vi "FIB MAIN (6400d-132016-w's conflicted copy 2019-02-25).vi"() -> ()   [LabVIEW 2018]
uses:
  <vilib>/userdefined/High Color/IMAQdx.ctl
  STAGE POSITION.ctl
  Original FIB Source/CENTER STIGMATOR.ctl
  FIB EVENTS.ctl
  FIB CAMERA EVENTS.ctl
  <vilib>/vision/driver/IMAQdx.llb/IMAQdx Buffer Number Mode.ctl
  <vilib>/vision/driver/IMAQdx.llb/IMAQdx Camera Control Mode.ctl
  <vilib>/Instr/_visa.llb/VISA Flush IO Buffer Mask.ctl
  <vilib>/Utility/error.llb/whitespace.ctl
  Mikrodaq/HYMOD MAIA/ddd.ctl
  FIB STAGE EVENTS.ctl
  <vilib>/Instr/_visa.llb/VISA Configure Serial Port (Instr).vi
  <vilib>/vision/driver/NI_Vision_Acquisition_Software.lvlib
  <resource>/objmgr/imaqdx.rc
  <vilib>/vision/NI_Vision_Development_Module.lvlib
  <vilib>/Utility/Variable/NI_VariableUtilities.lvlib
panel:
  out "PREVIOUS GUN SETTINGS":T1 {"ION CURRENT" min=0 max=3e-05 step=1e-07; "SUPPRESSOR" min=0 max=30000 step=250; "EXTRACTOR" min=0 max=30000 step=250; "BEAM ENERGY" min=0 max=30000 step=1000}
  out "size(s) 5":i32
  in  "ENABLE APERTURES":bool
  in  "ENABLE ORSAY":bool=TRUE
  in  "ENABLE CAMERA":bool
  out "size(s) 4":i32
  in  "Tab Control 4":enum32{"COMMANDS", "HV RAMPS"}(tab)
  in  "1V ENERGY RAMP":bool
  out "TEST OUTPUT":string
  in  "TEST COMMAND":bool
  in  "TEST COMMAND":string
  out "SERIAL \nRESPONSE":string[](array[string])
  out "WARNING":string
  out "PROCESS":string
  out "PROCESSES":string[](array[string])
  out "BEAM RAMP":dbl[unit][](graph)
  out "EXTRACTOR RAMP":dbl[unit][](graph)
  out "SUPPRESSOR RAMP":dbl[unit][](graph)
  in  "Tab Control 3":T2(tab)
  in  "E&B":T3 {"ELECTRIC FIELD" min=0 max=20 step=0.1 scale=0.0..2.0; "M-FINE" min=0 max=20000 step=100 scale=-0.08..0.08; "M-COARSE" min=0 max=20 step=0.1 scale=0.0..2.0}
  in  "WIEN":bool
  out "CURRENT":dbl[unit] format="%_4g"
  out "VOLTAGE":dbl[unit] format="%_4g"
  out "BEAM VOLTAGE":dbl[unit](graph)
  out "BEAM CURRENT":dbl[unit](graph)
  out "VOLTAGE":dbl[unit] format="%_4g"
  out "CURRENT":dbl[unit] format="%_4g"
  out "EXTRACTOR":dbl[unit](graph)
  out "EXTRACTOR  CURRENT":dbl[unit](graph)
  out "VOLTAGE":dbl[unit] format="%_4g"
  out "CURRENT":dbl[unit] format="%_4g"
  out "SUPPRESSOR VOLTAGE":dbl[unit](graph)
  out "SUPPRESSOR CURRENT":dbl[unit](graph)
  out "CONDENSOR VOLTAGE":dbl[unit](graph)
  out "CONDENSOR CURRENT":dbl[unit](graph)
  out "OBJECTIVE VOLTAGE":dbl[unit](graph)
  out "OBJECTIVE CURRENT":dbl[unit](graph)
  out "HV SUPPLY FEEDBACK 13":dbl[unit](graph)
  out "HV SUPPLY FEEDBACK 12":dbl[unit](graph)
  out "HEAT POWER":cluster{i32[], dbl[unit][]}(graph)
  in  "IGAIN":dbl=0.00039 format="%_3p"
  in  "IOFFSET":dbl format="%_4g"
  in  "VOFFSET":dbl format="%_4g"
  out "CURRENT":dbl[unit] format="%_4g"
  out "VOLTAGE":dbl[unit] format="%_4g"
  in  "VGAIN":dbl=0.00071 format="%_3p"
  in  "OFFSET":dbl
  in  "RPONT":dbl[unit]
  in  "RMES":dbl[unit]
  out "TIMER":u32
  out "size(s)":i32
  out "SUPPRESSOR RAMP":dbl[unit][](array[numeric])
  out "EXTRACTOR RAMP":dbl[unit][](array[numeric])
  out "BEAM RAMP":dbl[unit][](array[numeric])
  in  "MEASURE HV":bool
  out "SERIAL \nRESPONSE 2":string[](array[string])
  out "VISA ERROR":errorcluster
  out "BEAM CURRENT (FC2)":dbl[unit] format="%_4g"
  out "BEAM CURRENT (FC1)":dbl[unit] format="%_4g"
  in  "APERTURE (MASS)":u16(ring)=3 items=["10 um", "20 um", "50 um", "50 um", "100 um", "200 um", "400 um"]
  in  "BRIGHT,CONT,GAMMA":cluster{"B":dbl, "C":dbl, "G":dbl}={"B"=250.0, "C"=67.0, "G"=1.6000000000000005} {"G" format="%_4g"; "C" format="%_4g"; "B" format="%_4g"}
  in  "REFLECTIVITY":bool
  in  "ROTATE VIEW":bool
  in  "ANGLE":sgl format="%.2f"
  in  "IMAGE SYMMETRY":u32(ring)=2 items=["Horizontal", "Vertical", "CENTRAL", "1st Diagonal", "2nd Diagonal"]
  in  "SYMMETRY":bool
  out "FIB CAMERA ERROR":errorcluster
  out "FIB SAMPLE CAMERA":T4="CSIRO-SAMPLE" caption="Session Out"
  out "IMAGE YCENTRE":dbl
  out "IMAGE XCENTRE":dbl
  out "ActualPeakBandwidth":dbl=1000.0
  out "IMAGE YPIXELS":u32=1024
  out "IMAGE XPIXELS":u32=1360
  in  "START SCANNING":bool
  in  "STOP":bool
  out "INTERLOCK STATE":bool
  in  "BEAM ON":bool=TRUE
  in  "BLANKING CONTROL":u16(ring) items=["LOCAL ", "SOURCE", "EXTERNAL"]
  in  "FIB SETUP FILE":path=path "C:/Users/jamie/Desktop/test.tdms"
  in  "SAVE SETUP":bool
  in  "READ & APPLY SETUP":bool
  in  "OBJECT APERTURE":u16(ring)=3 items=["10 um", "20 um", "50 um", "50 um", "100 um", "200 um", "400 um"]
  in  "USER":string="jslaird"
  in  "COMMENT":string
  in  "NAME":string
  out "gamme":bool
  out "Image":T5(plugin-control)
  in  "Tab Control":T6(tab)
  in  "RESET":bool
  in  "INTERLOCK HV":bool
  out "HIGH ENERGY":bool
  in  "SETTINGS DELAY":dbl[unit]=0.2
  in  "dV ENERGY":dbl[unit]=250.0
  in  "dV SUPPRESS":dbl[unit]=50.0
  in  "SHUTDOWN":bool
  in  "FILAMENT":bool
  out "HIGH VOLTAGE SUPPLIES":cluster{dbl[unit], dbl[unit], dbl[unit]}(knob)={0.0, 103.78830891166923, 181.50345045415557} scale format="%#_6p"
  in  "ION GUN":bool
  in  "FILAMENT HEATING":dbl[unit](slide) min=0.0 max=5.0 step=0.1 scale=0.0..5.000000000000001
  in  "ION GUN SETTINGS":T1 {"ION CURRENT" min=0 max=3e-05 step=1e-07; "SUPPRESSOR" min=0 max=30000 step=250; "EXTRACTOR" min=0 max=30000 step=250; "BEAM ENERGY" min=0 max=30000 step=1000}
  in  "dV EXTRACTOR":dbl[unit]=50.0
  in  "MOVE 2 POSITION":T7 {"Z" format="%_4g"; "Y" format="%_4g"; "X" format="%_4g"}
  out "POSITION":T7 {"Z" format="%_4g"; "Y" format="%_4g"; "X" format="%_4g"}
  in  "EXPOSURE":dbl(slide)=106.26827541712952 min=1.0 max=2500.0 step=10.0 scale=5.0..1000.0 scale format="%#_3f"
  out "FIB CAMERA":T5(plugin-control)
  out "IP ADDRESS":string="192.168.1.10"
  in  "CONFIGS":u16(ring) items=["MANUAL", "BEAM FOCUS", "SAMPLE VIEWING"]
  in  "GAIN METHOD":u16(ring)=2 items=["OFF", "ONCE", "CONTINOUS"]
  in  "GAIN":sgl=1.0 min=0 max=31 step=1
  out "CENTRE CAMERA FOV":T8={"Numeric Control"=677, "Numeric Control"=510}
  in  "Tab Control 2":T9(tab)
  out "Yo":dbl format="%_3g"
  out "Xo":dbl format="%_3g"
  in  "STORE OBJECT":bool
  in  "WOBBLER SETTINBGS FOR OBJECT ALIGNMENT":T10={"WOBBLER AMPLITUDE"={0.0, 33.333523, 47.735184}, "WOBBLE"=1} {"WOBBLE" items=["ENERGY", "CONDENSOR", "OBJECTIVE"]; "WOBBLER AMPLITUDE" scale=0.0..100.0}
  in  "OBJ APERTURE ALIGNMENT":T11={"DOWN"=FALSE, "UP"=FALSE, "STEP SIZE"=1, "LEFT"=FALSE, "RIGHT"=FALSE} {"STEP SIZE" items=["1 um", "5 um", "20 um", "50 um", "100 um", "500 um", "2000 um"]}
  in  "TURN ON WOBBLER":bool
  in  "OBJECT APERTURE POSITIONS":cluster{"NAME":string, "Xo":dbl, "Yo":dbl}[](array[cluster])=[{"NAME"="10um", "Xo"=0.0, "Yo"=0.0}, {"NAME"="20um", "Xo"=0.0, "Yo"=0.0}, {"NAME"="50um", "Xo"=0.0, "Yo"=0.0}, {"NAME"="50um", "Xo"=0.0, "Yo"=0.0}, {"NAME"="100um", "Xo"=0.0, "Yo"=0.0}, {"NAME"="200um", "Xo"=0.0, "Yo"=0.0}, {"NAME"="400um", "Xo"=0.0, "Yo"=0.0}] {"Yo" format="%_3g"; "Xo" format="%_3g"}
  in  "MASS APERTURE POSITIONS":cluster{"NAME":string, "Xa":dbl, "Ya":dbl}[](array[cluster])=[{"NAME"="10um", "Xa"=0.0, "Ya"=0.0}, {"NAME"="20um", "Xa"=0.0, "Ya"=0.0}, {"NAME"="50um", "Xa"=0.0, "Ya"=0.0}, {"NAME"="50um", "Xa"=0.0, "Ya"=0.0}, {"NAME"="100um", "Xa"=0.0, "Ya"=0.0}, {"NAME"="200um", "Xa"=0.0, "Ya"=0.0}, {"NAME"="400um", "Xa"=0.0, "Ya"=0.0}] {"Ya" format="%_3g"; "Xa" format="%_3g"}
  in  "MASS APERTURE ALIGNMENT":T11={"DOWN"=FALSE, "UP"=FALSE, "STEP SIZE"=1, "LEFT"=FALSE, "RIGHT"=FALSE} {"STEP SIZE" items=["1 um", "5 um", "20 um", "50 um", "100 um", "500 um", "2000 um"]}
  out "Xa":dbl format="%_3g"
  out "Ya":dbl format="%_3g"
  in  "STORE APERTURE":bool
  out "REFERENCED":bool[](array[boolean])
  out "ON TRARGET":bool[](array[boolean])
  in  "INIT PI":bool
  in  "STAGE AXES":string[](array[string])=["1", "2"]
  out "VELOCITIES":dbl[](array[numeric])
  out "POSITIONS":dbl[](array[numeric]) format="%_5g"
  out "STATUS":bool
  in  "HOME ALL AXES":bool
  in  "AXES MOTIION SETTINGS":dbl[][](array[numeric])=[[1.0, 140.0, 5.0, 350.0, 1200.0, 10000.0, 100.0, 30000.0, 200.0], [2.0, 140.0, 5.0, 350.0, 1200.0, 10000.0, 100.0, 30000.0, 200.0], [3.0, 140.0, 5.0, 0.0, 1200.0, 10000.0, 100.0, 30000.0, 200.0], [4.0, 140.0, 5.0, 0.0, 0.0, 10000.0, 100.0, 30000.0, 200.0]]
  out "NO CONTROLLER":bool
  in  "HOME ON LIMIT":u16(ring) items=["POSITIVE", "NEGATIVE"]
  out "RANGE":dbl[](array[numeric]) format="%_5g"
  in  "STIGMATOR":T12 {"STIG ALIGN"."-Y" min=-100 max=100 step=0.1 scale=-100.0..100.0; "STIG ALIGN"."+Y" min=-100 max=100 step=0.1 scale=-100.0..100.0; "STIG ALIGN"."-X" min=-100 max=100 step=0.1 scale=-100.0..100.0; "STIG ALIGN"."+X" min=-100 max=100 step=0.1 scale=-100.0..100.0; "THETA" format="%_3g"; "OFFY" format="%_3g"; "OFFX" format="%_3g"; "STIG Y" format="%_3g"; "STIG X" format="%_3g"}
  in  "STIGMATOR X & Y":cluster{"X":sgl, "Y":sgl} {"Y" min=0 max=20000 step=100 scale=0.0..1000.0; "X" min=0 max=20 step=0.1 scale=0.0..20.0}
  out "OBJECTIVE":sgl[unit] format="%_4g"
  out "CONDENSOR":sgl[unit] format="%_4g"
  in  "OBJECTIVE":cluster{"COARSE":sgl[unit], "FINE":sgl[unit]} {"FINE" min=0 max=20000 step=100 scale=0.0..1000.0; "COARSE" min=0 max=20000 step=100}
  in  "CONDENSOR":cluster{"COARSE":sgl[unit], "FINE":sgl[unit]} {"FINE" min=0 max=20000 step=100 scale=1.0..1000.0; "COARSE" min=0 max=20000 step=100}
  in  "SCAN CENTRE ON STAGE":T13 {"Zs" format="%_2g"; "Xs" format="%_2g"; "Ys" format="%_2g"}
  in  "STAGE POSITION":T13 {"Zs" format="%_2g"; "Xs" format="%_2g"; "Ys" format="%_2g"}
  in  "SCANNING CLUSTER":T14 {"MAGNIFICATION" scale=-180.0..180.0; "Y-OFFSET" min=0 max=3e-05 step=1e-07; "X-OFFSET" min=0 max=3e-05 step=1e-07; "SCANNING TYPE" items=["EXTERNAL", "ION MILLING"]}
  in  "EXTERNAL SCANNING ROI":T15={"X-AMPLITUDE"=1e-07, "dX"=0.0, "Y-AMPLITUDE"=1e-07, "dY"=0.0} {"Y-AMPLITUDE" min=1e-07 max=0.0005 step=9.999999999999999e-06; "X-AMPLITUDE" min=1e-07 max=0.0005 step=9.999999999999999e-06}
  out "CHAMBER VACUUM":cluster{dbl[unit], dbl[unit]}(knob)={2.179544466940017e-05, 0.00030039245125477424} scale format="%#_2e"
  in  "COLUMN THRESHOLD":dbl[unit]=6.666118421052631e-05
  out "VACUUM STATE":bool
  out "COLUMN VACUUM":dbl[unit](graph)
  out "COLUMN VACUUM":cluster{dbl[unit], dbl[unit]}(knob)={8.118323356328827e-09, 0.00010317996118558537} scale format="%#_1e"
  out "150V GOOD":bool
  in  "CHAMBER THRESHOLD":dbl[unit]
  in  "GATE VALVE":bool=TRUE
  in  "TERMINATION":bool=TRUE
  in  "TERMINATION CHAR":u16(ring)=1 items=["NONE", "CR", "LF", "CR+LF"]
  out "APPEND":string
  out "ORSAY CONNECTED":bool
  in  "STARTUP":T16[](array[typedef])=[enum."OPEN SERIAL CONN TO ORSAY", enum."INITIALISE ORSAY", enum."TURN OFF WOBBLER", enum."VACUUM ", enum."CHECK 150V", enum."BLANKING TOGGLE"]
  out "ORSAY":refnum<visa-resource-name>
  # "EXTRACTOR"
  # "CONDENSOR"
  # "OBJECT\nAPERTURES"
  # "OBJECTIVE"
  # "FILAMENT SHOULD BE ON PRIOR TO GUN !"
  # "E"
  # "C"
  # "O"
  # "AXIS               P                        I                      D                      L                  LOW-VEL    LOW-ACC      HI-VEL          HI-ACC"
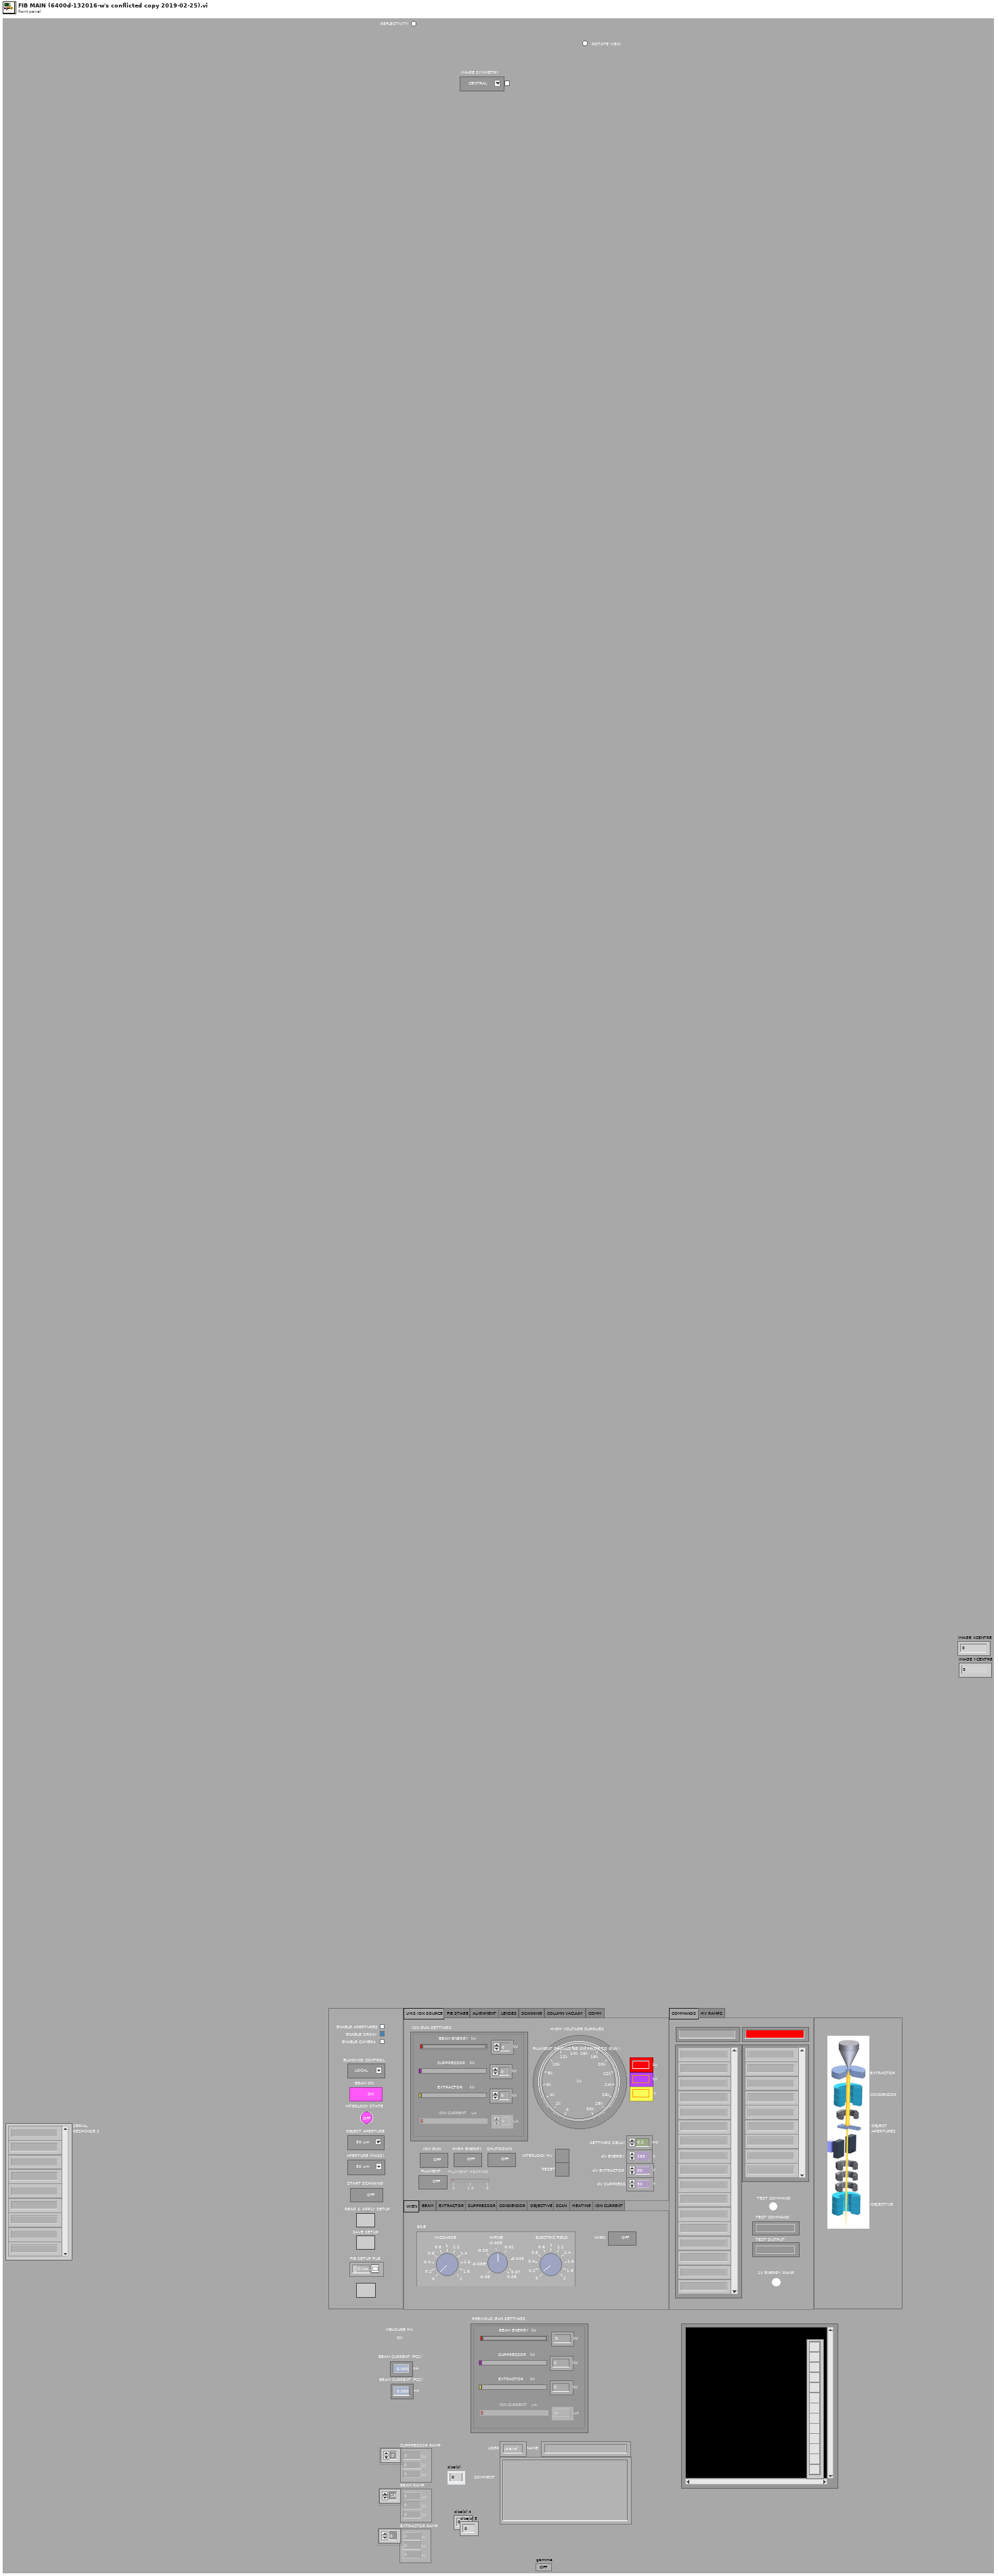
[diagram p1: front panel]
types:
  T1 = cluster{"BEAM ENERGY":sgl[unit], "SUPPRESSOR":sgl[unit], "EXTRACTOR":sgl[unit], "ION CURRENT":sgl[unit]}
  T2 = enum32{"WIEN", "BEAM", "EXTRACTOR", "SUPPRESSOR", "CONDENSOR", "OBJECTIVE", "SCAN", "HEATING", "ION CURRENT"}
  T3 = cluster{"M-COARSE":sgl, "M-FINE":sgl, "ELECTRIC FIELD":sgl}
  T4 = typedef "IMAQdx.ctl" = refnum<k21>
  T5 = typedef "IMAQ Image.ctl" = refnum<image>
  T6 = enum32{"LMIS ION SOURCE", "FIB STAGE", "ALIGNMENT", "LENSES", "SCANNING", "COLUMN VACUUM", "COMM"}
  T7 = typedef "STAGE POSITION.ctl" = cluster{"X":dbl[unit], "Y":dbl[unit], "Z":dbl[unit]}
  T8 = cluster{"Numeric Control":i32, "Numeric Control":i32}
  T9 = enum32{"OBJECTS", "MASS APERTURES", "MOTORS", "CENTRE STIGMATOR"}
  T10 = cluster{"WOBBLER AMPLITUDE":cluster{sgl, sgl, sgl}, "WOBBLE":u16}
  T11 = cluster{"DOWN":bool, "UP":bool, "STEP SIZE":u16, "LEFT":bool, "RIGHT":bool}
  T12 = typedef "CENTER STIGMATOR.ctl" = cluster{"STIG ALIGN":cluster{"+X":sgl, "-X":sgl, "+Y":sgl, "-Y":sgl}, "STIG X":dbl, "OFFX":dbl, "STIG Y":dbl, "OFFY":dbl, "THETA":dbl}
  T13 = cluster{"Xs":dbl[unit], "Ys":dbl[unit], "Zs":dbl[unit]}
  T14 = cluster{"SCANNING TYPE":u16, "X-OFFSET":sgl[unit], "Y-OFFSET":sgl[unit], "ROTATION":dbl[unit], "MAGNIFICATION":dbl}
  T15 = cluster{"X-AMPLITUDE":dbl[unit], "dX":dbl[unit], "Y-AMPLITUDE":dbl[unit], "dY":dbl[unit]}
  T16 = typedef "FIB EVENTS.ctl" = enum16{"LOOP", "OPEN SERIAL CONN TO ORSAY", "INITIALISE ORSAY", "READ SETTINGS", "SAVE SETTINGS", "OBJECTIVE LENS", "CONDENSOR LENS", "BLANKING TOGGLE", "TURN ON HEATER", "TURN OFF WOBBLER", "MEASURE HEATER OUTPUT", "TOGGLE GATE VALVE", "SCANNING CONTROLS", "TURN ON BEAM HV", "ENERGY RAMP CYCLE", "TURN ON SUPPRESSOR", "TURN ON EXTRACTOR", "TURN ON WIEN FILTER", "SET ENERGY RANGE", "MEASURE HV SUPPLY VOLTAGES", "SHUTDOWN ION SOURCE", "RESET TYPE II", "PROBE CURRENT FC#1", "PROBE CURRENT FC#2", "VACUUM ", "CHECK 150V", "INITIALISE PI MOTORS", "SET STIGMATOR", "SET WOBBLER FOR OBJECT", "SET OBJ & AP STAGE VELOCITIES", "READ APERTURE POSITIONS", "HOME OBJ & AP STAGES", "DEFINE NEW OBJ", "MOVE OBJ STAGES", "DEFINE NEW APERTURE", "MOVE APERTURE STAGES", "STOP SYSTEM", "TEST COMMANDS"}
  T17 = typedef "FIB CAMERA EVENTS.ctl" = enum16{"INIT VIDEO", "CAMERA GAIN", "CAMERA EXPOSURE", "LOOP"}
  T18 = enum8{"Enabled", "Disabled", "Disabled and Grayed Out"}
  T19 = cluster{"BEAM ENERGY":sgl[unit], "EXTRACTOR":sgl[unit], "SUPPRESSOR":sgl[unit], "ION CURRENT":sgl[unit]}
  T20 = typedef "FIB STAGE EVENTS.ctl" = enum16{"LOOP", "INIT STAGE CONTROLLER", "SEND COMMAND TO CONTROLLER", "HOME X", "HOME Y", "HOME Z", "ABORT ALL AXES", "GOTO MARKER", "ZERO XYZ", "READ XYZ POSITIONS", "GOTO XYZ POSITION", "STOP", "JOG XYZ", "WAIT FOR MOVE COMPLETE"}
  T21 = cluster{"BEAM":dbl[unit], "SUPPRESSOR":dbl[unit], "EXTRACTOR":dbl[unit]}
  T22 = typedef "ddd.ctl" = string[]
  T23 = enum16{"open", "open or create", "create or replace", "create", "open (read-only)"}
  T24 = typedef "VISA Flush IO Buffer Mask.ctl" = u16
  T25 = cluster{dbl[unit], "CHAMBER THRESHOLD":dbl[unit]}
  T26 = typedef "whitespace.ctl" = u16
  T27 = typedef "NI_Vision_Acquisition_Software.lvlib/IMAQdx Buffer Number Mode.ctl" = enum32{"Next", "Last", "Buffer Number", "Every", "Last New"}
  T28 = typedef "NI_Vision_Acquisition_Software.lvlib/IMAQdx Camera Control Mode.ctl" = enum32{"Controller", "Listener"}
  T29 = typedef "Image Type" = u32
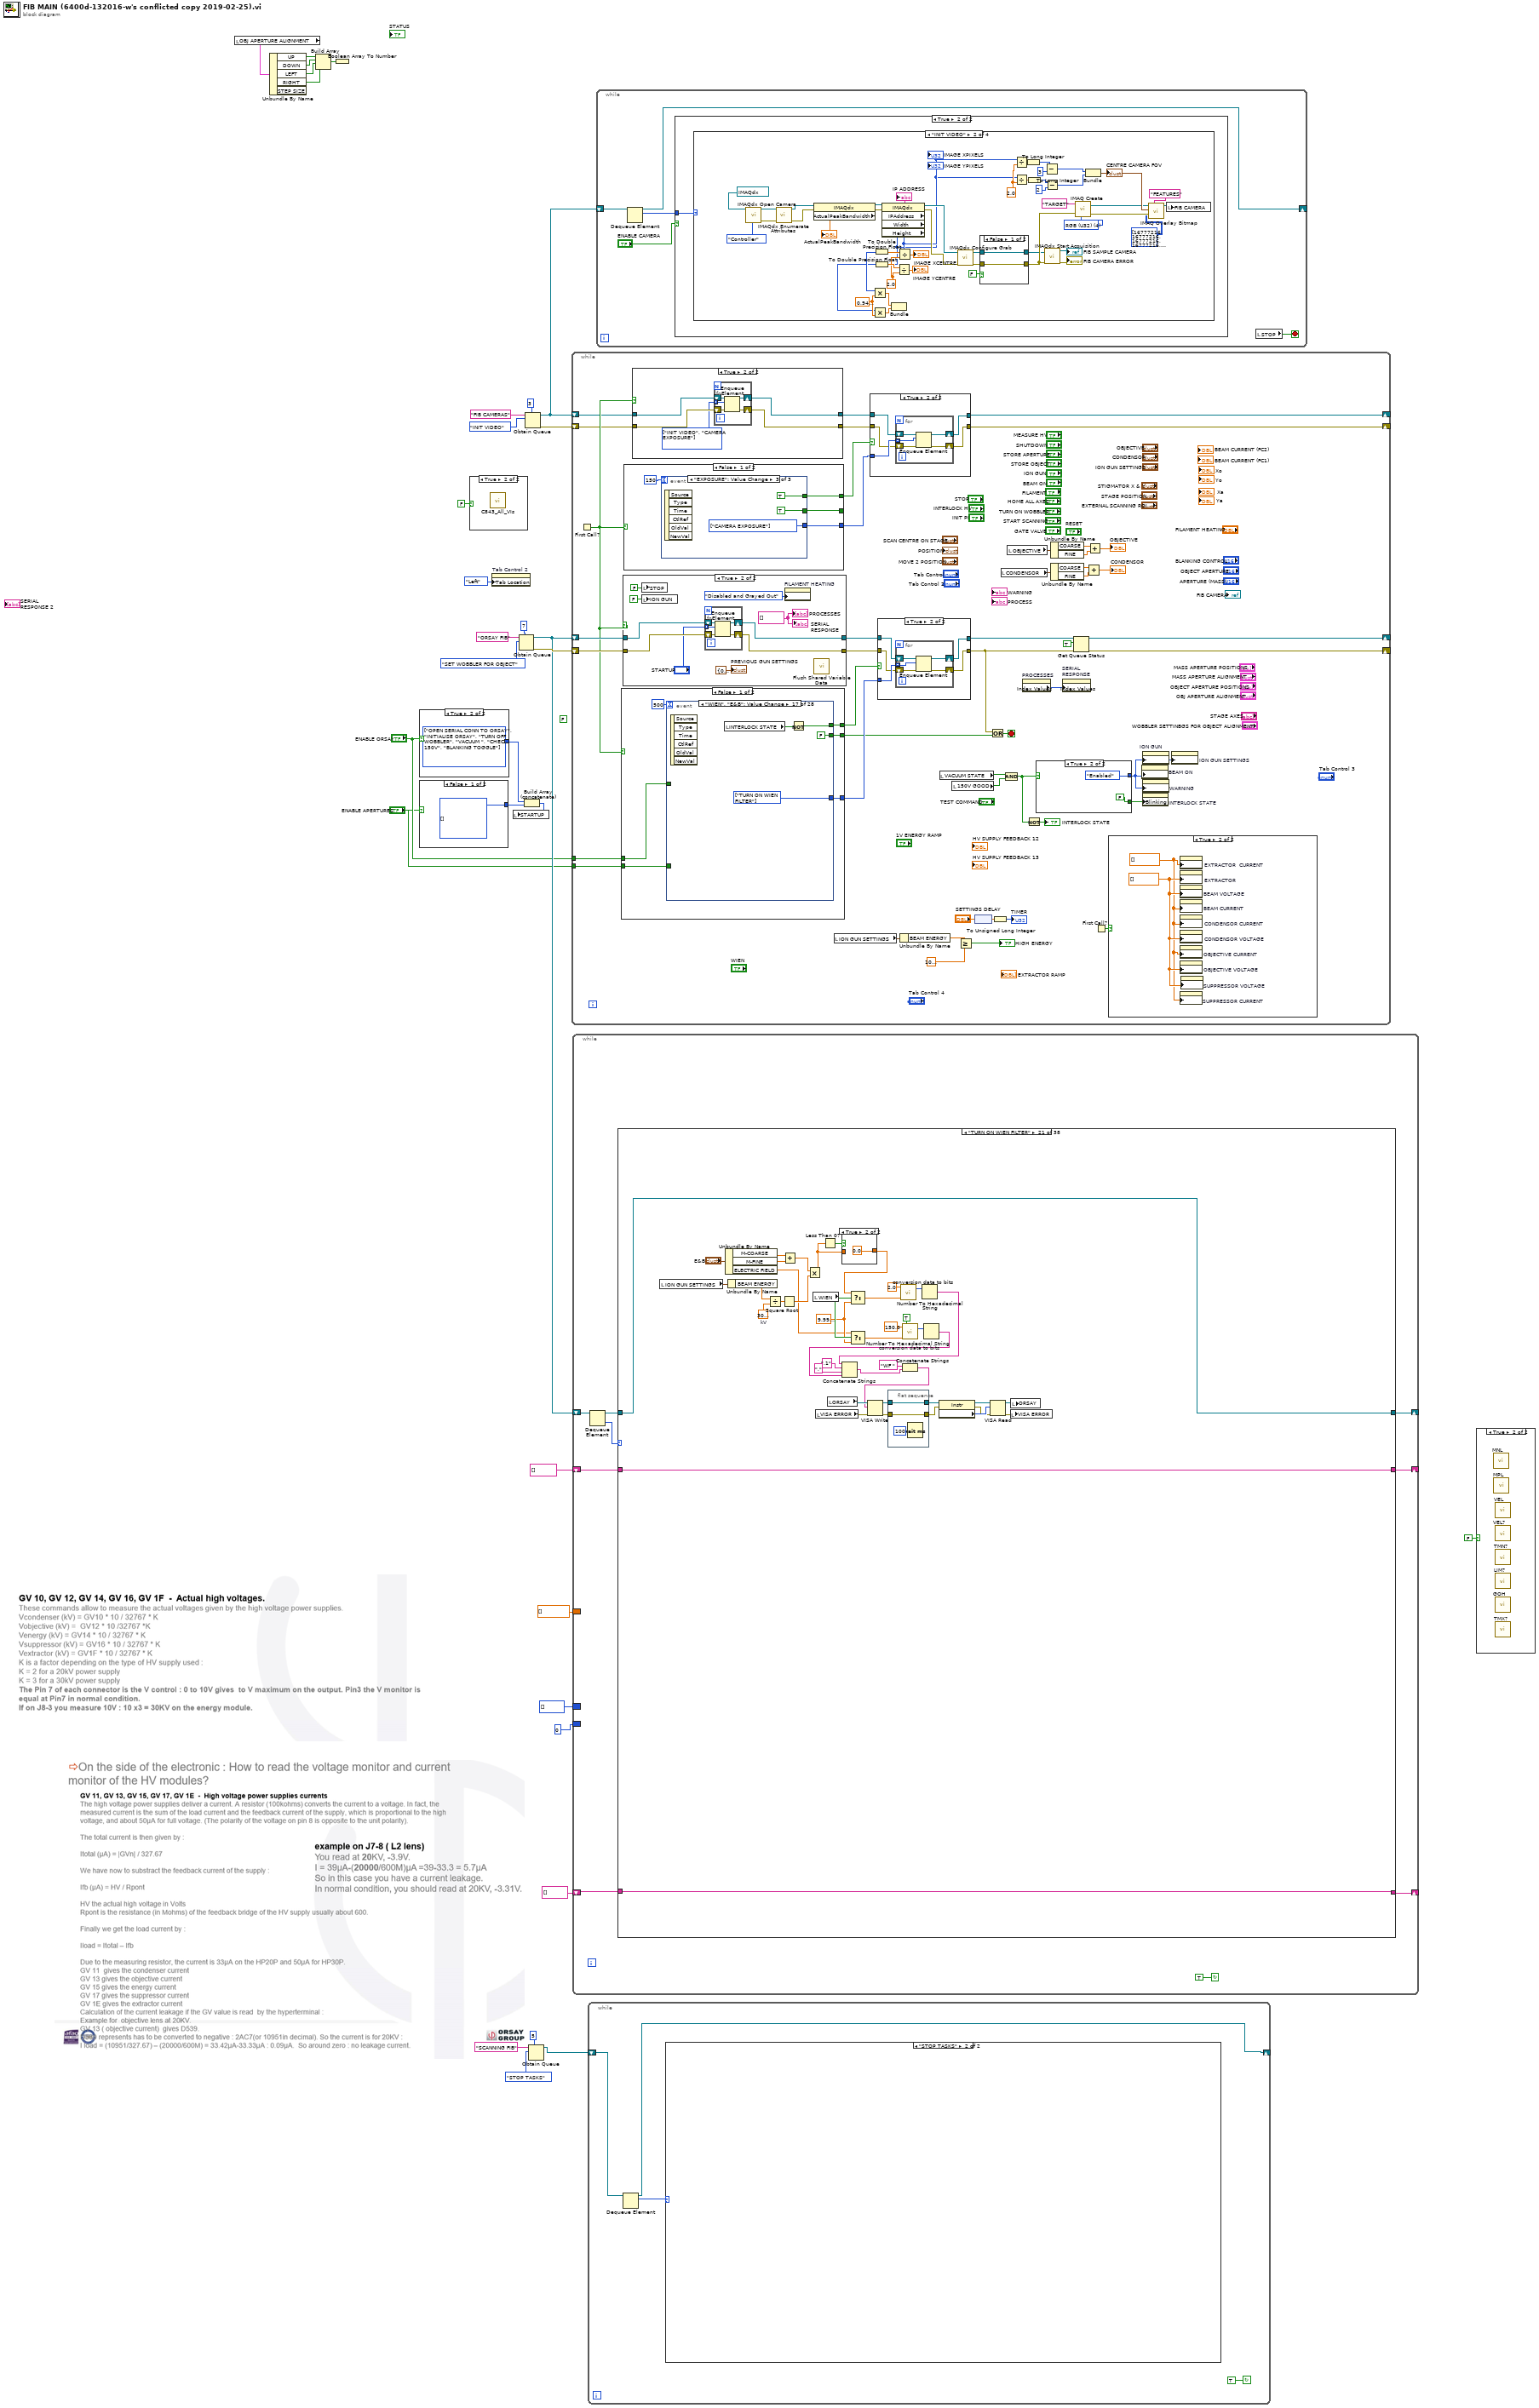
[diagram p0: block diagram]
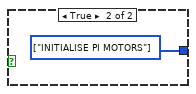
[diagram p2: hidden frame]
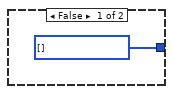
[diagram p3: hidden frame]
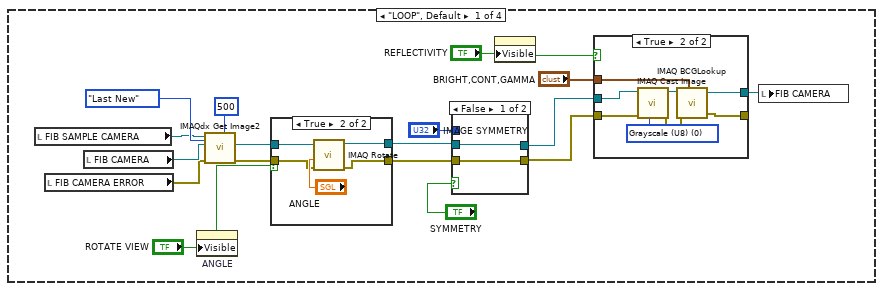
[diagram p8: hidden frame]
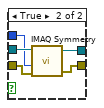
[diagram p11: hidden frame]
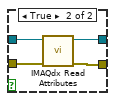
[diagram p12: hidden frame]
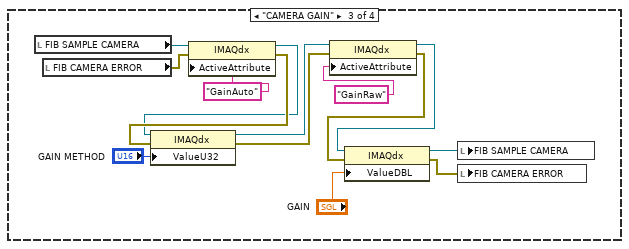
[diagram p13: hidden frame]
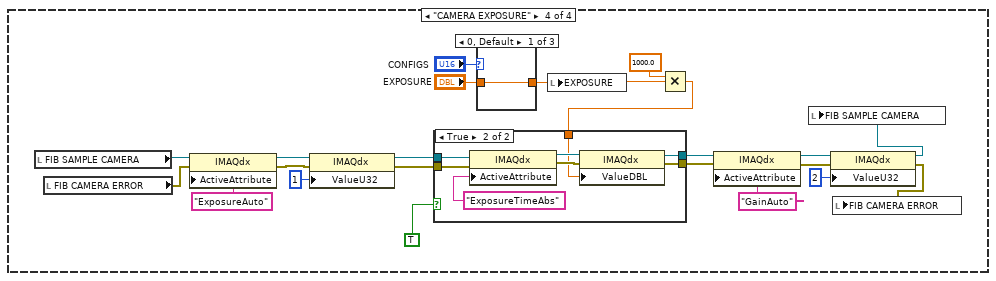
[diagram p14: hidden frame]
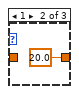
[diagram p16: hidden frame]
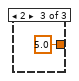
[diagram p17: hidden frame]
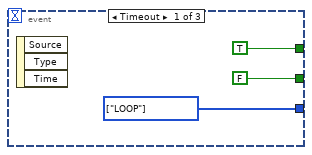
[diagram p20: hidden frame]
diagram:
  (unwired) FALSE ("ION GUN")
  n1 = local read "OBJ APERTURE ALIGNMENT"() -> (w20:T11)
  n2 = Unbundle By Name(w20) -> ("UP"=w21:bool, "DOWN"=w22:bool, "LEFT"=w23:bool, "RIGHT"=w24:bool)  [unwired: 1 out]
  n3 = Build Array(w21, w22, w23, w24) -> (w25:bool[])
  n4 = Boolean Array To Number(Boolean array=w25) -> ()  [unwired: 1 out]
  n5 = case shown="True" "ENABLE ORSAY" {
    tunnel: [w34 w35] -> w8
    frame False {
      w34 = T16[] [] items=["LOOP", "OPEN SERIAL CONN TO ORSAY", "INITIALISE ORSAY", "READ SETTINGS", "SAVE SETTINGS", "OBJECTIVE LENS", "CONDENSOR LENS", "BLANKING TOGGLE", "TURN ON HEATER", "TURN OFF WOBBLER", "MEASURE HEATER OUTPUT", "TOGGLE GATE VALVE", "SCANNING CONTROLS", "TURN ON BEAM HV", "ENERGY RAMP CYCLE", "TURN ON SUPPRESSOR", "TURN ON EXTRACTOR", "TURN ON WIEN FILTER", "SET ENERGY RANGE", "MEASURE HV SUPPLY VOLTAGES", "SHUTDOWN ION SOURCE", "RESET TYPE II", "PROBE CURRENT FC#1", "PROBE CURRENT FC#2", "VACUUM ", "CHECK 150V", "INITIALISE PI MOTORS", "SET STIGMATOR", "SET WOBBLER FOR OBJECT", "SET OBJ & AP STAGE VELOCITIES", "READ APERTURE POSITIONS", "HOME OBJ & AP STAGES", "DEFINE NEW OBJ", "MOVE OBJ STAGES", "DEFINE NEW APERTURE", "MOVE APERTURE STAGES", "STOP SYSTEM", "TEST COMMANDS"] ("STARTUP")
    }
    frame True {
      w35 = T16[] [enum."OPEN SERIAL CONN TO ORSAY", enum."INITIALISE ORSAY", enum."TURN OFF WOBBLER", enum."VACUUM ", enum."CHECK 150V", enum."BLANKING TOGGLE"] items=["LOOP", "OPEN SERIAL CONN TO ORSAY", "INITIALISE ORSAY", "READ SETTINGS", "SAVE SETTINGS", "OBJECTIVE LENS", "CONDENSOR LENS", "BLANKING TOGGLE", "TURN ON HEATER", "TURN OFF WOBBLER", "MEASURE HEATER OUTPUT", "TOGGLE GATE VALVE", "SCANNING CONTROLS", "TURN ON BEAM HV", "ENERGY RAMP CYCLE", "TURN ON SUPPRESSOR", "TURN ON EXTRACTOR", "TURN ON WIEN FILTER", "SET ENERGY RANGE", "MEASURE HV SUPPLY VOLTAGES", "SHUTDOWN ION SOURCE", "RESET TYPE II", "PROBE CURRENT FC#1", "PROBE CURRENT FC#2", "VACUUM ", "CHECK 150V", "INITIALISE PI MOTORS", "SET STIGMATOR", "SET WOBBLER FOR OBJECT", "SET OBJ & AP STAGE VELOCITIES", "READ APERTURE POSITIONS", "HOME OBJ & AP STAGES", "DEFINE NEW OBJ", "MOVE OBJ STAGES", "DEFINE NEW APERTURE", "MOVE APERTURE STAGES", "STOP SYSTEM", "TEST COMMANDS"] ("STARTUP")
    }
  }
  n6 = case shown="False" "ENABLE APERTURES" {
    tunnel: [w36 w37] -> w7
    frame False {
      w36 = T16[] [] items=["LOOP", "OPEN SERIAL CONN TO ORSAY", "INITIALISE ORSAY", "READ SETTINGS", "SAVE SETTINGS", "OBJECTIVE LENS", "CONDENSOR LENS", "BLANKING TOGGLE", "TURN ON HEATER", "TURN OFF WOBBLER", "MEASURE HEATER OUTPUT", "TOGGLE GATE VALVE", "SCANNING CONTROLS", "TURN ON BEAM HV", "ENERGY RAMP CYCLE", "TURN ON SUPPRESSOR", "TURN ON EXTRACTOR", "TURN ON WIEN FILTER", "SET ENERGY RANGE", "MEASURE HV SUPPLY VOLTAGES", "SHUTDOWN ION SOURCE", "RESET TYPE II", "PROBE CURRENT FC#1", "PROBE CURRENT FC#2", "VACUUM ", "CHECK 150V", "INITIALISE PI MOTORS", "SET STIGMATOR", "SET WOBBLER FOR OBJECT", "SET OBJ & AP STAGE VELOCITIES", "READ APERTURE POSITIONS", "HOME OBJ & AP STAGES", "DEFINE NEW OBJ", "MOVE OBJ STAGES", "DEFINE NEW APERTURE", "MOVE APERTURE STAGES", "STOP SYSTEM", "TEST COMMANDS"] ("STARTUP")
    }
    frame True {
      w37 = T16[] [enum."INITIALISE PI MOTORS"] items=["LOOP", "OPEN SERIAL CONN TO ORSAY", "INITIALISE ORSAY", "READ SETTINGS", "SAVE SETTINGS", "OBJECTIVE LENS", "CONDENSOR LENS", "BLANKING TOGGLE", "TURN ON HEATER", "TURN OFF WOBBLER", "MEASURE HEATER OUTPUT", "TOGGLE GATE VALVE", "SCANNING CONTROLS", "TURN ON BEAM HV", "ENERGY RAMP CYCLE", "TURN ON SUPPRESSOR", "TURN ON EXTRACTOR", "TURN ON WIEN FILTER", "SET ENERGY RANGE", "MEASURE HV SUPPLY VOLTAGES", "SHUTDOWN ION SOURCE", "RESET TYPE II", "PROBE CURRENT FC#1", "PROBE CURRENT FC#2", "VACUUM ", "CHECK 150V", "INITIALISE PI MOTORS", "SET STIGMATOR", "SET WOBBLER FOR OBJECT", "SET OBJ & AP STAGE VELOCITIES", "READ APERTURE POSITIONS", "HOME OBJ & AP STAGES", "DEFINE NEW OBJ", "MOVE OBJ STAGES", "DEFINE NEW APERTURE", "MOVE APERTURE STAGES", "STOP SYSTEM", "TEST COMMANDS"] ("STARTUP")
    }
  }
  n7 = case shown="True" FALSE {
    frame False {
    }
    frame True {
      n8 = call "C843_All_VIs.vi"() -> ()  [unwired: 1 in]
    }
  }
  n9 = property on="Tab Control 2" class="TabCtl (strict)"("Tab Location"=enum32{"Top", "Bottom", "Left", "Right"}."Left") -> ()  [unwired: 2 in, 2 out]
  n10 = Obtain Queue(max queue size (-1, unlimited)=7, name (unnamed)="ORSAY FIB", element data type=FIB_EVENTS."SET WOBBLER FOR OBJECT" ("Enum")) -> (queue out=w10:refnum<queue>, error out=w31:errorcluster)  [unwired: 2 in, 1 out]
  n11 = Build Array (concatenate)(w8, w7) -> (w6:T16[])
  n12 = local write "STARTUP"(w6) -> ()
  n13 = Obtain Queue(max queue size (-1, unlimited)=3, name (unnamed)="FIB CAMERAS", element data type=FIB_CAMERA_EVENTS."INIT VIDEO") -> (queue out=w26:refnum<queue>, error out=w27:errorcluster)  [unwired: 2 in, 1 out]
  n14 = Obtain Queue(max queue size (-1, unlimited)=5, name (unnamed)="SCANNING FIB", element data type=enum16{"INIT DAQ", "STOP TASKS"}."STOP TASKS") -> (queue out=w14:refnum<queue>)  [unwired: 2 in, 2 out]
  n15 = while {
    shift-right: [w76] -> _
    shift-left: w10 -> [w84]
    shift-right: [w73] -> _
    shift-left: w31 -> [w83]
    shift-right: [w62] -> _
    shift-left: w26 -> [w68]
    shift-right: [w61] -> _
    shift-left: w27 -> [w67]
    tunnel: "ENABLE ORSAY" -> [w39]
    tunnel: "ENABLE APERTURES" -> [w38]
    stop <- w45 stop-if-true
    n16 = First Call?() -> (First Call?: T/F=w69:bool)
    n17 = case shown="False" w69 {
      tunnel: [w135 FALSE] -> w81
      tunnel: [w134 w249] -> w80
      tunnel: [w133 FALSE] -> w77
      tunnel: w39 -> [w132 _]
      tunnel: w38 -> [w131 _]
      frame False {
        n18 = event shown="[16] \"WIEN\", \"E&B\": Value Change" {
          selector: _ -> [_ _ _ _ _ _ _ _ _ _ _ _ _ _ _ _ _ _ _ _ _ _ _ _ _ _ _ _]
          dyn-events: _ -> [_ _ _ _ _ _ _ _ _ _ _ _ _ _ _ _ _ _ _ _ _ _ _ _ _ _ _ _]
          timeout: 500 -> [_ _ _ _ _ _ _ _ _ _ _ _ _ _ _ _ _ _ _ _ _ _ _ _ _ _ _ _]
          tunnel: [TRUE TRUE ("VACUUM STATE") TRUE ("VACUUM STATE") TRUE ("VACUUM STATE") w159 w161 w167 w171 w178 w185 TRUE ("VACUUM STATE") TRUE ("VACUUM STATE") TRUE ("VACUUM STATE") w199 TRUE ("VACUUM STATE") w204 w210 _ TRUE ("VACUUM STATE") w216 w220 w224 w228 TRUE w234 TRUE ("VACUUM STATE") w241 TRUE ("VACUUM STATE")] -> w135
          tunnel: [FALSE FALSE FALSE FALSE FALSE FALSE FALSE FALSE FALSE FALSE FALSE FALSE FALSE FALSE FALSE FALSE FALSE _ FALSE FALSE FALSE FALSE FALSE FALSE FALSE FALSE FALSE FALSE] -> w133
          tunnel: [w140 w150 w151 w156 w157 w165 w168 w174 w181 w183 w188 w191 w194 w197 w203 w207 w208 w212 w213 w219 w223 w227 w230 w233 w235 w237 w240 w243] -> w134
          tunnel: w132 -> [w138 _ _ _ _ _ _ _ _ _ _ _ _ _ _ _ _ _ _ _ _ _ _ _ _ _ _ _]
          tunnel: w131 -> [w137 _ _ _ _ _ _ _ _ _ _ _ _ _ _ _ _ _ _ _ _ _ _ _ _ _ _ _]
          event Timeout {
            n19 = event-data() -> ()  [unwired: 1 in, 3 out]
            n20 = case shown="True" w137 {
              tunnel: [w144 w145] -> w139
              frame False {
                w144 = T16[] [] items=["LOOP", "OPEN SERIAL CONN TO ORSAY", "INITIALISE ORSAY", "READ SETTINGS", "SAVE SETTINGS", "OBJECTIVE LENS", "CONDENSOR LENS", "BLANKING TOGGLE", "TURN ON HEATER", "TURN OFF WOBBLER", "MEASURE HEATER OUTPUT", "TOGGLE GATE VALVE", "SCANNING CONTROLS", "TURN ON BEAM HV", "ENERGY RAMP CYCLE", "TURN ON SUPPRESSOR", "TURN ON EXTRACTOR", "TURN ON WIEN FILTER", "SET ENERGY RANGE", "MEASURE HV SUPPLY VOLTAGES", "SHUTDOWN ION SOURCE", "RESET TYPE II", "PROBE CURRENT FC#1", "PROBE CURRENT FC#2", "VACUUM ", "CHECK 150V", "INITIALISE PI MOTORS", "SET STIGMATOR", "SET WOBBLER FOR OBJECT", "SET OBJ & AP STAGE VELOCITIES", "READ APERTURE POSITIONS", "HOME OBJ & AP STAGES", "DEFINE NEW OBJ", "MOVE OBJ STAGES", "DEFINE NEW APERTURE", "MOVE APERTURE STAGES", "STOP SYSTEM", "TEST COMMANDS"]
              }
              frame True {
                w145 = T16[] [enum."READ APERTURE POSITIONS"] items=["LOOP", "OPEN SERIAL CONN TO ORSAY", "INITIALISE ORSAY", "READ SETTINGS", "SAVE SETTINGS", "OBJECTIVE LENS", "CONDENSOR LENS", "BLANKING TOGGLE", "TURN ON HEATER", "TURN OFF WOBBLER", "MEASURE HEATER OUTPUT", "TOGGLE GATE VALVE", "SCANNING CONTROLS", "TURN ON BEAM HV", "ENERGY RAMP CYCLE", "TURN ON SUPPRESSOR", "TURN ON EXTRACTOR", "TURN ON WIEN FILTER", "SET ENERGY RANGE", "MEASURE HV SUPPLY VOLTAGES", "SHUTDOWN ION SOURCE", "RESET TYPE II", "PROBE CURRENT FC#1", "PROBE CURRENT FC#2", "VACUUM ", "CHECK 150V", "INITIALISE PI MOTORS", "SET STIGMATOR", "SET WOBBLER FOR OBJECT", "SET OBJ & AP STAGE VELOCITIES", "READ APERTURE POSITIONS", "HOME OBJ & AP STAGES", "DEFINE NEW OBJ", "MOVE OBJ STAGES", "DEFINE NEW APERTURE", "MOVE APERTURE STAGES", "STOP SYSTEM", "TEST COMMANDS"]
              }
            }
            n21 = case shown="True" w138 {
              tunnel: [w146 w147] -> w141
              frame False {
                w146 = T16[] [] items=["LOOP", "OPEN SERIAL CONN TO ORSAY", "INITIALISE ORSAY", "READ SETTINGS", "SAVE SETTINGS", "OBJECTIVE LENS", "CONDENSOR LENS", "BLANKING TOGGLE", "TURN ON HEATER", "TURN OFF WOBBLER", "MEASURE HEATER OUTPUT", "TOGGLE GATE VALVE", "SCANNING CONTROLS", "TURN ON BEAM HV", "ENERGY RAMP CYCLE", "TURN ON SUPPRESSOR", "TURN ON EXTRACTOR", "TURN ON WIEN FILTER", "SET ENERGY RANGE", "MEASURE HV SUPPLY VOLTAGES", "SHUTDOWN ION SOURCE", "RESET TYPE II", "PROBE CURRENT FC#1", "PROBE CURRENT FC#2", "VACUUM ", "CHECK 150V", "INITIALISE PI MOTORS", "SET STIGMATOR", "SET WOBBLER FOR OBJECT", "SET OBJ & AP STAGE VELOCITIES", "READ APERTURE POSITIONS", "HOME OBJ & AP STAGES", "DEFINE NEW OBJ", "MOVE OBJ STAGES", "DEFINE NEW APERTURE", "MOVE APERTURE STAGES", "STOP SYSTEM", "TEST COMMANDS"]
              }
              frame True {
                w147 = T16[] [enum."MEASURE HV SUPPLY VOLTAGES", enum."MEASURE HEATER OUTPUT", enum."CHECK 150V", enum."LOOP"] items=["LOOP", "OPEN SERIAL CONN TO ORSAY", "INITIALISE ORSAY", "READ SETTINGS", "SAVE SETTINGS", "OBJECTIVE LENS", "CONDENSOR LENS", "BLANKING TOGGLE", "TURN ON HEATER", "TURN OFF WOBBLER", "MEASURE HEATER OUTPUT", "TOGGLE GATE VALVE", "SCANNING CONTROLS", "TURN ON BEAM HV", "ENERGY RAMP CYCLE", "TURN ON SUPPRESSOR", "TURN ON EXTRACTOR", "TURN ON WIEN FILTER", "SET ENERGY RANGE", "MEASURE HV SUPPLY VOLTAGES", "SHUTDOWN ION SOURCE", "RESET TYPE II", "PROBE CURRENT FC#1", "PROBE CURRENT FC#2", "VACUUM ", "CHECK 150V", "INITIALISE PI MOTORS", "SET STIGMATOR", "SET WOBBLER FOR OBJECT", "SET OBJ & AP STAGE VELOCITIES", "READ APERTURE POSITIONS", "HOME OBJ & AP STAGES", "DEFINE NEW OBJ", "MOVE OBJ STAGES", "DEFINE NEW APERTURE", "MOVE APERTURE STAGES", "STOP SYSTEM", "TEST COMMANDS"]
              }
            }
            n22 = Build Array (concatenate)(w141, w139) -> (w140:T16[])
          }
          event "1V ENERGY RAMP": Mouse Down {
            w150 = T16[] [enum."ENERGY RAMP CYCLE"] items=["LOOP", "OPEN SERIAL CONN TO ORSAY", "INITIALISE ORSAY", "READ SETTINGS", "SAVE SETTINGS", "OBJECTIVE LENS", "CONDENSOR LENS", "BLANKING TOGGLE", "TURN ON HEATER", "TURN OFF WOBBLER", "MEASURE HEATER OUTPUT", "TOGGLE GATE VALVE", "SCANNING CONTROLS", "TURN ON BEAM HV", "ENERGY RAMP CYCLE", "TURN ON SUPPRESSOR", "TURN ON EXTRACTOR", "TURN ON WIEN FILTER", "SET ENERGY RANGE", "MEASURE HV SUPPLY VOLTAGES", "SHUTDOWN ION SOURCE", "RESET TYPE II", "PROBE CURRENT FC#1", "PROBE CURRENT FC#2", "VACUUM ", "CHECK 150V", "INITIALISE PI MOTORS", "SET STIGMATOR", "SET WOBBLER FOR OBJECT", "SET OBJ & AP STAGE VELOCITIES", "READ APERTURE POSITIONS", "HOME OBJ & AP STAGES", "DEFINE NEW OBJ", "MOVE OBJ STAGES", "DEFINE NEW APERTURE", "MOVE APERTURE STAGES", "STOP SYSTEM", "TEST COMMANDS"]
            n23 = event-data() -> ()  [unwired: 1 in, 8 out]
          }
          event "RESET": Mouse Down {
            w151 = T16[] [enum."INITIALISE ORSAY"] items=["LOOP", "OPEN SERIAL CONN TO ORSAY", "INITIALISE ORSAY", "READ SETTINGS", "SAVE SETTINGS", "OBJECTIVE LENS", "CONDENSOR LENS", "BLANKING TOGGLE", "TURN ON HEATER", "TURN OFF WOBBLER", "MEASURE HEATER OUTPUT", "TOGGLE GATE VALVE", "SCANNING CONTROLS", "TURN ON BEAM HV", "ENERGY RAMP CYCLE", "TURN ON SUPPRESSOR", "TURN ON EXTRACTOR", "TURN ON WIEN FILTER", "SET ENERGY RANGE", "MEASURE HV SUPPLY VOLTAGES", "SHUTDOWN ION SOURCE", "RESET TYPE II", "PROBE CURRENT FC#1", "PROBE CURRENT FC#2", "VACUUM ", "CHECK 150V", "INITIALISE PI MOTORS", "SET STIGMATOR", "SET WOBBLER FOR OBJECT", "SET OBJ & AP STAGE VELOCITIES", "READ APERTURE POSITIONS", "HOME OBJ & AP STAGES", "DEFINE NEW OBJ", "MOVE OBJ STAGES", "DEFINE NEW APERTURE", "MOVE APERTURE STAGES", "STOP SYSTEM", "TEST COMMANDS"]
            n24 = event-data() -> ()  [unwired: 1 in, 8 out]
          }
          event "MEASURE HV": Mouse Down {
            w156 = T16[] [enum."MEASURE HV SUPPLY VOLTAGES"] items=["LOOP", "OPEN SERIAL CONN TO ORSAY", "INITIALISE ORSAY", "READ SETTINGS", "SAVE SETTINGS", "OBJECTIVE LENS", "CONDENSOR LENS", "BLANKING TOGGLE", "TURN ON HEATER", "TURN OFF WOBBLER", "MEASURE HEATER OUTPUT", "TOGGLE GATE VALVE", "SCANNING CONTROLS", "TURN ON BEAM HV", "ENERGY RAMP CYCLE", "TURN ON SUPPRESSOR", "TURN ON EXTRACTOR", "TURN ON WIEN FILTER", "SET ENERGY RANGE", "MEASURE HV SUPPLY VOLTAGES", "SHUTDOWN ION SOURCE", "RESET TYPE II", "PROBE CURRENT FC#1", "PROBE CURRENT FC#2", "VACUUM ", "CHECK 150V", "INITIALISE PI MOTORS", "SET STIGMATOR", "SET WOBBLER FOR OBJECT", "SET OBJ & AP STAGE VELOCITIES", "READ APERTURE POSITIONS", "HOME OBJ & AP STAGES", "DEFINE NEW OBJ", "MOVE OBJ STAGES", "DEFINE NEW APERTURE", "MOVE APERTURE STAGES", "STOP SYSTEM", "TEST COMMANDS"]
            n25 = event-data() -> ()  [unwired: 1 in, 8 out]
          }
          event "GATE VALVE": Mouse Down {
            w157 = T16[] [enum."TOGGLE GATE VALVE"] items=["LOOP", "OPEN SERIAL CONN TO ORSAY", "INITIALISE ORSAY", "READ SETTINGS", "SAVE SETTINGS", "OBJECTIVE LENS", "CONDENSOR LENS", "BLANKING TOGGLE", "TURN ON HEATER", "TURN OFF WOBBLER", "MEASURE HEATER OUTPUT", "TOGGLE GATE VALVE", "SCANNING CONTROLS", "TURN ON BEAM HV", "ENERGY RAMP CYCLE", "TURN ON SUPPRESSOR", "TURN ON EXTRACTOR", "TURN ON WIEN FILTER", "SET ENERGY RANGE", "MEASURE HV SUPPLY VOLTAGES", "SHUTDOWN ION SOURCE", "RESET TYPE II", "PROBE CURRENT FC#1", "PROBE CURRENT FC#2", "VACUUM ", "CHECK 150V", "INITIALISE PI MOTORS", "SET STIGMATOR", "SET WOBBLER FOR OBJECT", "SET OBJ & AP STAGE VELOCITIES", "READ APERTURE POSITIONS", "HOME OBJ & AP STAGES", "DEFINE NEW OBJ", "MOVE OBJ STAGES", "DEFINE NEW APERTURE", "MOVE APERTURE STAGES", "STOP SYSTEM", "TEST COMMANDS"]
            n26 = event-data() -> ()  [unwired: 1 in, 8 out]
            n27 = local read "INTERLOCK STATE"() -> (w160:bool)
            n28 = Not(x=w160) -> (.not. x?=w159:bool)
          }
          event "ION GUN": Value Change {
            w165 = T16[] [enum."SET ENERGY RANGE", enum."TURN ON BEAM HV", enum."TURN ON SUPPRESSOR", enum."TURN ON EXTRACTOR"] items=["LOOP", "OPEN SERIAL CONN TO ORSAY", "INITIALISE ORSAY", "READ SETTINGS", "SAVE SETTINGS", "OBJECTIVE LENS", "CONDENSOR LENS", "BLANKING TOGGLE", "TURN ON HEATER", "TURN OFF WOBBLER", "MEASURE HEATER OUTPUT", "TOGGLE GATE VALVE", "SCANNING CONTROLS", "TURN ON BEAM HV", "ENERGY RAMP CYCLE", "TURN ON SUPPRESSOR", "TURN ON EXTRACTOR", "TURN ON WIEN FILTER", "SET ENERGY RANGE", "MEASURE HV SUPPLY VOLTAGES", "SHUTDOWN ION SOURCE", "RESET TYPE II", "PROBE CURRENT FC#1", "PROBE CURRENT FC#2", "VACUUM ", "CHECK 150V", "INITIALISE PI MOTORS", "SET STIGMATOR", "SET WOBBLER FOR OBJECT", "SET OBJ & AP STAGE VELOCITIES", "READ APERTURE POSITIONS", "HOME OBJ & AP STAGES", "DEFINE NEW OBJ", "MOVE OBJ STAGES", "DEFINE NEW APERTURE", "MOVE APERTURE STAGES", "STOP SYSTEM", "TEST COMMANDS"]
            n29 = event-data() -> ()  [unwired: 1 in, 6 out]
            n30 = local read "INTERLOCK STATE"() -> (w164:bool)
            n31 = local read "ION GUN"() -> (w162:bool)
            n32 = Not(x=w164) -> (.not. x?=w163:bool)
            n33 = And(x=w163, y=w162) -> (x .and. y?=w161:bool)
          }
          event "INIT PI": Mouse Down {
            w168 = T16[] [enum."INITIALISE PI MOTORS"] items=["LOOP", "OPEN SERIAL CONN TO ORSAY", "INITIALISE ORSAY", "READ SETTINGS", "SAVE SETTINGS", "OBJECTIVE LENS", "CONDENSOR LENS", "BLANKING TOGGLE", "TURN ON HEATER", "TURN OFF WOBBLER", "MEASURE HEATER OUTPUT", "TOGGLE GATE VALVE", "SCANNING CONTROLS", "TURN ON BEAM HV", "ENERGY RAMP CYCLE", "TURN ON SUPPRESSOR", "TURN ON EXTRACTOR", "TURN ON WIEN FILTER", "SET ENERGY RANGE", "MEASURE HV SUPPLY VOLTAGES", "SHUTDOWN ION SOURCE", "RESET TYPE II", "PROBE CURRENT FC#1", "PROBE CURRENT FC#2", "VACUUM ", "CHECK 150V", "INITIALISE PI MOTORS", "SET STIGMATOR", "SET WOBBLER FOR OBJECT", "SET OBJ & AP STAGE VELOCITIES", "READ APERTURE POSITIONS", "HOME OBJ & AP STAGES", "DEFINE NEW OBJ", "MOVE OBJ STAGES", "DEFINE NEW APERTURE", "MOVE APERTURE STAGES", "STOP SYSTEM", "TEST COMMANDS"]
            n34 = event-data() -> ()  [unwired: 1 in, 8 out]
            n35 = local read "INIT PI"() -> (w167:bool)
          }
          event "ION GUN SETTINGS.SUPPRESSOR": Value Change {
            w174 = T16[] [enum."TURN ON SUPPRESSOR"] items=["LOOP", "OPEN SERIAL CONN TO ORSAY", "INITIALISE ORSAY", "READ SETTINGS", "SAVE SETTINGS", "OBJECTIVE LENS", "CONDENSOR LENS", "BLANKING TOGGLE", "TURN ON HEATER", "TURN OFF WOBBLER", "MEASURE HEATER OUTPUT", "TOGGLE GATE VALVE", "SCANNING CONTROLS", "TURN ON BEAM HV", "ENERGY RAMP CYCLE", "TURN ON SUPPRESSOR", "TURN ON EXTRACTOR", "TURN ON WIEN FILTER", "SET ENERGY RANGE", "MEASURE HV SUPPLY VOLTAGES", "SHUTDOWN ION SOURCE", "RESET TYPE II", "PROBE CURRENT FC#1", "PROBE CURRENT FC#2", "VACUUM ", "CHECK 150V", "INITIALISE PI MOTORS", "SET STIGMATOR", "SET WOBBLER FOR OBJECT", "SET OBJ & AP STAGE VELOCITIES", "READ APERTURE POSITIONS", "HOME OBJ & AP STAGES", "DEFINE NEW OBJ", "MOVE OBJ STAGES", "DEFINE NEW APERTURE", "MOVE APERTURE STAGES", "STOP SYSTEM", "TEST COMMANDS"]
            n36 = event-data() -> ()  [unwired: 1 in, 6 out]
            n37 = local read "INTERLOCK STATE"() -> (w173:bool)
            n38 = local read "ION GUN"() -> (w170:bool)
            n39 = Not(x=w173) -> (.not. x?=w172:bool)
            n40 = And(x=w172, y=w170) -> (x .and. y?=w171:bool)
          }
          event "ION GUN SETTINGS.EXTRACTOR": Value Change {
            w181 = T16[] [enum."TURN ON EXTRACTOR"] items=["LOOP", "OPEN SERIAL CONN TO ORSAY", "INITIALISE ORSAY", "READ SETTINGS", "SAVE SETTINGS", "OBJECTIVE LENS", "CONDENSOR LENS", "BLANKING TOGGLE", "TURN ON HEATER", "TURN OFF WOBBLER", "MEASURE HEATER OUTPUT", "TOGGLE GATE VALVE", "SCANNING CONTROLS", "TURN ON BEAM HV", "ENERGY RAMP CYCLE", "TURN ON SUPPRESSOR", "TURN ON EXTRACTOR", "TURN ON WIEN FILTER", "SET ENERGY RANGE", "MEASURE HV SUPPLY VOLTAGES", "SHUTDOWN ION SOURCE", "RESET TYPE II", "PROBE CURRENT FC#1", "PROBE CURRENT FC#2", "VACUUM ", "CHECK 150V", "INITIALISE PI MOTORS", "SET STIGMATOR", "SET WOBBLER FOR OBJECT", "SET OBJ & AP STAGE VELOCITIES", "READ APERTURE POSITIONS", "HOME OBJ & AP STAGES", "DEFINE NEW OBJ", "MOVE OBJ STAGES", "DEFINE NEW APERTURE", "MOVE APERTURE STAGES", "STOP SYSTEM", "TEST COMMANDS"]
            n41 = event-data() -> ()  [unwired: 1 in, 6 out]
            n42 = local read "INTERLOCK STATE"() -> (w180:bool)
            n43 = local read "ION GUN"() -> (w176:bool)
            n44 = Not(x=w180) -> (.not. x?=w177:bool)
            n45 = And(x=w177, y=w176) -> (x .and. y?=w178:bool)
          }
          event "ION GUN SETTINGS.BEAM ENERGY": Value Change {
            w183 = T16[] [enum."TURN ON BEAM HV"] items=["LOOP", "OPEN SERIAL CONN TO ORSAY", "INITIALISE ORSAY", "READ SETTINGS", "SAVE SETTINGS", "OBJECTIVE LENS", "CONDENSOR LENS", "BLANKING TOGGLE", "TURN ON HEATER", "TURN OFF WOBBLER", "MEASURE HEATER OUTPUT", "TOGGLE GATE VALVE", "SCANNING CONTROLS", "TURN ON BEAM HV", "ENERGY RAMP CYCLE", "TURN ON SUPPRESSOR", "TURN ON EXTRACTOR", "TURN ON WIEN FILTER", "SET ENERGY RANGE", "MEASURE HV SUPPLY VOLTAGES", "SHUTDOWN ION SOURCE", "RESET TYPE II", "PROBE CURRENT FC#1", "PROBE CURRENT FC#2", "VACUUM ", "CHECK 150V", "INITIALISE PI MOTORS", "SET STIGMATOR", "SET WOBBLER FOR OBJECT", "SET OBJ & AP STAGE VELOCITIES", "READ APERTURE POSITIONS", "HOME OBJ & AP STAGES", "DEFINE NEW OBJ", "MOVE OBJ STAGES", "DEFINE NEW APERTURE", "MOVE APERTURE STAGES", "STOP SYSTEM", "TEST COMMANDS"]
            n46 = event-data() -> ()  [unwired: 1 in, 6 out]
            n47 = local read "INTERLOCK STATE"() -> (w182:bool)
            n48 = local read "ION GUN"() -> (w187:bool)
            n49 = Not(x=w182) -> (.not. x?=w186:bool)
            n50 = And(x=w186, y=w187) -> (x .and. y?=w185:bool)
          }
          event "TEST COMMAND": Mouse Down {
            w188 = T16[] [enum."TEST COMMANDS"] items=["LOOP", "OPEN SERIAL CONN TO ORSAY", "INITIALISE ORSAY", "READ SETTINGS", "SAVE SETTINGS", "OBJECTIVE LENS", "CONDENSOR LENS", "BLANKING TOGGLE", "TURN ON HEATER", "TURN OFF WOBBLER", "MEASURE HEATER OUTPUT", "TOGGLE GATE VALVE", "SCANNING CONTROLS", "TURN ON BEAM HV", "ENERGY RAMP CYCLE", "TURN ON SUPPRESSOR", "TURN ON EXTRACTOR", "TURN ON WIEN FILTER", "SET ENERGY RANGE", "MEASURE HV SUPPLY VOLTAGES", "SHUTDOWN ION SOURCE", "RESET TYPE II", "PROBE CURRENT FC#1", "PROBE CURRENT FC#2", "VACUUM ", "CHECK 150V", "INITIALISE PI MOTORS", "SET STIGMATOR", "SET WOBBLER FOR OBJECT", "SET OBJ & AP STAGE VELOCITIES", "READ APERTURE POSITIONS", "HOME OBJ & AP STAGES", "DEFINE NEW OBJ", "MOVE OBJ STAGES", "DEFINE NEW APERTURE", "MOVE APERTURE STAGES", "STOP SYSTEM", "TEST COMMANDS"]
            n51 = event-data() -> ()  [unwired: 1 in, 8 out]
          }
          event "INTERLOCK HV": Mouse Down {
            w191 = T16[] [enum."RESET TYPE II"] items=["LOOP", "OPEN SERIAL CONN TO ORSAY", "INITIALISE ORSAY", "READ SETTINGS", "SAVE SETTINGS", "OBJECTIVE LENS", "CONDENSOR LENS", "BLANKING TOGGLE", "TURN ON HEATER", "TURN OFF WOBBLER", "MEASURE HEATER OUTPUT", "TOGGLE GATE VALVE", "SCANNING CONTROLS", "TURN ON BEAM HV", "ENERGY RAMP CYCLE", "TURN ON SUPPRESSOR", "TURN ON EXTRACTOR", "TURN ON WIEN FILTER", "SET ENERGY RANGE", "MEASURE HV SUPPLY VOLTAGES", "SHUTDOWN ION SOURCE", "RESET TYPE II", "PROBE CURRENT FC#1", "PROBE CURRENT FC#2", "VACUUM ", "CHECK 150V", "INITIALISE PI MOTORS", "SET STIGMATOR", "SET WOBBLER FOR OBJECT", "SET OBJ & AP STAGE VELOCITIES", "READ APERTURE POSITIONS", "HOME OBJ & AP STAGES", "DEFINE NEW OBJ", "MOVE OBJ STAGES", "DEFINE NEW APERTURE", "MOVE APERTURE STAGES", "STOP SYSTEM", "TEST COMMANDS"]
            n52 = event-data() -> ()  [unwired: 1 in, 8 out]
          }
          event "STOP": Mouse Down {
            w194 = T16[] [enum."SHUTDOWN ION SOURCE", enum."STOP SYSTEM"] items=["LOOP", "OPEN SERIAL CONN TO ORSAY", "INITIALISE ORSAY", "READ SETTINGS", "SAVE SETTINGS", "OBJECTIVE LENS", "CONDENSOR LENS", "BLANKING TOGGLE", "TURN ON HEATER", "TURN OFF WOBBLER", "MEASURE HEATER OUTPUT", "TOGGLE GATE VALVE", "SCANNING CONTROLS", "TURN ON BEAM HV", "ENERGY RAMP CYCLE", "TURN ON SUPPRESSOR", "TURN ON EXTRACTOR", "TURN ON WIEN FILTER", "SET ENERGY RANGE", "MEASURE HV SUPPLY VOLTAGES", "SHUTDOWN ION SOURCE", "RESET TYPE II", "PROBE CURRENT FC#1", "PROBE CURRENT FC#2", "VACUUM ", "CHECK 150V", "INITIALISE PI MOTORS", "SET STIGMATOR", "SET WOBBLER FOR OBJECT", "SET OBJ & AP STAGE VELOCITIES", "READ APERTURE POSITIONS", "HOME OBJ & AP STAGES", "DEFINE NEW OBJ", "MOVE OBJ STAGES", "DEFINE NEW APERTURE", "MOVE APERTURE STAGES", "STOP SYSTEM", "TEST COMMANDS"]
            n53 = event-data() -> ()  [unwired: 1 in, 8 out]
          }
          event "HIGH ENERGY": Value Change {
            w197 = T16[] [enum."SET ENERGY RANGE"] items=["LOOP", "OPEN SERIAL CONN TO ORSAY", "INITIALISE ORSAY", "READ SETTINGS", "SAVE SETTINGS", "OBJECTIVE LENS", "CONDENSOR LENS", "BLANKING TOGGLE", "TURN ON HEATER", "TURN OFF WOBBLER", "MEASURE HEATER OUTPUT", "TOGGLE GATE VALVE", "SCANNING CONTROLS", "TURN ON BEAM HV", "ENERGY RAMP CYCLE", "TURN ON SUPPRESSOR", "TURN ON EXTRACTOR", "TURN ON WIEN FILTER", "SET ENERGY RANGE", "MEASURE HV SUPPLY VOLTAGES", "SHUTDOWN ION SOURCE", "RESET TYPE II", "PROBE CURRENT FC#1", "PROBE CURRENT FC#2", "VACUUM ", "CHECK 150V", "INITIALISE PI MOTORS", "SET STIGMATOR", "SET WOBBLER FOR OBJECT", "SET OBJ & AP STAGE VELOCITIES", "READ APERTURE POSITIONS", "HOME OBJ & AP STAGES", "DEFINE NEW OBJ", "MOVE OBJ STAGES", "DEFINE NEW APERTURE", "MOVE APERTURE STAGES", "STOP SYSTEM", "TEST COMMANDS"]
            n54 = event-data() -> ()  [unwired: 1 in, 6 out]
            n55 = local read "INTERLOCK STATE"() -> (w200:bool)
            n56 = Not(x=w200) -> (.not. x?=w199:bool)
          }
          event "OBJECT APERTURE": Value Change {
            w203 = T16[] [enum."MOVE OBJ STAGES"] items=["LOOP", "OPEN SERIAL CONN TO ORSAY", "INITIALISE ORSAY", "READ SETTINGS", "SAVE SETTINGS", "OBJECTIVE LENS", "CONDENSOR LENS", "BLANKING TOGGLE", "TURN ON HEATER", "TURN OFF WOBBLER", "MEASURE HEATER OUTPUT", "TOGGLE GATE VALVE", "SCANNING CONTROLS", "TURN ON BEAM HV", "ENERGY RAMP CYCLE", "TURN ON SUPPRESSOR", "TURN ON EXTRACTOR", "TURN ON WIEN FILTER", "SET ENERGY RANGE", "MEASURE HV SUPPLY VOLTAGES", "SHUTDOWN ION SOURCE", "RESET TYPE II", "PROBE CURRENT FC#1", "PROBE CURRENT FC#2", "VACUUM ", "CHECK 150V", "INITIALISE PI MOTORS", "SET STIGMATOR", "SET WOBBLER FOR OBJECT", "SET OBJ & AP STAGE VELOCITIES", "READ APERTURE POSITIONS", "HOME OBJ & AP STAGES", "DEFINE NEW OBJ", "MOVE OBJ STAGES", "DEFINE NEW APERTURE", "MOVE APERTURE STAGES", "STOP SYSTEM", "TEST COMMANDS"]
            n57 = event-data() -> ()  [unwired: 1 in, 6 out]
          }
          event "BEAM ON": Value Change {
            w207 = T16[] [enum."BLANKING TOGGLE"] items=["LOOP", "OPEN SERIAL CONN TO ORSAY", "INITIALISE ORSAY", "READ SETTINGS", "SAVE SETTINGS", "OBJECTIVE LENS", "CONDENSOR LENS", "BLANKING TOGGLE", "TURN ON HEATER", "TURN OFF WOBBLER", "MEASURE HEATER OUTPUT", "TOGGLE GATE VALVE", "SCANNING CONTROLS", "TURN ON BEAM HV", "ENERGY RAMP CYCLE", "TURN ON SUPPRESSOR", "TURN ON EXTRACTOR", "TURN ON WIEN FILTER", "SET ENERGY RANGE", "MEASURE HV SUPPLY VOLTAGES", "SHUTDOWN ION SOURCE", "RESET TYPE II", "PROBE CURRENT FC#1", "PROBE CURRENT FC#2", "VACUUM ", "CHECK 150V", "INITIALISE PI MOTORS", "SET STIGMATOR", "SET WOBBLER FOR OBJECT", "SET OBJ & AP STAGE VELOCITIES", "READ APERTURE POSITIONS", "HOME OBJ & AP STAGES", "DEFINE NEW OBJ", "MOVE OBJ STAGES", "DEFINE NEW APERTURE", "MOVE APERTURE STAGES", "STOP SYSTEM", "TEST COMMANDS"]
            n58 = event-data() -> ()  [unwired: 1 in, 6 out]
            n59 = local read "INTERLOCK STATE"() -> (w205:bool)
            n60 = Not(x=w205) -> (.not. x?=w204:bool)
          }
          event "WIEN", "E&B": Value Change {
            w208 = T16[] [enum."TURN ON WIEN FILTER"] items=["LOOP", "OPEN SERIAL CONN TO ORSAY", "INITIALISE ORSAY", "READ SETTINGS", "SAVE SETTINGS", "OBJECTIVE LENS", "CONDENSOR LENS", "BLANKING TOGGLE", "TURN ON HEATER", "TURN OFF WOBBLER", "MEASURE HEATER OUTPUT", "TOGGLE GATE VALVE", "SCANNING CONTROLS", "TURN ON BEAM HV", "ENERGY RAMP CYCLE", "TURN ON SUPPRESSOR", "TURN ON EXTRACTOR", "TURN ON WIEN FILTER", "SET ENERGY RANGE", "MEASURE HV SUPPLY VOLTAGES", "SHUTDOWN ION SOURCE", "RESET TYPE II", "PROBE CURRENT FC#1", "PROBE CURRENT FC#2", "VACUUM ", "CHECK 150V", "INITIALISE PI MOTORS", "SET STIGMATOR", "SET WOBBLER FOR OBJECT", "SET OBJ & AP STAGE VELOCITIES", "READ APERTURE POSITIONS", "HOME OBJ & AP STAGES", "DEFINE NEW OBJ", "MOVE OBJ STAGES", "DEFINE NEW APERTURE", "MOVE APERTURE STAGES", "STOP SYSTEM", "TEST COMMANDS"]
            n61 = event-data() -> ()  [unwired: 1 in, 6 out]
            n62 = local read "INTERLOCK STATE"() -> (w211:bool)
            n63 = Not(x=w211) -> (.not. x?=w210:bool)
          }
          event "SHUTDOWN": Mouse Down {
            w212 = T16[] [enum."SHUTDOWN ION SOURCE"] items=["LOOP", "OPEN SERIAL CONN TO ORSAY", "INITIALISE ORSAY", "READ SETTINGS", "SAVE SETTINGS", "OBJECTIVE LENS", "CONDENSOR LENS", "BLANKING TOGGLE", "TURN ON HEATER", "TURN OFF WOBBLER", "MEASURE HEATER OUTPUT", "TOGGLE GATE VALVE", "SCANNING CONTROLS", "TURN ON BEAM HV", "ENERGY RAMP CYCLE", "TURN ON SUPPRESSOR", "TURN ON EXTRACTOR", "TURN ON WIEN FILTER", "SET ENERGY RANGE", "MEASURE HV SUPPLY VOLTAGES", "SHUTDOWN ION SOURCE", "RESET TYPE II", "PROBE CURRENT FC#1", "PROBE CURRENT FC#2", "VACUUM ", "CHECK 150V", "INITIALISE PI MOTORS", "SET STIGMATOR", "SET WOBBLER FOR OBJECT", "SET OBJ & AP STAGE VELOCITIES", "READ APERTURE POSITIONS", "HOME OBJ & AP STAGES", "DEFINE NEW OBJ", "MOVE OBJ STAGES", "DEFINE NEW APERTURE", "MOVE APERTURE STAGES", "STOP SYSTEM", "TEST COMMANDS"]
            n64 = event-data() -> ()  [unwired: 1 in, 8 out]
          }
          event "FILAMENT HEATING", "FILAMENT": Value Change {
            w213 = T16[] [enum."TURN ON HEATER", enum."MEASURE HEATER OUTPUT"] items=["LOOP", "OPEN SERIAL CONN TO ORSAY", "INITIALISE ORSAY", "READ SETTINGS", "SAVE SETTINGS", "OBJECTIVE LENS", "CONDENSOR LENS", "BLANKING TOGGLE", "TURN ON HEATER", "TURN OFF WOBBLER", "MEASURE HEATER OUTPUT", "TOGGLE GATE VALVE", "SCANNING CONTROLS", "TURN ON BEAM HV", "ENERGY RAMP CYCLE", "TURN ON SUPPRESSOR", "TURN ON EXTRACTOR", "TURN ON WIEN FILTER", "SET ENERGY RANGE", "MEASURE HV SUPPLY VOLTAGES", "SHUTDOWN ION SOURCE", "RESET TYPE II", "PROBE CURRENT FC#1", "PROBE CURRENT FC#2", "VACUUM ", "CHECK 150V", "INITIALISE PI MOTORS", "SET STIGMATOR", "SET WOBBLER FOR OBJECT", "SET OBJ & AP STAGE VELOCITIES", "READ APERTURE POSITIONS", "HOME OBJ & AP STAGES", "DEFINE NEW OBJ", "MOVE OBJ STAGES", "DEFINE NEW APERTURE", "MOVE APERTURE STAGES", "STOP SYSTEM", "TEST COMMANDS"]
            n65 = event-data() -> ()  [unwired: 1 in, 6 out]
          }
          event "OBJECTIVE": Value Change {
            w219 = T16[] [enum."OBJECTIVE LENS"] items=["LOOP", "OPEN SERIAL CONN TO ORSAY", "INITIALISE ORSAY", "READ SETTINGS", "SAVE SETTINGS", "OBJECTIVE LENS", "CONDENSOR LENS", "BLANKING TOGGLE", "TURN ON HEATER", "TURN OFF WOBBLER", "MEASURE HEATER OUTPUT", "TOGGLE GATE VALVE", "SCANNING CONTROLS", "TURN ON BEAM HV", "ENERGY RAMP CYCLE", "TURN ON SUPPRESSOR", "TURN ON EXTRACTOR", "TURN ON WIEN FILTER", "SET ENERGY RANGE", "MEASURE HV SUPPLY VOLTAGES", "SHUTDOWN ION SOURCE", "RESET TYPE II", "PROBE CURRENT FC#1", "PROBE CURRENT FC#2", "VACUUM ", "CHECK 150V", "INITIALISE PI MOTORS", "SET STIGMATOR", "SET WOBBLER FOR OBJECT", "SET OBJ & AP STAGE VELOCITIES", "READ APERTURE POSITIONS", "HOME OBJ & AP STAGES", "DEFINE NEW OBJ", "MOVE OBJ STAGES", "DEFINE NEW APERTURE", "MOVE APERTURE STAGES", "STOP SYSTEM", "TEST COMMANDS"]
            n66 = event-data() -> ()  [unwired: 1 in, 6 out]
            n67 = local read "INTERLOCK STATE"() -> (w217:bool)
            n68 = Not(x=w217) -> (.not. x?=w216:bool)
          }
          event "CONDENSOR": Value Change {
            w223 = T16[] [enum."CONDENSOR LENS"] items=["LOOP", "OPEN SERIAL CONN TO ORSAY", "INITIALISE ORSAY", "READ SETTINGS", "SAVE SETTINGS", "OBJECTIVE LENS", "CONDENSOR LENS", "BLANKING TOGGLE", "TURN ON HEATER", "TURN OFF WOBBLER", "MEASURE HEATER OUTPUT", "TOGGLE GATE VALVE", "SCANNING CONTROLS", "TURN ON BEAM HV", "ENERGY RAMP CYCLE", "TURN ON SUPPRESSOR", "TURN ON EXTRACTOR", "TURN ON WIEN FILTER", "SET ENERGY RANGE", "MEASURE HV SUPPLY VOLTAGES", "SHUTDOWN ION SOURCE", "RESET TYPE II", "PROBE CURRENT FC#1", "PROBE CURRENT FC#2", "VACUUM ", "CHECK 150V", "INITIALISE PI MOTORS", "SET STIGMATOR", "SET WOBBLER FOR OBJECT", "SET OBJ & AP STAGE VELOCITIES", "READ APERTURE POSITIONS", "HOME OBJ & AP STAGES", "DEFINE NEW OBJ", "MOVE OBJ STAGES", "DEFINE NEW APERTURE", "MOVE APERTURE STAGES", "STOP SYSTEM", "TEST COMMANDS"]
            n69 = event-data() -> ()  [unwired: 1 in, 6 out]
            n70 = local read "INTERLOCK STATE"() -> (w221:bool)
            n71 = Not(x=w221) -> (.not. x?=w220:bool)
          }
          event "READ & APPLY SETUP": Mouse Down {
            w227 = T16[] [enum."READ SETTINGS"] items=["LOOP", "OPEN SERIAL CONN TO ORSAY", "INITIALISE ORSAY", "READ SETTINGS", "SAVE SETTINGS", "OBJECTIVE LENS", "CONDENSOR LENS", "BLANKING TOGGLE", "TURN ON HEATER", "TURN OFF WOBBLER", "MEASURE HEATER OUTPUT", "TOGGLE GATE VALVE", "SCANNING CONTROLS", "TURN ON BEAM HV", "ENERGY RAMP CYCLE", "TURN ON SUPPRESSOR", "TURN ON EXTRACTOR", "TURN ON WIEN FILTER", "SET ENERGY RANGE", "MEASURE HV SUPPLY VOLTAGES", "SHUTDOWN ION SOURCE", "RESET TYPE II", "PROBE CURRENT FC#1", "PROBE CURRENT FC#2", "VACUUM ", "CHECK 150V", "INITIALISE PI MOTORS", "SET STIGMATOR", "SET WOBBLER FOR OBJECT", "SET OBJ & AP STAGE VELOCITIES", "READ APERTURE POSITIONS", "HOME OBJ & AP STAGES", "DEFINE NEW OBJ", "MOVE OBJ STAGES", "DEFINE NEW APERTURE", "MOVE APERTURE STAGES", "STOP SYSTEM", "TEST COMMANDS"]
            n72 = event-data() -> ()  [unwired: 1 in, 8 out]
            n73 = local read "INTERLOCK STATE"() -> (w225:bool)
            n74 = Not(x=w225) -> (.not. x?=w224:bool)
          }
          event "SCANNING CLUSTER": Value Change {
            w230 = T16[] [enum."SCANNING CONTROLS"] items=["LOOP", "OPEN SERIAL CONN TO ORSAY", "INITIALISE ORSAY", "READ SETTINGS", "SAVE SETTINGS", "OBJECTIVE LENS", "CONDENSOR LENS", "BLANKING TOGGLE", "TURN ON HEATER", "TURN OFF WOBBLER", "MEASURE HEATER OUTPUT", "TOGGLE GATE VALVE", "SCANNING CONTROLS", "TURN ON BEAM HV", "ENERGY RAMP CYCLE", "TURN ON SUPPRESSOR", "TURN ON EXTRACTOR", "TURN ON WIEN FILTER", "SET ENERGY RANGE", "MEASURE HV SUPPLY VOLTAGES", "SHUTDOWN ION SOURCE", "RESET TYPE II", "PROBE CURRENT FC#1", "PROBE CURRENT FC#2", "VACUUM ", "CHECK 150V", "INITIALISE PI MOTORS", "SET STIGMATOR", "SET WOBBLER FOR OBJECT", "SET OBJ & AP STAGE VELOCITIES", "READ APERTURE POSITIONS", "HOME OBJ & AP STAGES", "DEFINE NEW OBJ", "MOVE OBJ STAGES", "DEFINE NEW APERTURE", "MOVE APERTURE STAGES", "STOP SYSTEM", "TEST COMMANDS"]
            n75 = event-data() -> ()  [unwired: 1 in, 6 out]
            n76 = local read "INTERLOCK STATE"() -> (w228:bool)
          }
          event "SAVE SETUP": Mouse Down {
            w233 = T16[] [enum."SAVE SETTINGS"] items=["LOOP", "OPEN SERIAL CONN TO ORSAY", "INITIALISE ORSAY", "READ SETTINGS", "SAVE SETTINGS", "OBJECTIVE LENS", "CONDENSOR LENS", "BLANKING TOGGLE", "TURN ON HEATER", "TURN OFF WOBBLER", "MEASURE HEATER OUTPUT", "TOGGLE GATE VALVE", "SCANNING CONTROLS", "TURN ON BEAM HV", "ENERGY RAMP CYCLE", "TURN ON SUPPRESSOR", "TURN ON EXTRACTOR", "TURN ON WIEN FILTER", "SET ENERGY RANGE", "MEASURE HV SUPPLY VOLTAGES", "SHUTDOWN ION SOURCE", "RESET TYPE II", "PROBE CURRENT FC#1", "PROBE CURRENT FC#2", "VACUUM ", "CHECK 150V", "INITIALISE PI MOTORS", "SET STIGMATOR", "SET WOBBLER FOR OBJECT", "SET OBJ & AP STAGE VELOCITIES", "READ APERTURE POSITIONS", "HOME OBJ & AP STAGES", "DEFINE NEW OBJ", "MOVE OBJ STAGES", "DEFINE NEW APERTURE", "MOVE APERTURE STAGES", "STOP SYSTEM", "TEST COMMANDS"]
            n77 = event-data() -> ()  [unwired: 1 in, 8 out]
          }
          event "WOBBLER SETTINBGS FOR OBJECT ALIGNMENT": Value Change {
            w235 = T16[] [enum."SET WOBBLER FOR OBJECT"] items=["LOOP", "OPEN SERIAL CONN TO ORSAY", "INITIALISE ORSAY", "READ SETTINGS", "SAVE SETTINGS", "OBJECTIVE LENS", "CONDENSOR LENS", "BLANKING TOGGLE", "TURN ON HEATER", "TURN OFF WOBBLER", "MEASURE HEATER OUTPUT", "TOGGLE GATE VALVE", "SCANNING CONTROLS", "TURN ON BEAM HV", "ENERGY RAMP CYCLE", "TURN ON SUPPRESSOR", "TURN ON EXTRACTOR", "TURN ON WIEN FILTER", "SET ENERGY RANGE", "MEASURE HV SUPPLY VOLTAGES", "SHUTDOWN ION SOURCE", "RESET TYPE II", "PROBE CURRENT FC#1", "PROBE CURRENT FC#2", "VACUUM ", "CHECK 150V", "INITIALISE PI MOTORS", "SET STIGMATOR", "SET WOBBLER FOR OBJECT", "SET OBJ & AP STAGE VELOCITIES", "READ APERTURE POSITIONS", "HOME OBJ & AP STAGES", "DEFINE NEW OBJ", "MOVE OBJ STAGES", "DEFINE NEW APERTURE", "MOVE APERTURE STAGES", "STOP SYSTEM", "TEST COMMANDS"]
            n78 = event-data() -> ()  [unwired: 1 in, 6 out]
            n79 = local read "INTERLOCK STATE"() -> (w234:bool)
          }
          event "OBJ APERTURE ALIGNMENT": Value Change {
            w237 = T16[] [enum."MOVE OBJ STAGES"] items=["LOOP", "OPEN SERIAL CONN TO ORSAY", "INITIALISE ORSAY", "READ SETTINGS", "SAVE SETTINGS", "OBJECTIVE LENS", "CONDENSOR LENS", "BLANKING TOGGLE", "TURN ON HEATER", "TURN OFF WOBBLER", "MEASURE HEATER OUTPUT", "TOGGLE GATE VALVE", "SCANNING CONTROLS", "TURN ON BEAM HV", "ENERGY RAMP CYCLE", "TURN ON SUPPRESSOR", "TURN ON EXTRACTOR", "TURN ON WIEN FILTER", "SET ENERGY RANGE", "MEASURE HV SUPPLY VOLTAGES", "SHUTDOWN ION SOURCE", "RESET TYPE II", "PROBE CURRENT FC#1", "PROBE CURRENT FC#2", "VACUUM ", "CHECK 150V", "INITIALISE PI MOTORS", "SET STIGMATOR", "SET WOBBLER FOR OBJECT", "SET OBJ & AP STAGE VELOCITIES", "READ APERTURE POSITIONS", "HOME OBJ & AP STAGES", "DEFINE NEW OBJ", "MOVE OBJ STAGES", "DEFINE NEW APERTURE", "MOVE APERTURE STAGES", "STOP SYSTEM", "TEST COMMANDS"]
            n80 = event-data() -> ()  [unwired: 1 in, 6 out]
          }
          event Value Change {
            w240 = T16[] [enum."SET STIGMATOR"] items=["LOOP", "OPEN SERIAL CONN TO ORSAY", "INITIALISE ORSAY", "READ SETTINGS", "SAVE SETTINGS", "OBJECTIVE LENS", "CONDENSOR LENS", "BLANKING TOGGLE", "TURN ON HEATER", "TURN OFF WOBBLER", "MEASURE HEATER OUTPUT", "TOGGLE GATE VALVE", "SCANNING CONTROLS", "TURN ON BEAM HV", "ENERGY RAMP CYCLE", "TURN ON SUPPRESSOR", "TURN ON EXTRACTOR", "TURN ON WIEN FILTER", "SET ENERGY RANGE", "MEASURE HV SUPPLY VOLTAGES", "SHUTDOWN ION SOURCE", "RESET TYPE II", "PROBE CURRENT FC#1", "PROBE CURRENT FC#2", "VACUUM ", "CHECK 150V", "INITIALISE PI MOTORS", "SET STIGMATOR", "SET WOBBLER FOR OBJECT", "SET OBJ & AP STAGE VELOCITIES", "READ APERTURE POSITIONS", "HOME OBJ & AP STAGES", "DEFINE NEW OBJ", "MOVE OBJ STAGES", "DEFINE NEW APERTURE", "MOVE APERTURE STAGES", "STOP SYSTEM", "TEST COMMANDS"]
            n81 = event-data() -> ()  [unwired: 1 in, 6 out]
            n82 = local read "INTERLOCK STATE"() -> (w241:bool)
          }
          event "HOME ALL AXES": Mouse Down {
            w243 = T16[] [enum."HOME OBJ & AP STAGES"] items=["LOOP", "OPEN SERIAL CONN TO ORSAY", "INITIALISE ORSAY", "READ SETTINGS", "SAVE SETTINGS", "OBJECTIVE LENS", "CONDENSOR LENS", "BLANKING TOGGLE", "TURN ON HEATER", "TURN OFF WOBBLER", "MEASURE HEATER OUTPUT", "TOGGLE GATE VALVE", "SCANNING CONTROLS", "TURN ON BEAM HV", "ENERGY RAMP CYCLE", "TURN ON SUPPRESSOR", "TURN ON EXTRACTOR", "TURN ON WIEN FILTER", "SET ENERGY RANGE", "MEASURE HV SUPPLY VOLTAGES", "SHUTDOWN ION SOURCE", "RESET TYPE II", "PROBE CURRENT FC#1", "PROBE CURRENT FC#2", "VACUUM ", "CHECK 150V", "INITIALISE PI MOTORS", "SET STIGMATOR", "SET WOBBLER FOR OBJECT", "SET OBJ & AP STAGE VELOCITIES", "READ APERTURE POSITIONS", "HOME OBJ & AP STAGES", "DEFINE NEW OBJ", "MOVE OBJ STAGES", "DEFINE NEW APERTURE", "MOVE APERTURE STAGES", "STOP SYSTEM", "TEST COMMANDS"]
            n83 = event-data() -> ()  [unwired: 1 in, 8 out]
          }
        }
      }
      frame True {
        w249 = T20[] [] items=["LOOP", "INIT STAGE CONTROLLER", "SEND COMMAND TO CONTROLLER", "HOME X", "HOME Y", "HOME Z", "ABORT ALL AXES", "GOTO MARKER", "ZERO XYZ", "READ XYZ POSITIONS", "GOTO XYZ POSITION", "STOP", "JOG XYZ", "WAIT FOR MOVE COMPLETE"]
        n84 = local write "ION GUN SETTINGS"(T19 {"BEAM ENERGY"=0.0, "EXTRACTOR"=0.0, "SUPPRESSOR"=0.0, "ION CURRENT"=0.0} ("ION GUN SETTINGS")) -> ()
      }
    }
    n85 = case shown="True" w69 {
      tunnel: w84 -> [w263 w273]
      tunnel: w83 -> [w262 w272]
      tunnel: [w263 w271] -> w82
      tunnel: [w262 w270] -> w79
      frame False {
      }
      frame True {
        w267 = string[] [] ("PROCESSES")
        n86 = local write "STOP"(FALSE ("STOP")) -> ()
        n87 = local write "ION GUN"(FALSE ("TURN ON GUN")) -> ()
        n88 = for {
          shift-right: [w276] -> w271
          shift-left: w273 -> [w278]
          shift-right: [w275] -> w270
          shift-left: w272 -> [w277]
          tunnel: "STARTUP" -> [w274] mode=indexing
          n89 = Enqueue Element(queue=w278, element=w274, error in (no error)=w277) -> (queue out=w276:refnum<queue>, error out=w275:errorcluster)  [unwired: 1 in, 1 out]
        }
        n90 = property on="FILAMENT HEATING" class="Slide (strict)"("DisabledEnum"=T18."Disabled and Grayed Out" ("Disabled")) -> ()  [unwired: 2 in, 2 out]
        n91 = call <vilib>:"Flush Shared Variable Data.vi"() -> ()  [unwired: 11 in, 1 out]
        "PROCESSES" <- w267
        "SERIAL \nRESPONSE" <- w267
        "PREVIOUS GUN SETTINGS" <- T1 {"BEAM ENERGY"=0.0, "SUPPRESSOR"=0.0, "EXTRACTOR"=0.0, "ION CURRENT"=0.0} ("PREVIOUS GUN SETTINGS")
      }
    }
    n92 = case shown="False" w69 {
      tunnel: [w101 FALSE] -> w64
      tunnel: [w100 w112] -> w63
      tunnel: [w99 FALSE] -> _
      frame False {
        n93 = event shown="[2] \"EXPOSURE\": Value Change" {
          selector: _ -> [_ _ _]
          dyn-events: _ -> [_ _ _]
          timeout: 150 -> [_ _ _]
          tunnel: [TRUE TRUE TRUE] -> w101
          tunnel: [FALSE TRUE TRUE] -> w99
          tunnel: [w103 w108 w111] -> w100
          event Timeout {
            w103 = T17[] [enum."LOOP"] items=["INIT VIDEO", "CAMERA GAIN", "CAMERA EXPOSURE", "LOOP"]
            n94 = event-data() -> ()  [unwired: 1 in, 3 out]
          }
          event "GAIN", "GAIN METHOD": Value Change {
            w108 = T17[] [enum."CAMERA GAIN"] items=["INIT VIDEO", "CAMERA GAIN", "CAMERA EXPOSURE", "LOOP"]
            n95 = event-data() -> ()  [unwired: 1 in, 6 out]
          }
          event "EXPOSURE": Value Change {
            w111 = T17[] [enum."CAMERA EXPOSURE"] items=["INIT VIDEO", "CAMERA GAIN", "CAMERA EXPOSURE", "LOOP"]
            n96 = event-data() -> ()  [unwired: 1 in, 6 out]
          }
        }
      }
      frame True {
        w112 = T17[] [] items=["INIT VIDEO", "CAMERA GAIN", "CAMERA EXPOSURE", "LOOP"]
      }
    }
    n97 = case shown="True" w69 {
      tunnel: w68 -> [w116 w121]
      tunnel: w67 -> [w115 w120]
      tunnel: [w116 w119] -> w66
      tunnel: [w115 w118] -> w65
      frame False {
      }
      frame True {
        w117 = T17[] [enum."INIT VIDEO", enum."CAMERA EXPOSURE"] items=["INIT VIDEO", "CAMERA GAIN", "CAMERA EXPOSURE", "LOOP"]
        n98 = for {
          shift-right: [w124] -> w119
          shift-left: w121 -> [w126]
          shift-right: [w123] -> w118
          shift-left: w120 -> [w125]
          tunnel: w117 -> [w122] mode=indexing
          n99 = Enqueue Element(queue=w126, element=w122, error in (no error)=w125) -> (queue out=w124:refnum<queue>, error out=w123:errorcluster)  [unwired: 1 in, 1 out]
        }
      }
    }
    n100 = local read "ION GUN SETTINGS"() -> (w48:T1)
    n101 = case shown="True" w64 {
      tunnel: w66 -> [w88 w93]
      tunnel: w63 -> [_ w92]
      tunnel: [w88 w91] -> w62
      tunnel: [w87 w90] -> w61
      tunnel: w65 -> [w87 w89]
      frame False {
      }
      frame True {
        n102 = for {
          shift-right: [w96] -> w91
          shift-left: w93 -> [w98]
          shift-right: [w95] -> w90
          shift-left: w89 -> [w97]
          tunnel: w92 -> [w94] mode=indexing
          n103 = Enqueue Element(queue=w98, element=w94, error in (no error)=w97) -> (queue out=w96:refnum<queue>, error out=w95:errorcluster)  [unwired: 1 in, 1 out]
        }
      }
    }
    n104 = case shown="True" w81 {
      tunnel: w82 -> [w251 w256]
      tunnel: w80 -> [_ w255]
      tunnel: [w251 w254] -> w78
      tunnel: [w250 w253] -> w75
      tunnel: w79 -> [w250 w252]
      frame False {
      }
      frame True {
        n105 = for {
          shift-right: [w259] -> w254
          shift-left: w256 -> [w261]
          shift-right: [w258] -> w253
          shift-left: w252 -> [w260]
          tunnel: w255 -> [w257] mode=indexing
          n106 = Enqueue Element(queue=w261, element=w257, error in (no error)=w260) -> (queue out=w259:refnum<queue>, error out=w258:errorcluster)  [unwired: 1 in, 1 out]
        }
      }
    }
    n107 = Unbundle By Name(w48) -> ("BEAM ENERGY"=w40:sgl[unit])
    n108 = local read "VACUUM STATE"() -> (w71:bool)
    n109 = local read "150V GOOD"() -> (w72:bool)
    n110 = Greater Or Equal?(x=w40, y=sgl[unit] 10000.0) -> (x >= y?=→"HIGH ENERGY":bool)
    n111 = node("SETTINGS DELAY") -> (w43:dbl)
    n112 = Or(x=w75, y=w77) -> (x .or. y?=w45:bool)
    n113 = To Unsigned Long Integer(number=w43) -> (unsigned 32bit integer=→"TIMER":u32)
    n114 = local read "CONDENSOR"() -> (w50:cluster{"COARSE":sgl[unit], "FINE":sgl[unit]})
    n115 = Compound Arithmetic op=AND(w71, w72) -> (w58:bool)
    n116 = local read "OBJECTIVE"() -> (w49:cluster{"COARSE":sgl[unit], "FINE":sgl[unit]})
    n117 = property on="PROCESSES" class="Arr (strict)"() -> ("Index Values"=w57:u32[])  [unwired: 2 in, 2 out]
    n118 = Not(x=w58) -> (.not. x?=→"INTERLOCK STATE":bool)
    n119 = case shown="True" w58 {
      tunnel: [T18."Disabled and Grayed Out" ("Disabled") T18."Enabled" ("Disabled")] -> w60
      tunnel: [TRUE FALSE] -> w70
      frame False {
      }
      frame True {
      }
    }
    n120 = Unbundle By Name(w49) -> ("COARSE"=w52:sgl[unit], "FINE"=w51:sgl[unit])
    n121 = Unbundle By Name(w50) -> ("COARSE"=w53:sgl[unit], "FINE"=w54:sgl[unit])
    n122 = property on="SERIAL \nRESPONSE" class="Arr (strict)"("Index Values"=w57) -> ()  [unwired: 2 in, 2 out]
    n123 = Get Queue Status(queue=w78, return elements? (F)=TRUE, error in (no error)=w75) -> (queue out=w76:refnum<queue>, error out=w73:errorcluster)  [unwired: 6 out]
    n124 = Add(x=w53, y=w54) -> (x+y=→"CONDENSOR":sgl[unit])
    n125 = Add(x=w52, y=w51) -> (x+y=→"OBJECTIVE":sgl[unit])
    n126 = First Call?() -> (First Call?: T/F=w44:bool)
    n127 = case shown="True" w44 {
      frame False {
      }
      frame True {
        w85 = dbl[unit][] [] ("History Data")
        w86 = dbl[unit][] [] ("History Data")
        n128 = property on="BEAM VOLTAGE" class="WFChart (strict)"("History Data"=w86) -> ()  [unwired: 2 in, 2 out]
        n129 = property on="BEAM CURRENT" class="WFChart (strict)"("History Data"=w85) -> ()  [unwired: 2 in, 2 out]
        n130 = property on="EXTRACTOR  CURRENT" class="WFChart (strict)"("History Data"=w85) -> ()  [unwired: 2 in, 2 out]
        n131 = property on="EXTRACTOR" class="WFChart (strict)"("History Data"=w86) -> ()  [unwired: 2 in, 2 out]
        n132 = property on="CONDENSOR CURRENT" class="WFChart (strict)"("History Data"=w85) -> ()  [unwired: 2 in, 2 out]
        n133 = property on="CONDENSOR VOLTAGE" class="WFChart (strict)"("History Data"=w86) -> ()  [unwired: 2 in, 2 out]
        n134 = property on="OBJECTIVE CURRENT" class="WFChart (strict)"("History Data"=w85) -> ()  [unwired: 2 in, 2 out]
        n135 = property on="OBJECTIVE VOLTAGE" class="WFChart (strict)"("History Data"=w86) -> ()  [unwired: 2 in, 2 out]
        n136 = property on="SUPPRESSOR CURRENT" class="WFChart (strict)"("History Data"=w85) -> ()  [unwired: 2 in, 2 out]
        n137 = property on="SUPPRESSOR VOLTAGE" class="WFChart (strict)"("History Data"=w86) -> ()  [unwired: 2 in, 2 out]
      }
    }
    n138 = property on="BEAM ON" class="Bool (strict)"("DisabledEnum"=w60) -> ()  [unwired: 2 in, 2 out]
    n139 = property on="ION GUN" class="Bool (strict)"("DisabledEnum"=w60) -> ()  [unwired: 2 in, 2 out]
    n140 = property on="WARNING" class="Str"("DisabledEnum"=w60) -> ()  [unwired: 2 in, 2 out]
    n141 = property on="INTERLOCK STATE" class="Bool (strict)"("Blinking"=w70) -> ()  [unwired: 2 in, 2 out]
    n142 = property on="ION GUN SETTINGS" class="Clust (strict)"("DisabledEnum"=w60) -> ()  [unwired: 2 in, 2 out]
  }
  n143 = while {
    shift-right: [w285] -> _
    shift-left: string[] [] -> [w286]
    shift-right: [w280] -> _
    shift-left: string[] [] -> [w284]
    shift-right: [w283] -> _
    shift-left: w10 -> [w281]
    border: i32[] [] -> [_]
    border: dbl[unit][] [] -> [_]
    border: 0 -> [_]
    stop <- TRUE continue-if-true
    n144 = Dequeue Element(queue=w281) -> (queue out=w282:refnum<queue>, element=w287:T16)  [unwired: 2 in, 2 out]
    n145 = case shown="\"TURN ON WIEN FILTER\"" w287 {
      tunnel: w286 -> [w295 w326 w383 w414 w441 w525 w544 w588 w643 w657 w662 w673 w732 w780 w811 w841 w866 w942 w973 w1053 w1128 w1177 w1196 w1233 w1240 w1285 w1430 w1490 w1537 w1553 w1557 w1569 w1582 w1612 w1619 w1622 w1635 w1657]
      tunnel: [w293 w324 w381 w414 w440 w523 w543 w589 w643 w658 w662 w670 w731 w779 w810 w841 w865 w942 w972 w1052 w1128 w1177 w1196 w1232 w1238 w1285 w1430 w1487 w1535 w1553 w1557 w1569 w1582 w1611 w1619 w1622 w1635 w1657] -> w285
      tunnel: w284 -> [w292 w322 w384 w413 w439 w521 w542 w590 w641 w645 w660 w672 w767 w778 w812 w853 w868 w943 w975 w1055 w1129 w1178 w1198 w1230 w1241 w1283 w1428 w1488 w1538 w1551 w1555 w1567 w1580 w1615 w1617 w1620 w1633 w1655]
      tunnel: [w289 w320 w379 w413 w434 w515 w539 w578 w641 w645 w660 w667 w767 w775 w805 w838 w867 w943 w974 w1054 w1129 w1178 w1198 w1230 w1235 w1283 w1428 w1485 w1533 w1551 w1555 w1567 w1580 w1614 w1617 w1620 w1633 w1655] -> w280
      tunnel: [w290 w321 w380 w412 w435 w535 w540 w580 w642 w655 w661 w668 w768 w776 w806 w840 w863 w944 w970 w1050 w1130 w1176 w1197 w1231 w1236 w1284 w1429 w1486 w1534 w1552 w1556 w1568 w1581 w1616 w1618 w1621 w1634 w1656] -> w283
      tunnel: w282 -> [w290 w321 w380 w412 w436 w535 w540 w580 w642 w655 w661 w668 w768 w776 w806 w840 w863 w944 w970 w1050 w1130 w1176 w1197 w1231 w1236 w1284 w1429 w1486 w1534 w1552 w1556 w1568 w1581 w1616 w1618 w1621 w1634 w1656]
      frame "LOOP", Default {
        w288 = dbl[unit][] [] ("EXTRACTOR RAMP")
        w294 = "LOOP" ("PROCESS")
        n146 = local read "WOBBLER SETTINBGS FOR OBJECT ALIGNMENT"() -> (w298:T10)
        n147 = case shown="False" FALSE {
          frame False {
          }
          frame True {
            w302 = T24 16 items=["Flush Receive Buffer"=16, "Write Transmit Buffer to Device"=32, "Flush Receive Buffer (No I/O)"=64, "Flush Transmit Buffer"=128] ("Mask")
            n148 = local read "NO CONTROLLER"() -> (w307:bool)
            n149 = case shown="False" w307 {
              frame False {
                # "Query position for selected\naxes, not for all axes"
                n150 = call "POS?.vi"("System no."=1, "All axes?"=TRUE) -> ("Position"=w308:dbl[])  [unwired: 3 in, 14 out]
                n151 = local write "POSITIONS"(w308) -> ()
              }
              frame True {
              }
            }
            n152 = local read "VISA ERROR"() -> (w305:errorcluster)
            n153 = local read "ORSAY"() -> (w304:refnum<visa-resource-name>)
            n154 = VISA Flush I/O Buffer(VISA resource name=w304, mask (16)=w302, error in (no error)=w305) -> (VISA resource name out=w303:refnum<visa-resource-name>, error out=w306:errorcluster)
            n155 = local write "ORSAY"(w303) -> ()
            n156 = local write "VISA ERROR"(w306) -> ()
          }
        }
        n157 = local write "BEAM RAMP"(w288) -> ()
        n158 = local write "SUPPRESSOR RAMP"(w288) -> ()
        n159 = local write "EXTRACTOR RAMP"(w288) -> ()
        n160 = Unbundle By Name(w298) -> ("WOBBLE"=w297:u16)
        n161 = local write "PROCESS"(w294) -> ()
        n162 = case shown="1" w297 {
          tunnel: [TRUE FALSE FALSE] -> w301
          tunnel: [FALSE TRUE FALSE] -> w300
          tunnel: [FALSE FALSE TRUE] -> w299
          frame 0, Default {
          }
          frame 1 {
          }
          frame 2 {
          }
        }
        n163 = Build Array (concatenate)(w295, w294) -> (w293:string[])
        n164 = property class="DigNum (strict)"("Blinking"=w301) -> ()  [unwired: 2 in, 2 out]
        n165 = property class="DigNum (strict)"("Blinking"=w300) -> ()  [unwired: 2 in, 2 out]
        n166 = property class="DigNum (strict)"("Blinking"=w299) -> ()  [unwired: 2 in, 2 out]
        n167 = local write "PROCESSES"(w293) -> ()
        n168 = Build Array (concatenate)(w292, "LOOP") -> (w289:string[])
        n169 = local write "SERIAL \nRESPONSE"(w289) -> ()
      }
      frame "OPEN SERIAL CONN TO ORSAY" {
        w325 = "OPENING SERIAL CONNECTION TO ORSAY MB" ("PROCESS")
        n170 = flat-sequence {
          tunnel: [w338] -> w323
          frame #0 {
            w330 = T24 128 items=["Flush Receive Buffer"=16, "Write Transmit Buffer to Device"=32, "Flush Receive Buffer (No I/O)"=64, "Flush Transmit Buffer"=128] ("Mask")
            w347 = T24 16 items=["Flush Receive Buffer"=16, "Write Transmit Buffer to Device"=32, "Flush Receive Buffer (No I/O)"=64, "Flush Transmit Buffer"=128] ("Mask")
            n171 = case shown="0, Default" "TERMINATION CHAR" {
              tunnel: [0 13 10] -> w336
              tunnel: [w359 w362 w367] -> w335
              tunnel: [w358 w361 w366] -> w334
              tunnel: ["" "\r" "\n"] -> w327
              frame 0, Default {
                w358 = u16 0 items=["None", "Last Bit", "TermChar"] ("Serial Settings:End Mode for Reads")
                w359 = u16 0 items=["None", "Last Bit", "TermChar"] ("Serial Settings:End Mode for Reads")
              }
              frame 1 {
                w361 = u16 0 items=["None", "Last Bit", "TermChar"] ("Serial Settings:End Mode for Reads")
                w362 = u16 2 items=["None", "Last Bit", "TermChar"] ("Serial Settings:End Mode for Reads")
              }
              frame 2 {
                w366 = u16 0 items=["None", "Last Bit", "TermChar"] ("Serial Settings:End Mode for Reads")
                w367 = u16 2 items=["None", "Last Bit", "TermChar"] ("Serial Settings:End Mode for Reads")
              }
            }
            "APPEND" <- w327
            n172 = call-poly "VISA Configure Serial Port"("VISA resource name"=refnum<visa-resource-name> "ORSAY-USB", "Enable Termination\nChar (T)"=FALSE ("Enable Termination\nChar (T)"), "baud rate (9600)"=9600) -> ("VISA resource name out"=w351:refnum<visa-resource-name>, "error out"=w350:errorcluster)  [unwired: 11 in]
            n173 = property class="Instr"(reference=w351, error in=w350, "Serial Settings:End Mode for Writes"=w335, "Message Based Settings:Send End Enable"="TERMINATION", "Message Based Settings:Termination Character"=w336, "ASRL End In"=w334) -> (reference out=w342:refnum<visa-resource-name>, error out=w340:errorcluster)
            n174 = flat-sequence {
              tunnel: [w370] -> w341
              tunnel: w342 -> [w370]
              tunnel: [w369] -> w339
              tunnel: w340 -> [w369]
              frame #0 {
                n175 = Wait (ms)(milliseconds to wait=u32 200) -> ()  [unwired: 1 out]
              }
            }
            n176 = property class="Instr"(reference=w341, error in=w339) -> (reference out=w346:refnum<visa-resource-name>, error out=w343:errorcluster, "Serial Settings:Number of Bytes at Serial Port"=w344:u32)
            n177 = VISA Read(VISA resource name=w346, byte count=w344, error in (no error)=w343) -> (VISA resource name out=w345:refnum<visa-resource-name>, read buffer=w338:string, error out=w332:errorcluster)  [unwired: 1 out]
            n178 = VISA Flush I/O Buffer(VISA resource name=w345, mask (16)=w330, error in (no error)=w332) -> (VISA resource name out=w333:refnum<visa-resource-name>, error out=w331:errorcluster)
            n179 = VISA Flush I/O Buffer(VISA resource name=w333, mask (16)=w347, error in (no error)=w331) -> (VISA resource name out=→"ORSAY":refnum<visa-resource-name>, error out=→"VISA ERROR":errorcluster)
            n180 = Unbundle By Name(w331) -> ("status"=w353:bool)
            n181 = Not(x=w353) -> (.not. x?=→"ORSAY CONNECTED":bool)
          }
          frame #1 {
            n182 = Wait (ms)(milliseconds to wait=u32 2000 ("millisecond timer value")) -> ()  [unwired: 1 out]
          }
        }
        n183 = local write "PROCESS"(w325) -> ()
        n184 = Build Array (concatenate)(w326, w325) -> (w324:string[])
        n185 = Build Array (concatenate)(w322, w323) -> (w320:string[])
        n186 = local write "SERIAL \nRESPONSE"(w320) -> ()
      }
      frame "INITIALISE ORSAY" {
        w374 = cluster{"COARSE":sgl[unit], "FINE":sgl[unit]} {"COARSE"=0.0, "FINE"=0.0} ("CONDENSOR")
        w378 = dbl[unit][] [] ("SUPPRESSOR RAMP")
        w382 = "RESET ORSAY" ("PROCESS")
        n187 = flat-sequence {
          tunnel: [w392] -> w385
          tunnel: "DS CF12,58A4,30EE,58A4,7630,24B2,7630,DB4E,0" -> [w389]
          frame #0 {
            n188 = local read "APPEND"() -> (w390:string)
            n189 = Concatenate Strings("RE 1" ("ORSAY COMMAND"), w390) -> (w387:string)
            n190 = Concatenate Strings(w389, w390) -> (w386:string)
            n191 = local read "ORSAY"() -> (w394:refnum<visa-resource-name>)
            n192 = Build Array(w387, w386) -> (w388:string[])
            n193 = for {
              tunnel: [w407] -> w395
              tunnel: [w404] -> w392
              tunnel: w388 -> [w396] mode=indexing
              shift-right: [w405] -> w393
              shift-left: w394 -> [w406]
              n194 = VISA Write(VISA resource name=w406, write buffer=w396) -> (VISA resource name out=w400:refnum<visa-resource-name>, error out=w399:errorcluster)  [unwired: 1 in, 1 out]
              n195 = flat-sequence {
                tunnel: w400 -> [w408]
                tunnel: [w410] -> w397
                tunnel: w399 -> [w410]
                tunnel: [w408] -> w398
                frame #0 {
                  n196 = Wait (ms)(milliseconds to wait=u32 1000) -> ()  [unwired: 1 out]
                }
              }
              n197 = property class="Instr"(reference=w398, error in=w397) -> (reference out=w401:refnum<visa-resource-name>, error out=w403:errorcluster, "Serial Settings:Number of Bytes at Serial Port"=w402:u32)
              n198 = VISA Read(VISA resource name=w401, byte count=w402, error in (no error)=w403) -> (VISA resource name out=w405:refnum<visa-resource-name>, read buffer=w404:string, error out=w407:errorcluster)  [unwired: 1 out]
            }
            n199 = local write "ORSAY"(w393) -> ()
            n200 = local write "VISA ERROR"(w395) -> ()
          }
          frame #1 {
            n201 = Wait (ms)(milliseconds to wait=u32 200) -> ()  [unwired: 1 out]
          }
        }
        n202 = Build Array (concatenate)(w383, w382) -> (w381:string[])
        n203 = local write "PROCESS"(w382) -> ()
        n204 = Build Array (concatenate)(w384, w385) -> (w379:string[])
        n205 = local write "SERIAL \nRESPONSE"(w379) -> ()
        n206 = local write "CONDENSOR"(w374) -> ()
        n207 = local write "OBJECTIVE"(w374) -> ()
        n208 = property on="SUPPRESSOR" class="Slide (strict)"("DisabledEnum"=T18."Disabled and Grayed Out" ("Disabled")) -> ()  [unwired: 2 in, 2 out]
        n209 = property on="ION CURRENT" class="Slide (strict)"("DisabledEnum"=T18."Disabled and Grayed Out" ("Disabled")) -> ()  [unwired: 2 in, 2 out]
        n210 = property on="EXTRACTOR" class="Slide (strict)"("DisabledEnum"=T18."Disabled and Grayed Out" ("Disabled")) -> ()  [unwired: 2 in, 2 out]
        n211 = property on="SUPPRESSOR" class="Slide (strict)" props=["DisabledEnum"]() -> ()  [unwired: 2 in, 3 out]
        n212 = local write "ION GUN SETTINGS"(T19 {"BEAM ENERGY"=0.0, "EXTRACTOR"=0.0, "SUPPRESSOR"=0.0, "ION CURRENT"=0.0} ("ION GUN SETTINGS")) -> ()
        n213 = local write "EXTRACTOR RAMP"(w378) -> ()
        n214 = local write "BEAM RAMP"(w378) -> ()
        n215 = local write "SUPPRESSOR RAMP"(w378) -> ()
        "SUPPRESSOR RAMP" <- w378
        "EXTRACTOR RAMP" <- w378
        "BEAM RAMP" <- w378
      }
      frame "TEST COMMANDS" {
        n216 = flat-sequence {
          frame #0 {
            n217 = local read "APPEND"() -> (w425:string)
            n218 = Concatenate Strings("TEST COMMAND", w425) -> (w416:string)
            n219 = local read "VISA ERROR"() -> (w426:errorcluster)
            n220 = local read "ORSAY"() -> (w427:refnum<visa-resource-name>)
            n221 = VISA Write(VISA resource name=w427, write buffer=w416, error in (no error)=w426) -> (VISA resource name out=w420:refnum<visa-resource-name>, error out=w419:errorcluster)  [unwired: 1 out]
            n222 = flat-sequence {
              tunnel: w420 -> [w430]
              tunnel: [w432] -> w417
              tunnel: w419 -> [w432]
              tunnel: [w430] -> w418
              frame #0 {
                n223 = Wait (ms)(milliseconds to wait=u32 1000) -> ()  [unwired: 1 out]
              }
            }
            n224 = property class="Instr"(reference=w418, error in=w417) -> (reference out=w421:refnum<visa-resource-name>, error out=w423:errorcluster, "Serial Settings:Number of Bytes at Serial Port"=w422:u32)
            n225 = VISA Read(VISA resource name=w421, byte count=w422, error in (no error)=w423) -> (VISA resource name out=w429:refnum<visa-resource-name>, read buffer=→"TEST OUTPUT":string, error out=w428:errorcluster)  [unwired: 1 out]
            n226 = local write "ORSAY"(w429) -> ()
            n227 = local write "VISA ERROR"(w428) -> ()
          }
          frame #1 {
            n228 = local write "TEST COMMAND"(FALSE ("TEST COMMAND")) -> ()
          }
        }
      }
      frame "VACUUM " {
        w442 = "VACUUM CHECK"
        w475 = i16 2
        w474 = i16 2
        # "Bypass"
        # "Where is the column vac ?\nMust be before manual GV"
        # "Need a measure of vac in the target chamber & valve ??"
        n229 = local read "VISA ERROR"() -> (w492:errorcluster)
        n230 = local read "APPEND"() -> (w438:string)
        n231 = local read "ORSAY"() -> (w493:refnum<visa-resource-name>)
        n232 = Concatenate Strings("GV F", w438) -> (w454:string)
        n233 = Concatenate Strings("GV D", w438) -> (w452:string)
        n234 = VISA Write(VISA resource name=w493, write buffer=w454, error in (no error)=w492) -> (VISA resource name out=w450:refnum<visa-resource-name>, error out=w448:errorcluster)  [unwired: 1 out]
        n235 = flat-sequence {
          tunnel: [w505] -> w444
          tunnel: w447 -> [w505]
          tunnel: [w504] -> w445
          tunnel: w446 -> [w504]
          frame #0 {
            n236 = Wait (ms)(milliseconds to wait=u32 200) -> ()  [unwired: 1 out]
          }
        }
        n237 = flat-sequence {
          tunnel: [w508] -> w451
          tunnel: w450 -> [w508]
          tunnel: [w507] -> w449
          tunnel: w448 -> [w507]
          frame #0 {
            n238 = Wait (ms)(milliseconds to wait=u32 200) -> ()  [unwired: 1 out]
          }
        }
        n239 = property class="Instr"(reference=w451, error in=w449) -> (reference out=w461:refnum<visa-resource-name>, error out=w460:errorcluster, "Serial Settings:Number of Bytes at Serial Port"=w459:u32)
        n240 = property class="Instr"(reference=w444, error in=w445) -> (reference out=w458:refnum<visa-resource-name>, error out=w456:errorcluster, "Serial Settings:Number of Bytes at Serial Port"=w457:u32)
        n241 = VISA Read(VISA resource name=w461, byte count=w459, error in (no error)=w460) -> (VISA resource name out=w473:refnum<visa-resource-name>, read buffer=w463:string)  [unwired: 2 out]
        n242 = VISA Write(VISA resource name=w473, write buffer=w452) -> (VISA resource name out=w447:refnum<visa-resource-name>, error out=w446:errorcluster)  [unwired: 1 in, 1 out]
        n243 = VISA Read(VISA resource name=w458, byte count=w457, error in (no error)=w456) -> (VISA resource name out=w472:refnum<visa-resource-name>, read buffer=w462:string, error out=w471:errorcluster)  [unwired: 1 out]
        n244 = local write "ORSAY"(w472) -> ()
        n245 = local write "VISA ERROR"(w471) -> ()
        n246 = Concatenate Strings(w463, w462) -> (w443:string)
        n247 = Match Pattern(string=w463, regular expression=",") -> (before substring=w481:string)  [unwired: 1 in, 3 out]
        n248 = Match Pattern(string=w462, regular expression=",") -> (before substring=w483:string)  [unwired: 1 in, 3 out]
        n249 = property on="COLUMN VACUUM" class="Knob (strict)"("Scale.RampVis"=TRUE ("Scale.Ramp Visible")) -> ()  [unwired: 2 in, 2 out]
        n250 = local write "PROCESS"(w442) -> ()
        n251 = Hexadecimal String To Number(string=w481, offset=w474, default (0uL)=w474) -> (number=w485:i16)  [unwired: 1 out]
        n252 = Hexadecimal String To Number(string=w483, offset=w475, default (0uL)=w475) -> (number=w482:i16)  [unwired: 1 out]
        n253 = Absolute Value(x=w482) -> (abs(x)=w487:i16)
        n254 = Less?(x=w485, y=320) -> (x < y?=w488:bool)
        n255 = Build Array (concatenate)(w441, w442) -> (w440:string[])
        n256 = Equal To 0?(x=w485) -> (x = 0?=w484:bool)
        n257 = Equal To 0?(x=w487) -> (x = 0?=w486:bool)
        n258 = Build Array (concatenate)(w439, w443) -> (w434:string[])
        n259 = local write "PROCESSES"(w440) -> ()
        n260 = Select(t=i16 1, s=w484, f=w485) -> (s? t:f=w489:i16)
        n261 = Select(t=i16 1, s=w486, f=w487) -> (s? t:f=w490:i16)
        n262 = case shown="True" w488 {
          tunnel: w489 -> [w510 _]
          tunnel: w490 -> [_ w513]
          tunnel: [w509 w514] -> w491
          frame False {
            n263 = To Single Precision Float(number=w510) -> (single precision float=w509:sgl)
          }
          frame True {
            n264 = To Single Precision Float(number=w513) -> (single precision float=w511:sgl)
            n265 = Divide(x=w511, y=sgl 20.0) -> (x/y=w514:sgl)
          }
        }
        n266 = formula code="k=log(lp/3276700)-2.7;\np=10** k;"("lp"=w491) -> ("p"=w469:dbl)  [unwired: 1 out]
        n267 = node(w469) -> (w464:dbl[unit])
        "COLUMN VACUUM" <- w464
        n268 = Bundle(w464, "COLUMN THRESHOLD"="COLUMN THRESHOLD") -> (→"COLUMN VACUUM":cluster{dbl[unit], "COLUMN THRESHOLD":dbl[unit]})  [unwired: 1 in]
        n269 = Bundle(w464, "CHAMBER THRESHOLD"="CHAMBER THRESHOLD") -> (→"CHAMBER VACUUM":T25)  [unwired: 1 in]
        n270 = Less?(x=w464, y="COLUMN THRESHOLD") -> (x < y?=w437:bool)
        "VACUUM STATE" <- w437
        n271 = case shown="False" w437 {
          tunnel: w436 -> [w498 w502]
          tunnel: [w497 w502] -> w435
          frame False {
            w496 = T16[] [enum."TOGGLE GATE VALVE", enum."RESET TYPE II"] items=["LOOP", "OPEN SERIAL CONN TO ORSAY", "INITIALISE ORSAY", "READ SETTINGS", "SAVE SETTINGS", "OBJECTIVE LENS", "CONDENSOR LENS", "BLANKING TOGGLE", "TURN ON HEATER", "TURN OFF WOBBLER", "MEASURE HEATER OUTPUT", "TOGGLE GATE VALVE", "SCANNING CONTROLS", "TURN ON BEAM HV", "ENERGY RAMP CYCLE", "TURN ON SUPPRESSOR", "TURN ON EXTRACTOR", "TURN ON WIEN FILTER", "SET ENERGY RANGE", "MEASURE HV SUPPLY VOLTAGES", "SHUTDOWN ION SOURCE", "RESET TYPE II", "PROBE CURRENT FC#1", "PROBE CURRENT FC#2", "VACUUM ", "CHECK 150V", "INITIALISE PI MOTORS", "SET STIGMATOR", "SET WOBBLER FOR OBJECT", "SET OBJ & AP STAGE VELOCITIES", "READ APERTURE POSITIONS", "HOME OBJ & AP STAGES", "DEFINE NEW OBJ", "MOVE OBJ STAGES", "DEFINE NEW APERTURE", "MOVE APERTURE STAGES", "STOP SYSTEM", "TEST COMMANDS"]
            n272 = local write "GATE VALVE"(FALSE ("GATE VALVE")) -> ()
            n273 = for {
              shift-right: [w500] -> w497
              shift-left: w498 -> [w501]
              tunnel: w496 -> [w499] mode=indexing
              n274 = Enqueue Element(queue=w501, element=w499) -> (queue out=w500:refnum<queue>)  [unwired: 2 in, 2 out]
            }
            n275 = One Button Dialog(message="FIB Low Vacuum !") -> ()  [unwired: 1 in, 1 out]
          }
          frame True {
          }
        }
        n276 = local write "SERIAL \nRESPONSE"(w434) -> ()
      }
      frame "RESET TYPE II" {
        n277 = local read "APPEND"() -> (w516:string)
        n278 = local read "VISA ERROR"() -> (w519:errorcluster)
        n279 = local read "ORSAY"() -> (w520:refnum<visa-resource-name>)
        n280 = Concatenate Strings("RE 2", w516) -> (w526:string)
        n281 = VISA Write(VISA resource name=w520, write buffer=w526, error in (no error)=w519) -> (VISA resource name out=w530:refnum<visa-resource-name>, error out=w527:errorcluster)  [unwired: 1 out]
        n282 = flat-sequence {
          tunnel: [w538] -> w529
          tunnel: w530 -> [w538]
          tunnel: [w537] -> w528
          tunnel: w527 -> [w537]
          frame #0 {
            n283 = Wait (ms)(milliseconds to wait=u32 200) -> ()  [unwired: 1 out]
          }
        }
        n284 = Build Array (concatenate)(w525, "RESET TYPE II") -> (w523:string[])
        n285 = property class="Instr"(reference=w529, error in=w528) -> (reference out=w533:refnum<visa-resource-name>, error out=w532:errorcluster, "Serial Settings:Number of Bytes at Serial Port"=w531:u32)
        n286 = local write "PROCESSES"(w523) -> ()
        n287 = VISA Read(VISA resource name=w533, byte count=w531, error in (no error)=w532) -> (VISA resource name out=w518:refnum<visa-resource-name>, read buffer=w522:string, error out=w517:errorcluster)  [unwired: 1 out]
        n288 = Build Array (concatenate)(w521, w522) -> (w515:string[])
        n289 = local write "SERIAL \nRESPONSE"(w515) -> ()
        n290 = local write "ORSAY"(w518) -> ()
        n291 = local write "VISA ERROR"(w517) -> ()
      }
      frame "CHECK 150V" {
        # "Should be true for 150V OK"
        # "NOT COMPLETE!!"
        n292 = local read "APPEND"() -> (w541:string)
        n293 = local read "ORSAY"() -> (w565:refnum<visa-resource-name>)
        n294 = Concatenate Strings("GV 15", w541) -> (w554:string)
        n295 = local read "VISA ERROR"() -> (w564:errorcluster)
        n296 = VISA Write(VISA resource name=w565, write buffer=w554, error in (no error)=w564) -> (VISA resource name out=w552:refnum<visa-resource-name>, error out=w550:errorcluster)  [unwired: 1 out]
        n297 = flat-sequence {
          tunnel: [w575] -> w553
          tunnel: w552 -> [w575]
          tunnel: [w574] -> w551
          tunnel: w550 -> [w574]
          frame #0 {
            n298 = Wait (ms)(milliseconds to wait=u32 50) -> ()  [unwired: 1 out]
          }
        }
        n299 = property class="Instr"(reference=w553, error in=w551) -> (reference out=w560:refnum<visa-resource-name>, error out=w558:errorcluster, "Serial Settings:Number of Bytes at Serial Port"=w559:u32)
        n300 = Build Array (concatenate)(w544, "150V CHECK") -> (w543:string[])
        n301 = VISA Read(VISA resource name=w560, byte count=w559, error in (no error)=w558) -> (VISA resource name out=w563:refnum<visa-resource-name>, read buffer=w546:string, error out=w562:errorcluster)  [unwired: 1 out]
        n302 = local write "VISA ERROR"(w562) -> ()
        n303 = local write "PROCESSES"(w543) -> ()
        n304 = local write "ORSAY"(w563) -> ()
        n305 = call <vilib>:"Trim Whitespace.vi"("string"=w546) -> ("trimmed string"=w549:string)  [unwired: 1 in]
        n306 = Match Pattern(string=w549, regular expression=",") -> (after substring=w548:string)  [unwired: 1 in, 3 out]
        n307 = Build Array (concatenate)(w542, w546) -> (w539:string[])
        n308 = Hexadecimal String To Number(string=w548, default (0uL)=i16 0 ("constante")) -> (number=w557:i16)  [unwired: 1 in, 1 out]
        n309 = local write "SERIAL \nRESPONSE"(w539) -> ()
        n310 = Compound Arithmetic op=AND(w557, 64 ("constante")) -> (w570:i32)
        n311 = Compound Arithmetic op=AND(w557, 16 ("constante")) -> (w571:i32)
        n312 = Not Equal To 0?(x=w570) -> (x != 0?=w568:bool)
        n313 = Not Equal To 0?(x=w571) -> (x != 0?=w556:bool)
        n314 = Or(x=w568, y=w556) -> (x .or. y?=w547:bool)
        "150V GOOD" <- w547
        n315 = case shown="True" w547 {
          tunnel: ["150V INTERLOCKED!" ""] -> w561
          frame False {
          }
          frame True {
          }
        }
        n316 = local write "WARNING"(w561) -> ()
      }
      frame "PROBE CURRENT FC#1" {
        w587 = "MEASURE PROBE CURRENT #1"
        w620 = i16 2
        w614 = i16 2
        n317 = local read "VISA ERROR"() -> (w601:errorcluster)
        n318 = local read "ORSAY"() -> (w608:refnum<visa-resource-name>)
        n319 = local read "APPEND"() -> (w583:string)
        n320 = Concatenate Strings("GV 9", w583) -> (w586:string)
        n321 = VISA Write(VISA resource name=w608, write buffer=w586, error in (no error)=w601) -> (VISA resource name out=w599:refnum<visa-resource-name>, error out=w596:errorcluster)  [unwired: 1 out]
        n322 = flat-sequence {
          tunnel: [w638] -> w598
          tunnel: w599 -> [w638]
          tunnel: [w637] -> w597
          tunnel: w596 -> [w637]
          frame #0 {
            n323 = Wait (ms)(milliseconds to wait=u32 200) -> ()  [unwired: 1 out]
          }
        }
        n324 = property class="Instr"(reference=w598, error in=w597) -> (reference out=w613:refnum<visa-resource-name>, error out=w605:errorcluster, "Serial Settings:Number of Bytes at Serial Port"=w612:u32)
        n325 = local read "APPEND"() -> (w581:string)
        n326 = VISA Read(VISA resource name=w613, byte count=w612, error in (no error)=w605) -> (VISA resource name out=w607:refnum<visa-resource-name>, read buffer=w611:string, error out=w606:errorcluster)  [unwired: 1 out]
        n327 = Match Pattern(string=w611, regular expression=",") -> (before substring=w623:string)  [unwired: 1 in, 3 out]
        n328 = Concatenate Strings("GV 8", w581) -> (w584:string)
        n329 = Hexadecimal String To Number(string=w623, offset=w614, default (0uL)=w614) -> (number=w630:i16)  [unwired: 1 out]
        n330 = VISA Write(VISA resource name=w607, write buffer=w584, error in (no error)=w606) -> (VISA resource name out=w595:refnum<visa-resource-name>, error out=w593:errorcluster)  [unwired: 1 out]
        n331 = Divide(x=w630, y=i16 32767) -> (x/y=w624:dbl)
        n332 = Build Array (concatenate)(w588, w587) -> (w589:string[])
        n333 = Less?(x=w630, y=i16 1600) -> (x < y?=w628:bool)
        "gamme" <- w628
        n334 = Multiply(x=w624, y=sgl 21.28) -> (x*y=w625:dbl)
        n335 = local write "PROCESS"(w587) -> ()
        n336 = flat-sequence {
          tunnel: [w635] -> w594
          tunnel: w595 -> [w635]
          tunnel: [w634] -> w592
          tunnel: w593 -> [w634]
          frame #0 {
            n337 = Wait (ms)(milliseconds to wait=u32 100) -> ()  [unwired: 1 out]
          }
        }
        n338 = property class="Instr"(reference=w594, error in=w592) -> (reference out=w610:refnum<visa-resource-name>, error out=w604:errorcluster, "Serial Settings:Number of Bytes at Serial Port"=w609:u32)
        n339 = VISA Read(VISA resource name=w610, byte count=w609, error in (no error)=w604) -> (VISA resource name out=w603:refnum<visa-resource-name>, read buffer=w591:string, error out=w602:errorcluster)  [unwired: 1 out]
        n340 = Match Pattern(string=w591, regular expression=",") -> (before substring=w629:string)  [unwired: 1 in, 3 out]
        n341 = Hexadecimal String To Number(string=w629, offset=w620, default (0uL)=w620) -> (number=w632:i16)  [unwired: 1 out]
        n342 = Negate(x=w632) -> (-x=w631:i16)
        n343 = Divide(x=w631, y=i16 32767) -> (x/y=w626:dbl)
        n344 = Multiply(x=w626, y=sgl 1060.0) -> (x*y=w627:dbl)
        n345 = case shown="True" w628 {
          tunnel: w625 -> [w639 _]
          tunnel: w627 -> [_ w640]
          tunnel: [w639 w640] -> w600
          frame False {
            (unwired) "Probe current (nA)" ("Définir l'attribut")
          }
          frame True {
            (unwired) "Probe current (pA)" ("Définir l'attribut")
          }
        }
        n346 = node(w600) -> (w579:dbl[unit])
        n347 = Build Array (concatenate)(w590, w591) -> (w578:string[])
        n348 = local write "SERIAL \nRESPONSE"(w578) -> ()
        n349 = local write "BEAM CURRENT (FC1)"(w579) -> ()
        n350 = local write "ORSAY"(w603) -> ()
        n351 = local write "VISA ERROR"(w602) -> ()
      }
      frame "PROBE CURRENT FC#2" {
      }
      frame "CONDENSOR LENS" {
        w651 = u16 3 items=["BEAM ENERGY", "EXTRACTOR", "SUPPRESSOR", "CONDENSOR", "OBJECTIVE"] ("HV SUPPLY")
        w656 = "CONDENSOR LENS"
        n352 = local read "CONDENSOR"() -> (w659:cluster{"COARSE":sgl[unit], "FINE":sgl[unit]})
        n353 = Unbundle By Name(w659) -> ("COARSE"=w650:sgl[unit], "FINE"=w649:sgl[unit])
        n354 = local read "VISA ERROR"() -> (w653:errorcluster)
        n355 = local read "ORSAY"() -> (w654:refnum<visa-resource-name>)
        n356 = Add(x=w650, y=w649) -> (x+y=w644:sgl[unit])
        n357 = local read "TIMER"() -> (w646:u32)
        n358 = local write "PROCESS"(w656) -> ()
        n359 = local read "APPEND"() -> (w652:string)
        n360 = call "SET HV SUPPLY MEASURE IV.vi"("ORSAY"=w654, "SETTLE"=w646, "HV SUPPLY"=w651, "VOLTAGE"=w644, "ORSAY ERROR"=w653, "APPEND"=w652) -> ("ORSAY 2"=w648:refnum<visa-resource-name>, "ORSAY ERROR"=w647:errorcluster)  [unwired: 8 in]
        n361 = Build Array (concatenate)(w657, w656) -> (w658:string[])
        n362 = local write "ORSAY"(w648) -> ()
        n363 = local write "VISA ERROR"(w647) -> ()
      }
      frame "SHUTDOWN ION SOURCE" {
        w663 = FALSE ("TURN ON FILAMENT")
        n364 = local write "FILAMENT HEATING"(dbl[unit] 0.0 ("FILAMENT HEATING")) -> ()
        n365 = local write "ION GUN"(w663) -> ()
        n366 = local write "FILAMENT"(w663) -> ()
        n367 = local write "ION GUN SETTINGS"(T19 {"BEAM ENERGY"=0.0, "EXTRACTOR"=0.0, "SUPPRESSOR"=0.0, "ION CURRENT"=0.0} ("ION GUN SETTINGS")) -> ()
      }
      frame "TURN ON HEATER" {
        w671 = "TURN ON HEATER"
        n368 = local read "FILAMENT"() -> (w666:bool)
        n369 = case shown="True" w666 {
          tunnel: ["SH 0,0" w695] -> w669
          frame False {
          }
          frame True {
            n370 = local read "FILAMENT HEATING"() -> (w690:dbl[unit])
            n371 = node(w690) -> (w688:dbl)
            n372 = call "conversion data to bits.vi"("Data input"=w688, "15 /16b"=TRUE, "Max supply"=sgl 5.0) -> ("15 bits output"=w692:u16)  [unwired: 1 out]
            n373 = Number To Hexadecimal String(2:w692) -> (0:w693:string)  [unwired: 1 in]
            n374 = Concatenate Strings("SH ", w693, ",1" ("string")) -> (w695:string)
          }
        }
        n375 = local read "VISA ERROR"() -> (w676:errorcluster)
        n376 = local read "ORSAY"() -> (w677:refnum<visa-resource-name>)
        n377 = VISA Write(VISA resource name=w677, write buffer=w669, error in (no error)=w676) -> (VISA resource name out=w683:refnum<visa-resource-name>, error out=w680:errorcluster)  [unwired: 1 out]
        n378 = flat-sequence {
          tunnel: [w699] -> w682
          tunnel: w683 -> [w699]
          tunnel: [w698] -> w681
          tunnel: w680 -> [w698]
          frame #0 {
            n379 = Wait (ms)(milliseconds to wait=u32 200) -> ()  [unwired: 1 out]
          }
        }
        n380 = property class="Instr"(reference=w682, error in=w681) -> (reference out=w686:refnum<visa-resource-name>, error out=w685:errorcluster, "Serial Settings:Number of Bytes at Serial Port"=w684:u32)
        n381 = VISA Read(VISA resource name=w686, byte count=w684, error in (no error)=w685) -> (VISA resource name out=w679:refnum<visa-resource-name>, read buffer=w675:string, error out=w678:errorcluster)  [unwired: 1 out]
        n382 = local write "ORSAY"(w679) -> ()
        n383 = local write "VISA ERROR"(w678) -> ()
        n384 = local write "PROCESS"(w671) -> ()
        n385 = Build Array (concatenate)(w673, w671) -> (w670:string[])
        n386 = local write "PROCESSES"(w670) -> ()
        n387 = property on="FILAMENT HEATING" class="Slide (strict)"("DisabledEnum"=T18."Enabled" ("Disabled")) -> ()  [unwired: 2 in, 2 out]
        n388 = Build Array (concatenate)(w672, w675) -> (w667:string[])
        n389 = local write "SERIAL \nRESPONSE"(w667) -> ()
      }
      frame "MEASURE HEATER OUTPUT" {
        w720 = T26 0 items=["both", "start of string", "end of string"] ("location (both)")
        w729 = T26 0 items=["both", "start of string", "end of string"] ("location (both)")
        # "SH, 0, 3.8e-4,0,0,0.71e-3"
        n390 = local read "VISA ERROR"() -> (w743:errorcluster)
        n391 = local read "APPEND"() -> (w746:string)
        n392 = local read "ORSAY"() -> (w744:refnum<visa-resource-name>)
        n393 = Concatenate Strings("GV 18" ("string"), w746) -> (w759:string)
        n394 = VISA Write(VISA resource name=w744, write buffer=w759, error in (no error)=w743) -> (VISA resource name out=w763:refnum<visa-resource-name>, error out=w762:errorcluster)  [unwired: 1 out]
        n395 = flat-sequence {
          tunnel: [w774] -> w761
          tunnel: w763 -> [w774]
          tunnel: [w773] -> w760
          tunnel: w762 -> [w773]
          frame #0 {
            n396 = Wait (ms)(milliseconds to wait=u32 100) -> ()  [unwired: 1 out]
          }
        }
        n397 = property class="Instr"(reference=w761, error in=w760) -> (reference out=w766:refnum<visa-resource-name>, error out=w765:errorcluster, "Serial Settings:Number of Bytes at Serial Port"=w764:u32)
        n398 = VISA Read(VISA resource name=w766, byte count=w764, error in (no error)=w765) -> (VISA resource name out=w748:refnum<visa-resource-name>, read buffer=w722:string, error out=w747:errorcluster)  [unwired: 1 out]
        n399 = call <vilib>:"Trim Whitespace.vi"("string"=w722, "location (both)"=w729) -> ("trimmed string"=w728:string)
        n400 = Match Pattern(string=w728, regular expression="FIB>") -> (before substring=w726:string)  [unwired: 1 in, 3 out]
        n401 = Match Pattern(string=w726, regular expression=",") -> (before substring=w723:string)  [unwired: 1 in, 3 out]
        n402 = Hexadecimal String To Number(string=w723, default (0uL)=u16 0 ("default (0 U32)")) -> (number=w721:u16)  [unwired: 1 in, 1 out]
        n403 = To Double Precision Float(number=w721) -> (double precision float=w733:dbl)
        n404 = Multiply(x=w733, y="IGAIN") -> (x*y=w739:dbl)
        n405 = Add(x=w739, y="IOFFSET") -> (x+y=w711:dbl)
        n406 = local read "APPEND"() -> (w745:string)
        n407 = node(w711) -> (w706:dbl[unit])
        "CURRENT" <- w706
        n408 = Concatenate Strings("GV 19" ("string"), w745) -> (w751:string)
        n409 = VISA Write(VISA resource name=w748, write buffer=w751, error in (no error)=w747) -> (VISA resource name out=w755:refnum<visa-resource-name>, error out=w754:errorcluster)  [unwired: 1 out]
        n410 = feedback #1() -> (w702:i32)
        n411 = Increment(x=w702) -> (x+1=w703:i32)
        n412 = feedback-in #1(w703) -> ()
        n413 = flat-sequence {
          tunnel: [w771] -> w753
          tunnel: w755 -> [w771]
          tunnel: [w770] -> w752
          tunnel: w754 -> [w770]
          frame #0 {
            n414 = Wait (ms)(milliseconds to wait=u32 100) -> ()  [unwired: 1 out]
          }
        }
        n415 = Build Array (concatenate)(w732, "MEASURE HEATER OUTPUT") -> (w731:string[])
        n416 = feedback #2() -> (w709:i32[])
        n417 = Build Array (concatenate)(w709, w703) -> (w701:i32[])
        n418 = feedback-in #2(w701) -> ()
        n419 = feedback #3() -> (w707:dbl[unit][])
        n420 = property class="Instr"(reference=w753, error in=w752) -> (reference out=w758:refnum<visa-resource-name>, error out=w757:errorcluster, "Serial Settings:Number of Bytes at Serial Port"=w756:u32)
        n421 = VISA Read(VISA resource name=w758, byte count=w756, error in (no error)=w757) -> (VISA resource name out=w742:refnum<visa-resource-name>, read buffer=w715:string, error out=w741:errorcluster)  [unwired: 1 out]
        n422 = call <vilib>:"Trim Whitespace.vi"("string"=w715, "location (both)"=w720) -> ("trimmed string"=w719:string)
        n423 = Match Pattern(string=w719, regular expression="FIB>") -> (before substring=w717:string)  [unwired: 1 in, 3 out]
        n424 = local write "ORSAY"(w742) -> ()
        n425 = local write "VISA ERROR"(w741) -> ()
        n426 = Match Pattern(string=w717, regular expression=",") -> (before substring=w713:string)  [unwired: 1 in, 3 out]
        n427 = Hexadecimal String To Number(string=w713, default (0uL)=u16 0 ("default (0 U32)")) -> (number=w712:u16)  [unwired: 1 in, 1 out]
        n428 = To Double Precision Float(number=w712) -> (double precision float=w734:dbl)
        n429 = Multiply(x="VGAIN", y=w734) -> (x*y=w735:dbl)
        n430 = Add(x="VOFFSET", y=w735) -> (x+y=w710:dbl)
        n431 = node(w710) -> (w705:dbl[unit])
        "VOLTAGE" <- w705
        n432 = Multiply(x=w706, y=w705) -> (x*y=w708:dbl[unit])
        n433 = Build Array (concatenate)(w707, w708) -> (w704:dbl[unit][])
        n434 = feedback-in #3(w704) -> ()
        n435 = Bundle(w701, w704) -> (→"HEAT POWER":cluster{i32[], dbl[unit][]})  [unwired: 1 in]
      }
      frame "TOGGLE GATE VALVE" {
        n436 = local read "GATE VALVE"() -> (w783:bool)
        n437 = case shown="True" w783 {
          tunnel: ["1" "0"] -> w782
          tunnel: ["OPENING GATE VALVE" "CLOSING GATE VALVE"] -> w781
          frame False {
          }
          frame True {
          }
        }
        n438 = local read "VISA ERROR"() -> (w793:errorcluster)
        n439 = local read "ORSAY"() -> (w792:refnum<visa-resource-name>)
        n440 = local read "APPEND"() -> (w777:string)
        n441 = Concatenate Strings("VC ", w782, w777) -> (w794:string)
        n442 = VISA Write(VISA resource name=w792, write buffer=w794, error in (no error)=w793) -> (VISA resource name out=w788:refnum<visa-resource-name>, error out=w791:errorcluster)  [unwired: 1 out]
        n443 = flat-sequence {
          tunnel: [w804] -> w789
          tunnel: w788 -> [w804]
          tunnel: [w803] -> w790
          tunnel: w791 -> [w803]
          frame #0 {
            n444 = Wait (ms)(milliseconds to wait=u32 200) -> ()  [unwired: 1 out]
          }
        }
        n445 = Build Array (concatenate)(w780, w781) -> (w779:string[])
        n446 = local write "PROCESSES"(w779) -> ()
        n447 = property class="Instr"(reference=w789, error in=w790) -> (reference out=w785:refnum<visa-resource-name>, error out=w786:errorcluster, "Serial Settings:Number of Bytes at Serial Port"=w787:u32)
        n448 = VISA Read(VISA resource name=w785, byte count=w787, error in (no error)=w786) -> (VISA resource name out=w795:refnum<visa-resource-name>, read buffer=w797:string, error out=w796:errorcluster)  [unwired: 1 out]
        n449 = local write "ORSAY"(w795) -> ()
        n450 = local write "VISA ERROR"(w796) -> ()
        n451 = Build Array (concatenate)(w778, w797) -> (w775:string[])
        n452 = local write "SERIAL \nRESPONSE"(w775) -> ()
      }
      frame "OBJECTIVE LENS" {
        w809 = "OBJECTIVE LENS"
        n453 = local read "OBJECTIVE"() -> (w832:cluster{"COARSE":sgl[unit], "FINE":sgl[unit]})
        n454 = Unbundle By Name(w832) -> ("COARSE"=w827:sgl[unit], "FINE"=w826:sgl[unit])
        n455 = node(w827) -> (w824:sgl)
        n456 = node(w826) -> (w825:sgl)
        n457 = Add(x=w824, y=w825) -> (x+y=w823:sgl)
        n458 = local read "VISA ERROR"() -> (w819:errorcluster)
        n459 = call "conversion data to bits.vi"("Data input"=w823, "Max supply"=sgl 20000.0) -> ("15 bits output"=w829:u16)  [unwired: 1 in, 1 out]
        n460 = local write "PROCESS"(w809) -> ()
        n461 = local read "ORSAY"() -> (w834:refnum<visa-resource-name>)
        n462 = Number To Hexadecimal String(2:w829) -> (0:w828:string)  [unwired: 1 in]
        n463 = local read "APPEND"() -> (w807:string)
        n464 = Concatenate Strings("L2 ", w828, w807) -> (w808:string)
        n465 = Build Array (concatenate)(w811, w809) -> (w810:string[])
        n466 = VISA Write(VISA resource name=w834, write buffer=w808, error in (no error)=w819) -> (VISA resource name out=w818:refnum<visa-resource-name>, error out=w817:errorcluster)  [unwired: 1 out]
        n467 = flat-sequence {
          tunnel: [w837] -> w816
          tunnel: w818 -> [w837]
          tunnel: [w836] -> w815
          tunnel: w817 -> [w836]
          frame #0 {
            n468 = Wait (ms)(milliseconds to wait=u32 50) -> ()  [unwired: 1 out]
          }
        }
        n469 = local write "PROCESSES"(w810) -> ()
        n470 = property class="Instr"(reference=w816, error in=w815) -> (reference out=w822:refnum<visa-resource-name>, error out=w821:errorcluster, "Serial Settings:Number of Bytes at Serial Port"=w820:u32)
        n471 = VISA Read(VISA resource name=w822, byte count=w820, error in (no error)=w821) -> (VISA resource name out=w833:refnum<visa-resource-name>, read buffer=w813:string, error out=w814:errorcluster)  [unwired: 1 out]
        n472 = local write "ORSAY"(w833) -> ()
        n473 = local write "VISA ERROR"(w814) -> ()
        n474 = Build Array (concatenate)(w812, w813) -> (w805:string[])
        n475 = local write "SERIAL \nRESPONSE"(w805) -> ()
      }
      frame "SET ENERGY RANGE" {
        # "HIGH energy range (MAX 30kV)"
        # "LOW energy range (MAX 10kV)"
        n476 = local read "HIGH ENERGY"() -> (w839:bool)
        n477 = local read "VISA ERROR"() -> (w856:errorcluster)
        n478 = local read "ORSAY"() -> (w857:refnum<visa-resource-name>)
        n479 = Select(t="RE 3", s=w839, f="RE 4") -> (s? t:f=w850:string)
        n480 = VISA Write(VISA resource name=w857, write buffer=w850, error in (no error)=w856) -> (VISA resource name out=w846:refnum<visa-resource-name>, error out=w845:errorcluster)  [unwired: 1 out]
        n481 = flat-sequence {
          tunnel: [w860] -> w843
          tunnel: w846 -> [w860]
          tunnel: [w859] -> w844
          tunnel: w845 -> [w859]
          frame #0 {
            n482 = Wait (ms)(milliseconds to wait=u32 100) -> ()  [unwired: 1 out]
          }
        }
        n483 = property class="Instr"(reference=w843, error in=w844) -> (reference out=w849:refnum<visa-resource-name>, error out=w848:errorcluster, "Serial Settings:Number of Bytes at Serial Port"=w847:u32)
        n484 = VISA Read(VISA resource name=w849, byte count=w847, error in (no error)=w848) -> (VISA resource name out=w855:refnum<visa-resource-name>, read buffer=w842:string, error out=w854:errorcluster)  [unwired: 1 out]
        n485 = Build Array (concatenate)(w853, w842) -> (w838:string[])
        n486 = local write "SERIAL \nRESPONSE"(w838) -> ()
        n487 = local write "VISA ERROR"(w854) -> ()
        n488 = local write "ORSAY"(w855) -> ()
      }
      frame "TURN ON BEAM HV" {
        w861 = "RAMPING UP/DOWN ION GUN PARAMETERS" ("PROCESS")
        n489 = flat-sequence {
          tunnel: [w870] -> w864
          tunnel: [w869] -> w862
          tunnel: w868 -> [w876]
          tunnel: [w875] -> w867
          tunnel: w864 -> [w871]
          tunnel: w862 -> [w873]
          frame #0 {
            n490 = local read "PREVIOUS GUN SETTINGS"() -> (w869:T1)
            n491 = local read "ION GUN SETTINGS"() -> (w870:T1)
          }
          frame #1 {
            # "New settings"
            n492 = Unbundle By Name(w873) -> ("BEAM ENERGY"=w872:sgl[unit])  [unwired: 3 out]
            n493 = Unbundle By Name(w871) -> ("BEAM ENERGY"=w874:sgl[unit])
            n494 = local write "PREVIOUS GUN SETTINGS"(w871) -> ()
            n495 = stacked-sequence {
              tunnel: w874 -> [w887 _ _]
              tunnel: w876 -> [_ w907 _]
              tunnel: w872 -> [w877 _ _]
              tunnel: [_ w907 _] -> w875
              frame #0 {
                n496 = Subtract(x=w887, y=w877) -> (x-y=w884:sgl[unit])
                n497 = node(w884) -> (w883:sgl)
                n498 = Greater Than 0?(x=w883) -> (x > 0?=w885:bool)
                n499 = case shown="False" w885 {
                  tunnel: [w890 w892] -> w879
                  tunnel: "dV ENERGY" -> [w891 w892]
                  frame False {
                    n500 = Negate(x=w891) -> (-x=w890:dbl[unit])
                  }
                  frame True {
                  }
                }
                n501 = Absolute Value(x=w884) -> (abs(x)=w886:sgl[unit])
                n502 = Divide(x=w886, y=w879) -> (x/y=w889:dbl)
                n503 = Absolute Value(x=w889) -> (abs(x)=w878:dbl)
                n504 = To Long Integer(number=w878) -> (32bit integer=w888:i32)
                n505 = for {
                  N: w888 -> [_]
                  tunnel: w879 -> [w896]
                  tunnel: [w893] -> w880 mode=indexing
                  tunnel: w877 -> [w894]
                  i -> [w898]
                  n506 = Increment(x=w898) -> (x+1=w897:i32)
                  n507 = Multiply(x=w896, y=w897) -> (x*y=w895:dbl[unit])
                  n508 = Add(x=w894, y=w895) -> (x+y=w893:dbl[unit])
                }
                "BEAM RAMP" <- w880
                n509 = local write "BEAM RAMP"(w880) -> ()
                n510 = Array Size(array=w880) -> (size(s)=→"size(s)":i32)
              }
              frame #1 {
                n511 = local read "BEAM RAMP"() -> (w900:dbl[unit][])
                n512 = Array Size(array=w900) -> (size(s)=w899:i32)
                n513 = local read "VISA ERROR"() -> (w905:errorcluster)
                n514 = local read "ORSAY"() -> (w906:refnum<visa-resource-name>)
                n515 = local read "TIMER"() -> (w904:u32)
                n516 = Not Equal To 0?(x=w899) -> (x != 0?=w901:bool)
                n517 = case shown="True" w901 {
                  tunnel: w906 -> [w909 w915]
                  tunnel: w905 -> [w908 w914]
                  tunnel: w904 -> [_ w913]
                  tunnel: [w909 w912] -> w903
                  tunnel: w900 -> [_ w910]
                  tunnel: [w908 w911] -> w902
                  frame False {
                  }
                  frame True {
                    n518 = for {
                      shift-right: [w930] -> w912
                      shift-left: w915 -> [w939]
                      shift-right: [w927] -> w911
                      shift-left: w914 -> [w938]
                      tunnel: w913 -> [w937]
                      tunnel: w910 -> [w934] mode=indexing
                      w925 = u16 2 items=["BEAM ENERGY", "EXTRACTOR", "SUPPRESSOR", "CONDENSOR", "OBJECTIVE"] ("HV SUPPLY")
                      w926 = u16 1 items=["BEAM ENERGY", "EXTRACTOR", "SUPPRESSOR", "CONDENSOR", "OBJECTIVE"] ("HV SUPPLY")
                      w933 = u16 0 items=["BEAM ENERGY", "EXTRACTOR", "SUPPRESSOR", "CONDENSOR", "OBJECTIVE"] ("HV SUPPLY")
                      n519 = local read "APPEND"() -> (w922:string)
                      n520 = call "SET HV SUPPLY MEASURE IV.vi"("ORSAY"=w939, "SETTLE"=w937, "HV SUPPLY"=w933, "VOLTAGE"=w934, "ORSAY ERROR"=w938, "APPEND"=w922) -> ("ORSAY 2"=w936:refnum<visa-resource-name>, "ORSAY ERROR"=w935:errorcluster)  [unwired: 8 in]
                      n521 = call "READ HV SUPPLIES.vi"("ORSAY"=w936, "HV SUPPLY"=w933, "ORSAY ERROR"=w935, "APPEND"=w922) -> ("ORSAY 2"=w932:refnum<visa-resource-name>, "VOLTAGE"=w917:dbl[unit], "CURRENT"=w916:dbl[unit], "ORSAY ERROR"=w929:errorcluster)  [unwired: 8 in]
                      n522 = local write "CURRENT"(w916) -> ()
                      n523 = local write "VOLTAGE"(w917) -> ()
                      n524 = local write "BEAM VOLTAGE"(w917) -> ()
                      n525 = local write "BEAM CURRENT"(w916) -> ()
                      n526 = call "READ HV SUPPLIES.vi"("ORSAY"=w932, "HV SUPPLY"=w926, "ORSAY ERROR"=w929, "APPEND"=w922) -> ("ORSAY 2"=w931:refnum<visa-resource-name>, "VOLTAGE"=w919:dbl[unit], "CURRENT"=w924:dbl[unit], "ORSAY ERROR"=w928:errorcluster)  [unwired: 8 in]
                      n527 = call "READ HV SUPPLIES.vi"("ORSAY"=w931, "HV SUPPLY"=w925, "ORSAY ERROR"=w928, "APPEND"=w922) -> ("ORSAY 2"=w930:refnum<visa-resource-name>, "VOLTAGE"=w920:dbl[unit], "CURRENT"=w923:dbl[unit], "ORSAY ERROR"=w927:errorcluster)  [unwired: 8 in]
                      n528 = Bundle By Name(cluster=T21 {"BEAM"=0.0, "SUPPRESSOR"=0.0, "EXTRACTOR"=0.0} ("HIGH VOLTAGE SUPPLIES"), "BEAM"=w917, "SUPPRESSOR"=w920, "EXTRACTOR"=w919) -> (w921:T21)
                      n529 = local write "HIGH VOLTAGE SUPPLIES"(w921) -> ()
                      n530 = local write "EXTRACTOR  CURRENT"(w924) -> ()
                      n531 = local write "EXTRACTOR"(w919) -> ()
                      n532 = local write "SUPPRESSOR CURRENT"(w923) -> ()
                      n533 = local write "SUPPRESSOR VOLTAGE"(w920) -> ()
                    }
                  }
                }
                n534 = local write "VISA ERROR"(w902) -> ()
                n535 = local write "ORSAY"(w903) -> ()
              }
              frame #2 {
                n536 = property on="SUPPRESSOR" class="Slide (strict)"("DisabledEnum"=T18."Enabled" ("Disabled")) -> ()  [unwired: 2 in, 2 out]
              }
            }
          }
        }
        n537 = local write "PROCESS"(w861) -> ()
        n538 = Build Array (concatenate)(w866, w861) -> (w865:string[])
        n539 = local write "PROCESSES"(w865) -> ()
      }
      frame "ENERGY RAMP CYCLE" {
        n540 = while {
          tunnel: dbl[unit][] [500.0, 1000.0, 1500.0, 2000.0, 2500.0, 3000.0, 3500.0, 4000.0, 4500.0, 5000.0, 4500.0, 4000.0, 3500.0, 3000.0, 2500.0, 2000.0, 1500.0, 1000.0, 500.0, 0.0] -> [w947]
          stop <- w945 continue-if-true
          n541 = local read "VISA ERROR"() -> (w951:errorcluster)
          n542 = local read "TIMER"() -> (w948:u32)
          n543 = local read "ORSAY"() -> (w952:refnum<visa-resource-name>)
          n544 = Array Size(array=w947) -> (size(s)=w946:i32)
          n545 = for {
            N: w946 -> [_]
            shift-right: [w957] -> w950
            shift-left: w952 -> [w964]
            shift-right: [w955] -> w949
            shift-left: w951 -> [w963]
            tunnel: w948 -> [w962]
            tunnel: w947 -> [w953] mode=indexing
            w958 = u16 0 items=["BEAM ENERGY", "EXTRACTOR", "SUPPRESSOR", "CONDENSOR", "OBJECTIVE"] ("HV SUPPLY")
            n546 = local read "APPEND"() -> (w959:string)
            n547 = call "SET HV SUPPLY MEASURE IV.vi"("ORSAY"=w964, "SETTLE"=w962, "HV SUPPLY"=w958, "VOLTAGE"=w953, "ORSAY ERROR"=w963, "APPEND"=w959) -> ("ORSAY 2"=w961:refnum<visa-resource-name>, "ORSAY ERROR"=w960:errorcluster)  [unwired: 8 in]
            n548 = call "READ HV SUPPLIES.vi"("ORSAY"=w961, "HV SUPPLY"=w958, "ORSAY ERROR"=w960, "APPEND"=w959) -> ("ORSAY 2"=w956:refnum<visa-resource-name>, "ORSAY ERROR"=w954:errorcluster)  [unwired: 8 in, 2 out]
            n549 = flat-sequence {
              tunnel: [w966] -> w957
              tunnel: w956 -> [w966]
              tunnel: [w965] -> w955
              tunnel: w954 -> [w965]
              frame #0 {
                n550 = Wait (ms)(milliseconds to wait=u32 100) -> ()  [unwired: 1 out]
              }
            }
          }
          n551 = local read "1V ENERGY RAMP"() -> (w945:bool)
          n552 = local write "ORSAY"(w950) -> ()
          n553 = local write "VISA ERROR"(w949) -> ()
        }
      }
      frame "TURN ON SUPPRESSOR" {
        w969 = "RAMPING UP/DOWN SUPPRESSOR" ("PROCESS")
        n554 = flat-sequence {
          tunnel: [w977] -> w971
          tunnel: [w976] -> w968
          tunnel: w975 -> [w983]
          tunnel: [w982] -> w974
          tunnel: w971 -> [w979]
          tunnel: w968 -> [w980]
          frame #0 {
            n555 = local read "PREVIOUS GUN SETTINGS"() -> (w976:T1)
            n556 = local read "ION GUN SETTINGS"() -> (w977:T1)
          }
          frame #1 {
            # "New settings"
            n557 = Unbundle By Name(w980) -> ("SUPPRESSOR"=w978:sgl[unit])  [unwired: 3 out]
            n558 = local write "PREVIOUS GUN SETTINGS"(w979) -> ()
            n559 = Unbundle By Name(w979) -> ("SUPPRESSOR"=w981:sgl[unit])
            n560 = stacked-sequence {
              tunnel: w981 -> [w986 _ _]
              tunnel: w983 -> [_ w1014 _]
              tunnel: w978 -> [w984 _ _]
              tunnel: [_ w1014 _] -> w982
              frame #0 {
                # "S-E=Seffective"
                n561 = Subtract(x=w986, y=w984) -> (x-y=w985:sgl[unit])
                n562 = node(w985) -> (w993:sgl)
                n563 = Greater Than 0?(x=w993) -> (x > 0?=w992:bool)
                n564 = case shown="False" w992 {
                  tunnel: [w998 w999] -> w990
                  tunnel: "dV SUPPRESS" -> [w997 w999]
                  frame False {
                    n565 = Negate(x=w997) -> (-x=w998:dbl[unit])
                  }
                  frame True {
                  }
                }
                n566 = Absolute Value(x=w985) -> (abs(x)=w994:sgl[unit])
                n567 = Divide(x=w994, y=w990) -> (x/y=w996:dbl)
                n568 = Absolute Value(x=w996) -> (abs(x)=w989:dbl)
                n569 = To Long Integer(number=w989) -> (32bit integer=w995:i32)
                n570 = for {
                  N: w995 -> [_]
                  tunnel: w990 -> [w1004]
                  tunnel: [w1002] -> w987 mode=indexing
                  tunnel: w984 -> [w1001]
                  i -> [w1005]
                  n571 = Increment(x=w1005) -> (x+1=w1003:i32)
                  n572 = Multiply(x=w1004, y=w1003) -> (x*y=w1000:dbl[unit])
                  n573 = Add(x=w1001, y=w1000) -> (x+y=w1002:dbl[unit])
                }
                "SUPPRESSOR RAMP" <- w987
                n574 = local write "SUPPRESSOR RAMP"(w987) -> ()
                n575 = Array Size(array=w987) -> (size(s)=→"size(s) 4":i32)
              }
              frame #1 {
                n576 = local read "SUPPRESSOR RAMP"() -> (w1007:dbl[unit][])
                n577 = Array Size(array=w1007) -> (size(s)=w1006:i32)
                n578 = local read "VISA ERROR"() -> (w1012:errorcluster)
                n579 = local read "ORSAY"() -> (w1013:refnum<visa-resource-name>)
                n580 = local read "TIMER"() -> (w1011:u32)
                n581 = Not Equal To 0?(x=w1006) -> (x != 0?=w1008:bool)
                n582 = case shown="True" w1008 {
                  tunnel: w1013 -> [w1016 w1022]
                  tunnel: w1012 -> [w1015 w1021]
                  tunnel: w1011 -> [_ w1020]
                  tunnel: [w1016 w1019] -> w1010
                  tunnel: w1007 -> [_ w1017]
                  tunnel: [w1015 w1018] -> w1009
                  frame False {
                  }
                  frame True {
                    n583 = for {
                      shift-right: [w1032] -> w1019
                      shift-left: w1022 -> [w1046]
                      shift-right: [w1031] -> w1018
                      shift-left: w1021 -> [w1045]
                      tunnel: w1020 -> [w1044]
                      tunnel: w1017 -> [w1041] mode=indexing
                      w1033 = u16 1 items=["BEAM ENERGY", "EXTRACTOR", "SUPPRESSOR", "CONDENSOR", "OBJECTIVE"] ("HV SUPPLY")
                      w1037 = u16 0 items=["BEAM ENERGY", "EXTRACTOR", "SUPPRESSOR", "CONDENSOR", "OBJECTIVE"] ("HV SUPPLY")
                      w1040 = u16 2 items=["BEAM ENERGY", "EXTRACTOR", "SUPPRESSOR", "CONDENSOR", "OBJECTIVE"] ("HV SUPPLY")
                      n584 = local read "APPEND"() -> (w1034:string)
                      n585 = call "SET HV SUPPLY MEASURE IV.vi"("ORSAY"=w1046, "SETTLE"=w1044, "HV SUPPLY"=w1040, "VOLTAGE"=w1041, "ORSAY ERROR"=w1045, "APPEND"=w1034) -> ("ORSAY 2"=w1043:refnum<visa-resource-name>, "ORSAY ERROR"=w1042:errorcluster)  [unwired: 8 in]
                      n586 = call "READ HV SUPPLIES.vi"("ORSAY"=w1043, "HV SUPPLY"=w1040, "ORSAY ERROR"=w1042, "APPEND"=w1034) -> ("ORSAY 2"=w1039:refnum<visa-resource-name>, "VOLTAGE"=w1023:dbl[unit], "CURRENT"=w1024:dbl[unit], "ORSAY ERROR"=w1038:errorcluster)  [unwired: 8 in]
                      n587 = local write "VOLTAGE"(w1023) -> ()
                      n588 = local write "CURRENT"(w1024) -> ()
                      n589 = local write "SUPPRESSOR CURRENT"(w1024) -> ()
                      n590 = local write "SUPPRESSOR VOLTAGE"(w1023) -> ()
                      n591 = call "READ HV SUPPLIES.vi"("ORSAY"=w1039, "HV SUPPLY"=w1037, "ORSAY ERROR"=w1038, "APPEND"=w1034) -> ("ORSAY 2"=w1036:refnum<visa-resource-name>, "VOLTAGE"=w1028:dbl[unit], "CURRENT"=w1030:dbl[unit], "ORSAY ERROR"=w1035:errorcluster)  [unwired: 8 in]
                      n592 = local write "BEAM CURRENT"(w1030) -> ()
                      n593 = local write "BEAM VOLTAGE"(w1028) -> ()
                      n594 = call "READ HV SUPPLIES.vi"("ORSAY"=w1036, "HV SUPPLY"=w1033, "ORSAY ERROR"=w1035, "APPEND"=w1034) -> ("ORSAY 2"=w1032:refnum<visa-resource-name>, "VOLTAGE"=w1026:dbl[unit], "CURRENT"=w1029:dbl[unit], "ORSAY ERROR"=w1031:errorcluster)  [unwired: 8 in]
                      n595 = local write "EXTRACTOR  CURRENT"(w1029) -> ()
                      n596 = local write "EXTRACTOR"(w1026) -> ()
                      n597 = Bundle By Name(cluster=T21 {"BEAM"=0.0, "SUPPRESSOR"=0.0, "EXTRACTOR"=0.0} ("HIGH VOLTAGE SUPPLIES"), "BEAM"=w1028, "SUPPRESSOR"=w1023, "EXTRACTOR"=w1026) -> (w1027:T21)
                      n598 = local write "HIGH VOLTAGE SUPPLIES"(w1027) -> ()
                    }
                  }
                }
                n599 = local write "VISA ERROR"(w1009) -> ()
                n600 = local write "ORSAY"(w1010) -> ()
              }
              frame #2 {
                n601 = property on="EXTRACTOR" class="Slide (strict)"("DisabledEnum"=T18."Enabled" ("Disabled")) -> ()  [unwired: 2 in, 2 out]
              }
            }
          }
        }
        n602 = local write "PROCESS"(w969) -> ()
        n603 = Build Array (concatenate)(w973, w969) -> (w972:string[])
        n604 = local write "PROCESSES"(w972) -> ()
      }
      frame "TURN ON EXTRACTOR" {
        w1049 = "RAMPING UP/DOWN SUPPRESSOR" ("PROCESS")
        n605 = flat-sequence {
          tunnel: [w1057] -> w1051
          tunnel: [w1056] -> w1048
          tunnel: w1055 -> [w1063]
          tunnel: [w1062] -> w1054
          tunnel: w1051 -> [w1058]
          tunnel: w1048 -> [w1060]
          frame #0 {
            n606 = local read "PREVIOUS GUN SETTINGS"() -> (w1056:T1)
            n607 = local read "ION GUN SETTINGS"() -> (w1057:T1)
          }
          frame #1 {
            # "New settings"
            n608 = local write "PREVIOUS GUN SETTINGS"(w1058) -> ()
            n609 = Unbundle By Name(w1060) -> ("EXTRACTOR"=w1059:sgl[unit])  [unwired: 3 out]
            n610 = Unbundle By Name(w1058) -> ("EXTRACTOR"=w1061:sgl[unit])
            n611 = stacked-sequence {
              tunnel: w1061 -> [w1065 _ _]
              tunnel: w1063 -> [_ w1094 _]
              tunnel: w1059 -> [w1064 _ _]
              tunnel: [_ w1094 _] -> w1062
              frame #0 {
                n612 = Subtract(x=w1065, y=w1064) -> (x-y=w1071:sgl[unit])
                n613 = node(w1071) -> (w1073:sgl)
                n614 = Greater Than 0?(x=w1073) -> (x > 0?=w1072:bool)
                n615 = case shown="False" w1072 {
                  tunnel: [w1078 w1079] -> w1069
                  tunnel: "dV EXTRACTOR" -> [w1077 w1079]
                  frame False {
                    n616 = Negate(x=w1077) -> (-x=w1078:dbl[unit])
                  }
                  frame True {
                  }
                }
                n617 = Absolute Value(x=w1071) -> (abs(x)=w1074:sgl[unit])
                n618 = Divide(x=w1074, y=w1069) -> (x/y=w1076:dbl)
                n619 = Absolute Value(x=w1076) -> (abs(x)=w1068:dbl)
                n620 = To Long Integer(number=w1068) -> (32bit integer=w1075:i32)
                n621 = for {
                  N: w1075 -> [_]
                  tunnel: w1069 -> [w1084]
                  tunnel: [w1082] -> w1066 mode=indexing
                  tunnel: w1064 -> [w1081]
                  i -> [w1085]
                  n622 = Increment(x=w1085) -> (x+1=w1083:i32)
                  n623 = Multiply(x=w1084, y=w1083) -> (x*y=w1080:dbl[unit])
                  n624 = Add(x=w1081, y=w1080) -> (x+y=w1082:dbl[unit])
                }
                n625 = local write "EXTRACTOR RAMP"(w1066) -> ()
                n626 = local write "EXTRACTOR RAMP"(w1066) -> ()
                n627 = Array Size(array=w1066) -> (size(s)=→"size(s) 5":i32)
              }
              frame #1 {
                n628 = local read "EXTRACTOR RAMP"() -> (w1086:dbl[unit][])
                n629 = Array Size(array=w1086) -> (size(s)=w1087:i32)
                n630 = local read "VISA ERROR"() -> (w1092:errorcluster)
                n631 = local read "ORSAY"() -> (w1093:refnum<visa-resource-name>)
                n632 = local read "TIMER"() -> (w1091:u32)
                n633 = Not Equal To 0?(x=w1087) -> (x != 0?=w1088:bool)
                n634 = case shown="True" w1088 {
                  tunnel: w1093 -> [w1096 w1102]
                  tunnel: w1092 -> [w1095 w1101]
                  tunnel: w1091 -> [_ w1100]
                  tunnel: [w1096 w1099] -> w1090
                  tunnel: w1086 -> [_ w1097]
                  tunnel: [w1095 w1098] -> w1089
                  frame False {
                  }
                  frame True {
                    n635 = for {
                      shift-right: [w1115] -> w1099
                      shift-left: w1102 -> [w1126]
                      shift-right: [w1113] -> w1098
                      shift-left: w1101 -> [w1125]
                      tunnel: w1100 -> [w1124]
                      tunnel: w1097 -> [w1121] mode=indexing
                      w1110 = u16 0 items=["BEAM ENERGY", "EXTRACTOR", "SUPPRESSOR", "CONDENSOR", "OBJECTIVE"] ("HV SUPPLY")
                      w1111 = u16 2 items=["BEAM ENERGY", "EXTRACTOR", "SUPPRESSOR", "CONDENSOR", "OBJECTIVE"] ("HV SUPPLY")
                      w1120 = u16 1 items=["BEAM ENERGY", "EXTRACTOR", "SUPPRESSOR", "CONDENSOR", "OBJECTIVE"] ("HV SUPPLY")
                      n636 = local read "APPEND"() -> (w1112:string)
                      n637 = call "SET HV SUPPLY MEASURE IV.vi"("ORSAY"=w1126, "SETTLE"=w1124, "HV SUPPLY"=w1120, "VOLTAGE"=w1121, "ORSAY ERROR"=w1125, "APPEND"=w1112) -> ("ORSAY 2"=w1123:refnum<visa-resource-name>, "ORSAY ERROR"=w1122:errorcluster)  [unwired: 8 in]
                      n638 = call "READ HV SUPPLIES.vi"("ORSAY"=w1123, "HV SUPPLY"=w1120, "ORSAY ERROR"=w1122, "APPEND"=w1112) -> ("ORSAY 2"=w1118:refnum<visa-resource-name>, "VOLTAGE"=w1106:dbl[unit], "CURRENT"=w1119:dbl[unit], "ORSAY ERROR"=w1117:errorcluster)  [unwired: 8 in]
                      n639 = local write "EXTRACTOR"(w1106) -> ()
                      n640 = local write "EXTRACTOR  CURRENT"(w1119) -> ()
                      n641 = call "READ HV SUPPLIES.vi"("ORSAY"=w1118, "HV SUPPLY"=w1110, "ORSAY ERROR"=w1117, "APPEND"=w1112) -> ("ORSAY 2"=w1116:refnum<visa-resource-name>, "VOLTAGE"=w1103:dbl[unit], "CURRENT"=w1104:dbl[unit], "ORSAY ERROR"=w1114:errorcluster)  [unwired: 8 in]
                      n642 = local write "VOLTAGE"(w1103) -> ()
                      n643 = local write "CURRENT"(w1104) -> ()
                      n644 = local write "BEAM CURRENT"(w1104) -> ()
                      n645 = local write "BEAM VOLTAGE"(w1103) -> ()
                      n646 = call "READ HV SUPPLIES.vi"("ORSAY"=w1116, "HV SUPPLY"=w1111, "ORSAY ERROR"=w1114, "APPEND"=w1112) -> ("ORSAY 2"=w1115:refnum<visa-resource-name>, "VOLTAGE"=w1107:dbl[unit], "CURRENT"=w1109:dbl[unit], "ORSAY ERROR"=w1113:errorcluster)  [unwired: 8 in]
                      n647 = Bundle By Name(cluster=T21 {"BEAM"=0.0, "SUPPRESSOR"=0.0, "EXTRACTOR"=0.0} ("HIGH VOLTAGE SUPPLIES"), "BEAM"=w1103, "SUPPRESSOR"=w1107, "EXTRACTOR"=w1106) -> (w1108:T21)
                      n648 = local write "HIGH VOLTAGE SUPPLIES"(w1108) -> ()
                      n649 = local write "SUPPRESSOR CURRENT"(w1109) -> ()
                      n650 = local write "SUPPRESSOR VOLTAGE"(w1107) -> ()
                    }
                  }
                }
                n651 = local write "VISA ERROR"(w1089) -> ()
                n652 = local write "ORSAY"(w1090) -> ()
              }
              frame #2 {
                n653 = property on="EXTRACTOR" class="Slide (strict)"("DisabledEnum"=T18."Enabled" ("Disabled")) -> ()  [unwired: 2 in, 2 out]
              }
            }
          }
        }
        n654 = local write "PROCESS"(w1049) -> ()
        n655 = Build Array (concatenate)(w1053, w1049) -> (w1052:string[])
        n656 = local write "PROCESSES"(w1052) -> ()
      }
      frame "TURN ON WIEN FILTER" {
        w1152 = 9.999999747378752e-06 ("f")
        w1157 = dbl[unit] 30000.0  # kV
        n657 = local read "ION GUN SETTINGS"() -> (w1159:T1)
        n658 = Unbundle By Name("E&B") -> ("M-COARSE"=w1160:sgl, "M-FINE"=w1161:sgl, "ELECTRIC FIELD"=w1151:sgl)
        n659 = Unbundle By Name(w1159) -> ("BEAM ENERGY"=w1158:sgl[unit])
        n660 = Divide(x=w1158, y=w1157) -> (x/y=w1156:dbl)
        n661 = Square Root(x=w1156) -> (sqrt(x)=w1154:dbl)
        n662 = Add(x=w1160, y=w1161) -> (x+y=w1155:sgl)
        n663 = Multiply(x=w1155, y=w1154) -> (x*y=w1148:dbl)
        n664 = local read "WIEN"() -> (w1153:bool)
        n665 = local read "VISA ERROR"() -> (w1137:errorcluster)
        n666 = Less Than 0?(x=w1148) -> (x < 0?=w1150:bool)
        n667 = local read "ORSAY"() -> (w1138:refnum<visa-resource-name>)
        n668 = case shown="True" w1150 {
          tunnel: [w1171 0.0] -> w1149
          tunnel: w1148 -> [w1171 _]
          frame False {
          }
          frame True {
          }
        }
        n669 = Select(t=w1149, s=w1153, f=w1152) -> (s? t:f=w1144:dbl)
        n670 = Select(t=w1151, s=w1153, f=w1152) -> (s? t:f=w1143:dbl)
        n671 = flat-sequence {
          tunnel: w1167 -> [w1173]
          tunnel: [w1175] -> w1170
          tunnel: w1168 -> [w1175]
          tunnel: [w1173] -> w1169
          frame #0 {
            n672 = Wait (ms)(milliseconds to wait=u32 100) -> ()  [unwired: 1 out]
          }
        }
        n673 = call "conversion data to bits.vi"("Data input"=w1144, "Max supply"=2.0) -> ("15 bits output"=w1142:u16)  [unwired: 1 in, 1 out]
        n674 = call "conversion data to bits.vi"("Data input"=w1143, "15 /16b"=TRUE, "Max supply"=150.0) -> ("15 bits output"=w1141:u16)  [unwired: 1 out]
        n675 = Number To Hexadecimal String(2:w1142) -> (0:w1135:string)  [unwired: 1 in]
        n676 = Number To Hexadecimal String(2:w1141) -> (0:w1133:string)  [unwired: 1 in]
        n677 = Concatenate Strings(w1135, ",1", ",", w1133) -> (w1132:string)
        n678 = Concatenate Strings("WF " ("string"), w1132) -> (w1131:string)
        n679 = VISA Write(VISA resource name=w1138, write buffer=w1131, error in (no error)=w1137) -> (VISA resource name out=w1167:refnum<visa-resource-name>, error out=w1168:errorcluster)  [unwired: 1 out]
        n680 = property class="Instr"(reference=w1169, error in=w1170) -> (reference out=w1166:refnum<visa-resource-name>, error out=w1164:errorcluster, "Serial Settings:Number of Bytes at Serial Port"=w1165:u32)
        n681 = VISA Read(VISA resource name=w1166, byte count=w1165, error in (no error)=w1164) -> (VISA resource name out=w1140:refnum<visa-resource-name>, error out=w1139:errorcluster)  [unwired: 2 out]
        n682 = local write "VISA ERROR"(w1139) -> ()
        n683 = local write "ORSAY"(w1140) -> ()
      }
      frame "TURN OFF WOBBLER" {
        n684 = flat-sequence {
          frame #0 {
            n685 = local read "APPEND"() -> (w1188:string)
            n686 = Concatenate Strings("WB 0" ("string"), w1188) -> (w1180:string)
            n687 = local read "VISA ERROR"() -> (w1189:errorcluster)
            n688 = local read "ORSAY"() -> (w1190:refnum<visa-resource-name>)
            n689 = VISA Write(VISA resource name=w1190, write buffer=w1180, error in (no error)=w1189) -> (VISA resource name out=w1184:refnum<visa-resource-name>, error out=w1183:errorcluster)  [unwired: 1 out]
            n690 = flat-sequence {
              tunnel: w1184 -> [w1193]
              tunnel: [w1195] -> w1181
              tunnel: w1183 -> [w1195]
              tunnel: [w1193] -> w1182
              frame #0 {
                n691 = Wait (ms)(milliseconds to wait=u32 100) -> ()  [unwired: 1 out]
              }
            }
            n692 = property class="Instr"(reference=w1182, error in=w1181) -> (reference out=w1185:refnum<visa-resource-name>, error out=w1187:errorcluster, "Serial Settings:Number of Bytes at Serial Port"=w1186:u32)
            n693 = VISA Read(VISA resource name=w1185, byte count=w1186, error in (no error)=w1187) -> (VISA resource name out=w1192:refnum<visa-resource-name>, error out=w1191:errorcluster)  [unwired: 2 out]
            n694 = local write "ORSAY"(w1192) -> ()
            n695 = local write "VISA ERROR"(w1191) -> ()
          }
          frame #1 {
          }
        }
      }
      frame "STOP SYSTEM" {
        n696 = flat-sequence {
          frame #0 {
            n697 = local read "VISA ERROR"() -> (w1199:errorcluster)
            n698 = local read "ORSAY"() -> (w1200:refnum<visa-resource-name>)
            n699 = VISA Close(VISA resource name=w1200, error in (no error)=w1199) -> ()  [unwired: 1 out]
          }
          frame #1 {
            n700 = Stop(stop? (T)=TRUE) -> ()
          }
        }
      }
      frame "MEASURE HV SUPPLY VOLTAGES" {
        w1218 = u16 4 items=["BEAM ENERGY", "EXTRACTOR", "SUPPRESSOR", "CONDENSOR", "OBJECTIVE"] ("HV SUPPLY")
        w1219 = u16 3 items=["BEAM ENERGY", "EXTRACTOR", "SUPPRESSOR", "CONDENSOR", "OBJECTIVE"] ("HV SUPPLY")
        w1222 = u16 2 items=["BEAM ENERGY", "EXTRACTOR", "SUPPRESSOR", "CONDENSOR", "OBJECTIVE"] ("HV SUPPLY")
        w1223 = u16 1 items=["BEAM ENERGY", "EXTRACTOR", "SUPPRESSOR", "CONDENSOR", "OBJECTIVE"] ("HV SUPPLY")
        w1224 = u16 0 items=["BEAM ENERGY", "EXTRACTOR", "SUPPRESSOR", "CONDENSOR", "OBJECTIVE"] ("HV SUPPLY")
        w1234 = "MEASURING ION GUN HV" ("PROCESS")
        n701 = local read "ORSAY"() -> (w1229:refnum<visa-resource-name>)
        n702 = local read "APPEND"() -> (w1214:string)
        n703 = call "READ HV SUPPLIES.vi"("ORSAY"=w1229, "HV SUPPLY"=w1224, "APPEND"=w1214) -> ("ORSAY 2"=w1226:refnum<visa-resource-name>, "VOLTAGE"=w1211:dbl[unit], "CURRENT"=→"BEAM CURRENT" →"CURRENT":dbl[unit], "ORSAY ERROR"=w1228:errorcluster)  [unwired: 9 in]
        "BEAM VOLTAGE" <- w1211
        "VOLTAGE" <- w1211
        n704 = call "READ HV SUPPLIES.vi"("ORSAY"=w1226, "HV SUPPLY"=w1223, "ORSAY ERROR"=w1228, "APPEND"=w1214) -> ("ORSAY 2"=w1225:refnum<visa-resource-name>, "VOLTAGE"=w1203:dbl[unit], "CURRENT"=→"EXTRACTOR  CURRENT" →"CURRENT":dbl[unit], "ORSAY ERROR"=w1227:errorcluster)  [unwired: 8 in]
        "EXTRACTOR" <- w1203
        "VOLTAGE" <- w1203
        n705 = call "READ HV SUPPLIES.vi"("ORSAY"=w1225, "HV SUPPLY"=w1222, "ORSAY ERROR"=w1227, "APPEND"=w1214) -> ("ORSAY 2"=w1221:refnum<visa-resource-name>, "VOLTAGE"=w1202:dbl[unit], "CURRENT"=→"SUPPRESSOR CURRENT" →"CURRENT":dbl[unit], "ORSAY ERROR"=w1215:errorcluster)  [unwired: 8 in]
        "SUPPRESSOR VOLTAGE" <- w1202
        "VOLTAGE" <- w1202
        n706 = local write "PROCESS"(w1234) -> ()
        n707 = Build Array (concatenate)(w1233, w1234) -> (w1232:string[])
        n708 = call "READ HV SUPPLIES.vi"("ORSAY"=w1221, "HV SUPPLY"=w1219, "ORSAY ERROR"=w1215, "APPEND"=w1214) -> ("ORSAY 2"=w1220:refnum<visa-resource-name>, "VOLTAGE"=→"CONDENSOR VOLTAGE":dbl[unit], "CURRENT"=→"CONDENSOR CURRENT":dbl[unit], "ORSAY ERROR"=w1216:errorcluster)  [unwired: 8 in]
        n709 = Bundle By Name(cluster=T21 {"BEAM"=0.0, "SUPPRESSOR"=0.0, "EXTRACTOR"=0.0} ("HIGH VOLTAGE SUPPLIES"), "BEAM"=w1211, "SUPPRESSOR"=w1202, "EXTRACTOR"=w1203) -> (→"HIGH VOLTAGE SUPPLIES":T21)
        n710 = local write "PROCESSES"(w1232) -> ()
        n711 = call "READ HV SUPPLIES.vi"("ORSAY"=w1220, "HV SUPPLY"=w1218, "ORSAY ERROR"=w1216, "APPEND"=w1214) -> ("ORSAY 2"=w1217:refnum<visa-resource-name>, "VOLTAGE"=→"OBJECTIVE VOLTAGE":dbl[unit], "CURRENT"=→"OBJECTIVE CURRENT":dbl[unit])  [unwired: 8 in, 1 out]
        n712 = local write "ORSAY"(w1217) -> ()
      }
      frame "SCANNING CONTROLS" {
        w1239 = "SCANNING CONTROL" ("PROCESS")
        n713 = Unbundle By Name("SCANNING CLUSTER") -> ("X-OFFSET"=w1265:sgl[unit], "Y-OFFSET"=w1264:sgl[unit], "ROTATION"=w1263:dbl[unit])  [unwired: 1 out]
        n714 = node(w1265) -> (w1261:sgl)
        n715 = node(w1264) -> (w1258:sgl)
        n716 = node(w1263) -> (w1257:dbl)
        n717 = local read "ORSAY"() -> (w1243:refnum<visa-resource-name>)
        n718 = call "conversion data to bits.vi"("Data input"=w1261, "Max supply"=sgl 30000.0) -> ("15 bits output"=w1256:u16)  [unwired: 1 in, 1 out]
        n719 = call "conversion data to bits.vi"("Data input"=w1258, "Max supply"=sgl 12000.0) -> ("15 bits output"=w1255:u16)  [unwired: 1 in, 1 out]
        n720 = call "conversion data to bits.vi"("Data input"=w1257, "Max supply"=sgl 2000.0) -> ("15 bits output"=w1254:u16)  [unwired: 1 in, 1 out]
        n721 = Number To Hexadecimal String(2:w1256) -> (0:w1253:string)  [unwired: 1 in]
        n722 = Number To Hexadecimal String(2:w1255) -> (0:w1250:string)  [unwired: 1 in]
        n723 = Number To Hexadecimal String(2:w1254) -> (0:w1249:string)  [unwired: 1 in]
        n724 = local read "APPEND"() -> (w1237:string)
        n725 = Concatenate Strings("XX  ", w1253, w1237) -> (w1248:string)
        n726 = Concatenate Strings("XX  ", w1250, w1237) -> (w1247:string)
        n727 = local write "PROCESS"(w1239) -> ()
        n728 = Concatenate Strings("XX ", w1249, w1237) -> (w1246:string)
        n729 = Build Array (concatenate)(w1240, w1239) -> (w1238:string[])
        n730 = Build Array(w1248, w1247, w1246) -> (w1242:string[])
        n731 = for {
          tunnel: w1242 -> [w1278] mode=indexing
          shift-right: [w1277] -> w1244
          shift-left: w1243 -> [w1279]
          shift-right: [w1267] -> w1235
          shift-left: w1241 -> [w1268]
          n732 = VISA Write(VISA resource name=w1279, write buffer=w1278) -> (VISA resource name out=w1274:refnum<visa-resource-name>, error out=w1273:errorcluster)  [unwired: 1 in, 1 out]
          n733 = flat-sequence {
            tunnel: w1274 -> [w1280]
            tunnel: [w1282] -> w1271
            tunnel: w1273 -> [w1282]
            tunnel: [w1280] -> w1272
            frame #0 {
              n734 = Wait (ms)(milliseconds to wait=u32 100) -> ()  [unwired: 1 out]
            }
          }
          n735 = property class="Instr"(reference=w1272, error in=w1271) -> (reference out=w1276:refnum<visa-resource-name>, error out=w1270:errorcluster, "Serial Settings:Number of Bytes at Serial Port"=w1275:u32)
          n736 = VISA Read(VISA resource name=w1276, byte count=w1275, error in (no error)=w1270) -> (VISA resource name out=w1277:refnum<visa-resource-name>, read buffer=w1269:string)  [unwired: 2 out]
          n737 = Build Array (concatenate)(w1268, w1269) -> (w1267:string[])
          n738 = local write "SERIAL \nRESPONSE"(w1267) -> ()
        }
        n739 = local write "PROCESSES"(w1238) -> ()
        n740 = local write "ORSAY"(w1244) -> ()
      }
      frame "SAVE SETTINGS" {
        n741 = stacked-sequence {
          seq-local: [w1290 _] -> [_ w1395]
          seq-local: [w1289 _] -> [_ w1394]
          frame #0 {
            w1324 = "FIB SETTINGS" ("channel name")
            n742 = local read "STIGMATOR"() -> (w1288:T12)
            n743 = local read "ION GUN SETTINGS"() -> (w1367:T1)
            n744 = local read "STIGMATOR X & Y"() -> (w1350:cluster{"X":sgl, "Y":sgl})
            n745 = local read "CONDENSOR"() -> (w1351:cluster{"COARSE":sgl[unit], "FINE":sgl[unit]})
            n746 = local read "OBJECTIVE"() -> (w1352:cluster{"COARSE":sgl[unit], "FINE":sgl[unit]})
            n747 = Unbundle By Name(w1288) -> ("STIG ALIGN"=w1287:cluster{"+X":sgl, "-X":sgl, "+Y":sgl, "-Y":sgl})
            n748 = local read "COLUMN VACUUM"() -> (w1293:dbl[unit])
            n749 = Unbundle By Name(w1367) -> ("BEAM ENERGY"=w1345:sgl[unit], "EXTRACTOR"=w1321:sgl[unit], "SUPPRESSOR"=w1320:sgl[unit], "ION CURRENT"=w1319:sgl[unit])
            n750 = Unbundle By Name(w1352) -> ("COARSE"=w1344:sgl[unit], "FINE"=w1337:sgl[unit])
            n751 = local read "BEAM CURRENT (FC1)"() -> (w1294:dbl[unit])
            n752 = Unbundle By Name(w1351) -> ("COARSE"=w1336:sgl[unit], "FINE"=w1335:sgl[unit])
            n753 = Unbundle By Name(w1350) -> ("X"=w1334:sgl, "Y"=w1333:sgl)
            n754 = Unbundle By Name(w1287) -> ("+X"=w1303:sgl, "-X"=w1302:sgl, "+Y"=w1301:sgl, "-Y"=w1300:sgl)
            n755 = To Variant(anything=w1303) -> (Variant=w1299:variant)
            n756 = To Variant(anything=w1302) -> (Variant=w1298:variant)
            n757 = To Variant(anything=w1301) -> (Variant=w1297:variant)
            n758 = To Variant(anything=w1300) -> (Variant=w1296:variant)
            n759 = call "File Dialog"() -> ("selected path"=w1369:path, "error out"=w1348:errorcluster)  [unwired: 12 in, 2 out]
            n760 = node(w1336) -> (w1313:sgl)
            n761 = node(w1335) -> (w1312:sgl)
            n762 = node(w1345) -> (w1322:sgl)
            n763 = node(w1321) -> (w1316:sgl)
            n764 = node(w1320) -> (w1317:sgl)
            n765 = node(w1319) -> (w1318:sgl)
            n766 = node(w1344) -> (w1315:sgl)
            n767 = node(w1337) -> (w1314:sgl)
            n768 = TDMS Open(8:w1348, 10:T23."create or replace" ("operation (0:open)"), 11:w1369) -> (0:w1347:errorcluster, 3:w1349:refnum<k34>)  [unwired: 4 in]
            n769 = To Variant(anything=w1322) -> (Variant=w1343:variant)
            n770 = To Variant(anything=w1316) -> (Variant=w1342:variant)
            n771 = To Variant(anything=w1317) -> (Variant=w1341:variant)
            n772 = node(w1294) -> (w1286:dbl)
            n773 = To Variant(anything=w1318) -> (Variant=w1340:variant)
            n774 = To Variant(anything=w1315) -> (Variant=w1339:variant)
            n775 = To Variant(anything=w1314) -> (Variant=w1332:variant)
            n776 = To Variant(anything=w1313) -> (Variant=w1331:variant)
            n777 = To Variant(anything=w1312) -> (Variant=w1330:variant)
            n778 = To Variant(anything=w1334) -> (Variant=w1329:variant)
            n779 = To Variant(anything=w1333) -> (Variant=w1328:variant)
            n780 = node(w1293) -> (w1292:dbl)
            n781 = To Variant(anything=w1286) -> (Variant=w1295:variant)
            n782 = To Variant(anything=w1292) -> (Variant=w1291:variant)
            n783 = local read "SCANNING CLUSTER"() -> (w1311:T14)
            n784 = Build Array(w1343, w1342, w1341, w1340, w1339, w1332, w1331, w1330, w1329, w1328, w1299, w1298, w1297, w1296, w1295, w1291) -> (w1338:variant[])
            n785 = for {
              tunnel: T22 ["BEAM ENERGY", "EXTRACTOR", "SUPRESSOR", "ION CURRENT", "OBJ COARSE", "OBJ FINE", "COND COARSE", "COND FINE", "STIGX", "STIGY", "STIG+X", "STIG-X", "STIG+Y", "STIG-Y", "PROBE CURRENT", "COLUMN VACUUM"] -> [w1385] mode=indexing
              shift-right: [w1387] -> w1323
              shift-left: w1347 -> [w1383]
              tunnel: w1338 -> [w1381] mode=indexing
              tunnel: w1324 -> [w1380]
              tunnel: "ORSAY COLUMN" -> [w1379]
              shift-right: [w1386] -> w1326
              shift-left: w1349 -> [w1388]
              n786 = call <userlib>:"Set Data Name__ogtk.vi"("error in (no error)"=w1383, "Data Name"=w1385, "Data"=w1381) -> ("error out"=w1382:errorcluster, "Renamed Data"=w1384:variant)  [unwired: 7 in]
              n787 = TDMS Set Properties(5:w1384, 7:w1385, 8:w1382, 9:w1379, 10:w1380, 11:w1388) -> (0:w1387:errorcluster, 3:w1386:refnum<k34>)  [unwired: 2 out]
            }
            n788 = Get Date/Time String() -> (date string=w1355:string, time string=w1356:string)  [unwired: 3 in]
            n789 = Unbundle By Name(w1311) -> ("X-OFFSET"=w1307:sgl[unit], "Y-OFFSET"=w1306:sgl[unit], "ROTATION"=w1305:dbl[unit], "MAGNIFICATION"=w1304:dbl)  [unwired: 1 out]
            n790 = To Variant(anything=0) -> (Variant=w1357:variant)
            n791 = To Variant(anything="NAME") -> (Variant=w1360:variant)
            n792 = To Variant(anything="USER") -> (Variant=w1361:variant)
            n793 = To Variant(anything=w1355) -> (Variant=w1362:variant)
            n794 = To Variant(anything=w1356) -> (Variant=w1363:variant)
            n795 = To Variant(anything="COMMENT") -> (Variant=w1365:variant)
            n796 = Build Array(w1357, w1360, w1361, w1362, w1363, w1365) -> (w1366:variant[])
            n797 = for {
              shift-right: [w1377] -> w1289
              shift-left: w1323 -> [w1375]
              tunnel: string[] ["RUN ID", "USER ID", "DATE", "TIME", "COMMENTS"] ("property names") -> [w1372] mode=indexing
              tunnel: "RUN DETAILS" ("channel name") -> [w1373]
              tunnel: w1366 -> [w1371] mode=indexing
              tunnel: w1324 -> [w1370]
              shift-right: [w1376] -> w1290
              shift-left: w1326 -> [w1378]
              n798 = call <userlib>:"Set Data Name__ogtk.vi"("Data Name"=w1372, "Data"=w1371) -> ("Renamed Data"=w1374:variant)  [unwired: 8 in, 1 out]
              n799 = TDMS Set Properties(5:w1374, 7:w1372, 8:w1375, 9:w1373, 10:w1370, 11:w1378) -> (0:w1377:errorcluster, 3:w1376:refnum<k34>)  [unwired: 2 out]
            }
            n800 = node(w1307) -> (w1310:sgl)
            n801 = node(w1306) -> (w1308:sgl)
            n802 = node(w1305) -> (w1309:dbl)
            n803 = To Variant(anything=w1310) -> ()  [unwired: 1 out]
            n804 = To Variant(anything=w1308) -> ()  [unwired: 1 out]
            n805 = To Variant(anything=w1309) -> ()  [unwired: 1 out]
            n806 = To Variant(anything=w1304) -> ()  [unwired: 1 out]
          }
          frame #1 {
            n807 = local read "OBJECT APERTURE POSITIONS"() -> (w1389:cluster{"NAME":string, "Xo":dbl, "Yo":dbl}[])
            n808 = for {
              tunnel: "APERTURE SETTINGS" ("channel name") -> [w1418]
              tunnel: "FIB SETTINGS" ("channel name") -> [w1417]
              shift-right: [w1414] -> w1393
              shift-left: w1395 -> [w1416]
              shift-right: [w1413] -> w1392
              shift-left: w1394 -> [w1415]
              tunnel: w1389 -> [w1410] mode=indexing
              tunnel: "X" -> [w1408]
              tunnel: "Y" -> [w1406]
              i -> [w1412]
              n809 = Unbundle By Name(w1410) -> ("NAME"=w1409:string, "Xo"=w1402:dbl, "Yo"=w1401:dbl)
              n810 = Number To Decimal String(number=w1412, width (-)=i16 0) -> (decimal integer string=w1407:string)
              n811 = Concatenate Strings(w1409, w1407, w1408) -> (w1405:string)
              n812 = Concatenate Strings(w1409, w1407, w1406) -> (w1404:string)
              n813 = To Variant(anything=w1402) -> (Variant=w1400:variant)
              n814 = To Variant(anything=w1401) -> (Variant=w1399:variant)
              n815 = Build Array(w1405, w1404) -> (w1403:string[])
              n816 = Build Array(w1400, w1399) -> (w1398:variant[])
              n817 = for {
                shift-right: [w1426] -> w1413
                shift-left: w1415 -> [w1424]
                tunnel: w1403 -> [w1421] mode=indexing
                tunnel: w1418 -> [w1422]
                tunnel: w1417 -> [w1420]
                shift-right: [w1425] -> w1414
                shift-left: w1416 -> [w1427]
                tunnel: w1398 -> [w1419] mode=indexing
                n818 = call <userlib>:"Set Data Name__ogtk.vi"("Data Name"=w1421, "Data"=w1419) -> ("Renamed Data"=w1423:variant)  [unwired: 8 in, 1 out]
                n819 = TDMS Set Properties(5:w1423, 7:w1421, 8:w1424, 9:w1422, 10:w1420, 11:w1427) -> (0:w1426:errorcluster, 3:w1425:refnum<k34>)  [unwired: 2 out]
              }
            }
            n820 = TDMS Close(8:w1392, 11:w1393) -> ()  [unwired: 2 out]
          }
        }
      }
      frame "READ SETTINGS" {
        (unwired) 2 ("index")
        (unwired) 1 ("index")
        w1475 = "FIB SETTINGS" ("group name")
        (unwired) string[] ["BEAM ENERGY", "EXTRACTOR", "SUPRESSOR", "ION CURRENT", "OBJ COARSE", "OBJ FINE", "COND COARSE", "COND FINE", "STIGX", "STIGY", "SCAN TYPE", "X-OFFSET", "Y-OFFSET", "ROTATION", "MAGNIFICATION", "STIG+X", "STIG-X", "STIG+Y", "STIG-Y", "PROBE CURRENT", "COLUMN VACUUM"]
        n821 = TDMS Open(11:"FIB SETUP FILE") -> (0:w1480:errorcluster, 3:w1479:refnum<k34>)  [unwired: 6 in]
        n822 = TDMS List Contents(4:w1480, 6:w1475, 7:w1479) -> (1:w1474:string[], 3:w1478:refnum<k34>)  [unwired: 2 out]
        n823 = Index Array(array=w1474, index=0) -> (element=w1472:string)
        n824 = TDMS Get Properties(9:w1472, 10:w1475, 11:w1478) -> (0:w1476:errorcluster, 3:w1477:refnum<k34>, 4:w1434:variant[])  [unwired: 3 in, 3 out]
        n825 = Delete From Array(array=w1434, length=1, index=0) -> (array with subset deleted=w1431:variant[])  [unwired: 1 out]
        n826 = for {
          tunnel: w1431 -> [w1484] mode=indexing
          tunnel: [w1483] -> w1469 mode=indexing
          n827 = Variant To Data(type=sgl 0.0, Variant=w1484) -> (data=w1483:sgl)  [unwired: 1 in, 1 out]
        }
        n828 = TDMS Close(8:w1476, 11:w1477) -> ()  [unwired: 2 out]
        n829 = Index Array(array=w1469, index #1=0 ("index"), index #2=1 ("index"), index #3=2 ("index"), index #4=3 ("index"), index #5=4 ("index"), index #6=5 ("index"), index #7=6 ("index"), index #8=7 ("index"), index #9=8 ("index"), index #10=9 ("index")) -> (element #1=w1468:sgl, element #2=w1467:sgl, element #3=w1466:sgl, element #4=w1465:sgl, element #5=w1452:sgl, element #6=w1451:sgl, element #7=w1450:sgl, element #8=w1449:sgl, element #9=w1436:sgl, element #10=w1435:sgl)  [unwired: 4 in, 4 out]
        n830 = node(w1468) -> (w1464:sgl[unit])
        n831 = node(w1467) -> (w1463:sgl[unit])
        n832 = node(w1466) -> (w1462:sgl[unit])
        n833 = node(w1465) -> (w1461:sgl[unit])
        n834 = node(w1452) -> (w1460:sgl[unit])
        n835 = node(w1451) -> (w1459:sgl[unit])
        n836 = node(w1450) -> (w1458:sgl[unit])
        n837 = node(w1449) -> (w1457:sgl[unit])
        n838 = local read "STIGMATOR X & Y"() -> (w1438:cluster{"X":sgl, "Y":sgl})
        n839 = local read "ION GUN SETTINGS"() -> (w1471:T1)
        n840 = Bundle By Name(cluster=w1471, "BEAM ENERGY"=w1464, "EXTRACTOR"=w1463, "SUPPRESSOR"=w1462, "ION CURRENT"=w1461) -> (w1470:T1)
        n841 = local read "CONDENSOR"() -> (w1455:cluster{"COARSE":sgl[unit], "FINE":sgl[unit]})
        n842 = Bundle By Name(cluster=w1455, "COARSE"=w1458, "FINE"=w1457) -> (w1454:cluster{"COARSE":sgl[unit], "FINE":sgl[unit]})
        n843 = local read "OBJECTIVE"() -> (w1456:cluster{"COARSE":sgl[unit], "FINE":sgl[unit]})
        n844 = Bundle By Name(cluster=w1456, "COARSE"=w1460, "FINE"=w1459) -> (w1453:cluster{"COARSE":sgl[unit], "FINE":sgl[unit]})
        n845 = Bundle By Name(cluster=w1438, "X"=w1436, "Y"=w1435) -> (w1437:cluster{"X":sgl, "Y":sgl})
        n846 = local write "STIGMATOR X & Y"(w1437) -> ()
        n847 = local write "OBJECTIVE"(w1453) -> ()
        n848 = local write "CONDENSOR"(w1454) -> ()
        n849 = local write "ION GUN SETTINGS"(w1470) -> ()
      }
      frame "BLANKING TOGGLE" {
        w1491 = "BLANKING MODE" ("PROCESS")
        n850 = local read "BEAM ON"() -> (w1492:bool)
        n851 = case shown="False" w1492 {
          tunnel: [w1494 w1516] -> w1489
          frame False {
            n852 = local read "APPEND"() -> (w1493:string)
            n853 = local read "VISA ERROR"() -> (w1505:errorcluster)
            n854 = Concatenate Strings("BL 0,1", "," ("string"), "0" ("string"), w1493) -> (w1495:string)
            n855 = local read "ORSAY"() -> (w1506:refnum<visa-resource-name>)
            n856 = VISA Write(VISA resource name=w1506, write buffer=w1495, error in (no error)=w1505) -> (VISA resource name out=w1502:refnum<visa-resource-name>, error out=w1500:errorcluster)  [unwired: 1 out]
            n857 = flat-sequence {
              tunnel: [w1512] -> w1501
              tunnel: w1502 -> [w1512]
              tunnel: [w1511] -> w1499
              tunnel: w1500 -> [w1511]
              frame #0 {
                n858 = Wait (ms)(milliseconds to wait=u32 100) -> ()  [unwired: 1 out]
              }
            }
            n859 = property class="Instr"(reference=w1501, error in=w1499) -> (reference out=w1509:refnum<visa-resource-name>, error out=w1507:errorcluster, "Serial Settings:Number of Bytes at Serial Port"=w1508:u32)
            n860 = VISA Read(VISA resource name=w1509, byte count=w1508, error in (no error)=w1507) -> (VISA resource name out=w1504:refnum<visa-resource-name>, read buffer=w1494:string, error out=w1503:errorcluster)  [unwired: 1 out]
            n861 = local write "VISA ERROR"(w1503) -> ()
            n862 = local write "ORSAY"(w1504) -> ()
          }
          frame True {
            n863 = local read "BLANKING CONTROL"() -> (w1517:u16)
            n864 = local read "APPEND"() -> (w1513:string)
            n865 = Pick Line(multi-line string="BL 0,0\nBL 1,1\nBL 2,0", line index=w1517) -> (output string=w1522:string)  [unwired: 1 in]
            n866 = Concatenate Strings(w1522, w1513) -> (w1515:string)
            n867 = local read "VISA ERROR"() -> (w1525:errorcluster)
            n868 = local read "ORSAY"() -> (w1526:refnum<visa-resource-name>)
            n869 = VISA Write(VISA resource name=w1526, write buffer=w1515, error in (no error)=w1525) -> (VISA resource name out=w1521:refnum<visa-resource-name>, error out=w1519:errorcluster)  [unwired: 1 out]
            n870 = flat-sequence {
              tunnel: [w1532] -> w1520
              tunnel: w1521 -> [w1532]
              tunnel: [w1531] -> w1518
              tunnel: w1519 -> [w1531]
              frame #0 {
                n871 = Wait (ms)(milliseconds to wait=u32 100) -> ()  [unwired: 1 out]
              }
            }
            n872 = property class="Instr"(reference=w1520, error in=w1518) -> (reference out=w1529:refnum<visa-resource-name>, error out=w1527:errorcluster, "Serial Settings:Number of Bytes at Serial Port"=w1528:u32)
            n873 = VISA Read(VISA resource name=w1529, byte count=w1528, error in (no error)=w1527) -> (VISA resource name out=w1524:refnum<visa-resource-name>, read buffer=w1516:string, error out=w1523:errorcluster)  [unwired: 1 out]
            n874 = local write "ORSAY"(w1524) -> ()
            n875 = local write "VISA ERROR"(w1523) -> ()
          }
        }
        n876 = Build Array (concatenate)(w1490, w1491) -> (w1487:string[])
        n877 = local write "PROCESS"(w1491) -> ()
        n878 = Build Array (concatenate)(w1488, w1489) -> (w1485:string[])
        n879 = local write "SERIAL \nRESPONSE"(w1485) -> ()
        n880 = local write "PROCESSES"(w1487) -> ()
      }
      frame "SET STIGMATOR" {
        w1536 = "ADJUSTING STIGMATOR" ("PROCESS")
        n881 = local read "VISA ERROR"() -> (w1542:errorcluster)
        n882 = local read "ORSAY"() -> (w1549:refnum<visa-resource-name>)
        n883 = call "CENTER STIGMATOR.vi"("STIGMATOR"="STIGMATOR") -> ("STIGMATOR COMMAND"=w1543:string)  [unwired: 5 in]
        n884 = VISA Write(VISA resource name=w1549, write buffer=w1543, error in (no error)=w1542) -> (VISA resource name out=w1544:refnum<visa-resource-name>, error out=w1546:errorcluster)  [unwired: 1 out]
        n885 = property class="Instr"(reference=w1544, error in=w1546) -> (reference out=w1545:refnum<visa-resource-name>, error out=w1547:errorcluster, "Serial Settings:Number of Bytes at Serial Port"=w1548:u32)
        n886 = local write "PROCESS"(w1536) -> ()
        n887 = Build Array (concatenate)(w1537, w1536) -> (w1535:string[])
        n888 = VISA Read(VISA resource name=w1545, byte count=w1548, error in (no error)=w1547) -> (VISA resource name out=w1541:refnum<visa-resource-name>, read buffer=w1539:string, error out=w1540:errorcluster)  [unwired: 1 out]
        n889 = local write "PROCESSES"(w1535) -> ()
        n890 = local write "ORSAY"(w1541) -> ()
        n891 = local write "VISA ERROR"(w1540) -> ()
        n892 = Build Array (concatenate)(w1538, w1539) -> (w1533:string[])
        n893 = local write "SERIAL \nRESPONSE"(w1533) -> ()
      }
      frame "SET WOBBLER FOR OBJECT" {
        n894 = local read "WOBBLER SETTINBGS FOR OBJECT ALIGNMENT"() -> (w1554:T10)
        n895 = Unbundle By Name(w1554) -> ()  [unwired: 2 out]
      }
      frame "DEFINE NEW OBJ" {
        n896 = local read "OBJECT APERTURE POSITIONS"() -> (w1565:cluster{"NAME":string, "Xo":dbl, "Yo":dbl}[])
        n897 = property on="OBJECT APERTURE" class="Ring (strict)"() -> ("RingText.Text"=w1563:string)  [unwired: 2 in, 2 out]
        n898 = local read "Xo"() -> (w1562:dbl)
        n899 = local read "Yo"() -> (w1561:dbl)
        n900 = Index Array(array=w1565, index=0) -> (element=w1564:cluster{"NAME":string, "Xo":dbl, "Yo":dbl})
        n901 = Bundle By Name(cluster=w1564, "NAME"=w1563, "Xo"=w1562, "Yo"=w1561) -> (w1560:cluster{"NAME":string, "Xo":dbl, "Yo":dbl})
        n902 = local read "OBJECT APERTURE"() -> (w1566:u16)
        n903 = Replace Array Subset(array=w1565, new element=w1560, index=w1566) -> (w1559:cluster{"NAME":string, "Xo":dbl, "Yo":dbl}[])
        n904 = local write "OBJECT APERTURE POSITIONS"(w1559) -> ()
      }
      frame "DEFINE NEW APERTURE" {
        n905 = local read "MASS APERTURE POSITIONS"() -> (w1577:cluster{"NAME":string, "Xa":dbl, "Ya":dbl}[])
        n906 = property on="APERTURE (MASS)" class="Ring (strict)"() -> ("RingText.Text"=w1570:string)  [unwired: 2 in, 2 out]
        n907 = local read "Xa"() -> (w1575:dbl)
        n908 = local read "Ya"() -> (w1574:dbl)
        n909 = Index Array(array=w1577, index=0) -> (element=w1576:cluster{"NAME":string, "Xa":dbl, "Ya":dbl})
        n910 = Bundle By Name(cluster=w1576, "NAME"=w1570, "Xa"=w1575, "Ya"=w1574) -> (w1573:cluster{"NAME":string, "Xa":dbl, "Ya":dbl})
        n911 = local read "APERTURE (MASS)"() -> (w1578:u16)
        n912 = Replace Array Subset(array=w1577, new element=w1573, index=w1578) -> (w1572:cluster{"NAME":string, "Xa":dbl, "Ya":dbl}[])
        n913 = local write "MASS APERTURE POSITIONS"(w1572) -> ()
      }
      frame "INITIALISE PI MOTORS" {
        n914 = local read "ENABLE APERTURES"() -> (w1579:bool)
        n915 = case shown="True" w1579 {
          frame False {
          }
          frame True {
            # "Stage names input"
            # "TRUE: All axes can be moved"
            n916 = local read "STAGE AXES"() -> (w1588:string[])
            n917 = local write "INIT PI"(FALSE ("INIT PI")) -> ()
            n918 = call "C843_Configuration_Setup.vi"("System no."=1, "C-843 Board No."=1, "Axes to move"=w1588, "All axes?"=TRUE, "C-843 version"=TRUE, "Use dialog to define\nconnected stages?"=FALSE ("Use dialog to define\nconnected stages?"), "Stage names input"=string[] ["FIBSTAGE", "FIBSTAGE", "FIBSTAGE", "FIBSTAGE"], "Limit switch selection"="HOME ON LIMIT", "RON Affected axes"=w1588, "Reference mode"=bool[] [TRUE, TRUE, TRUE, TRUE]) -> ("Identification"=w1594:string, "Position"=→"POSITIONS":dbl[], "+/- movement\nrange"=→"RANGE":dbl[], "error out"=w1592:errorcluster)  [unwired: 5 in, 1 out]
            n919 = Select(t="NONE", s=w1592, f=w1594) -> (s? t:f=w1593:string)
            n920 = Unbundle By Name(w1592) -> ("status"=→"NO CONTROLLER":bool)
            n921 = Concatenate Strings("DETECTED CONTROLLER:", w1593) -> (w1596:string)
            n922 = local write "PROCESS"(w1596) -> ()
          }
        }
      }
      frame "READ APERTURE POSITIONS" {
        w1605 = FALSE ("All axes?")
        w1604 = 1 ("System no.")
        n923 = local read "STAGE AXES"() -> (w1606:string[])
        n924 = call "FRF?.vi"("System no."=w1604, "Axes to query"=w1606, "All axes?"=w1605) -> ("Referenced?"=w1602:bool[], "error out"=w1609:errorcluster)  [unwired: 2 in, 13 out]
        n925 = call "POS?.vi"("System no."=w1604, "Axes to query"=w1606, "All axes?"=w1605, "error in"=w1609) -> ("Position"=w1607:dbl[], "error out"=w1608:errorcluster)  [unwired: 1 in, 13 out]
        n926 = Build Array (concatenate)(w1612, "READING APERTURES") -> (w1611:string[])
        n927 = local write "REFERENCED"(w1602) -> ()
        n928 = local write "POSITIONS"(w1607) -> ()
        n929 = Build Array (concatenate)(w1615, "") -> (w1614:string[])
        n930 = call "RON?.vi"("System no."=w1604, "Axes to query"=w1606, "All axes?"=w1605, "error in"=w1608) -> ("Reference on?"=w1603:bool[])  [unwired: 1 in, 14 out]
        n931 = local write "ON TRARGET"(w1603) -> ()
      }
      frame "HOME OBJ & AP STAGES" {
      }
      frame "SET OBJ & AP STAGE VELOCITIES" {
        w1625 = string[] ["Xo", "Yo", "Xa", "Ya"] ("Axes to move")
        # "um/s"
        n932 = call "VEL.vi"("System no."=1, "Axes to set"=w1625, "Velocity values"=dbl[] [1000.0, 1000.0, 1000.0, 1000.0], "No.of digits"=i16 4, "Without axis ID?"=FALSE) -> ("error out"=w1627:errorcluster)  [unwired: 1 in, 13 out]
        n933 = call "VEL?.vi"("System no."=1, "Axes to query"=w1625, "All axes?"=TRUE, "error in"=w1627) -> ("Velocity"=→"VELOCITIES":dbl[])  [unwired: 1 in, 14 out]
        n934 = local write "PROCESS"("SETTING OBJ & APERTURE VELOCITIES" ("channel name")) -> ()
      }
      frame "MOVE OBJ STAGES" {
        w1638 = string[] ["Xo", "Yo"] ("Axes to move")
        n935 = local read "OBJECT APERTURE POSITIONS"() -> (w1650:cluster{"NAME":string, "Xo":dbl, "Yo":dbl}[])
        n936 = local read "OBJECT APERTURE"() -> (w1649:u16)
        n937 = Index Array(array=w1650, index=w1649) -> (element=w1648:cluster{"NAME":string, "Xo":dbl, "Yo":dbl})
        n938 = Unbundle By Name(w1648) -> ("Xo"=w1647:dbl, "Yo"=w1646:dbl)
        n939 = Build Array(w1647, w1646) -> (w1645:dbl[])
        n940 = call "MOV.vi"("System no."=1, "Axes to move"=w1638, "Position values"=w1645) -> ("error out"=w1651:errorcluster)  [unwired: 2 in, 14 out]
        n941 = call "MOV?.vi"("System no."=1, "Axes to query"=w1638, "All axes?"=TRUE, "error in"=w1651) -> ("Target position"=w1644:dbl[])  [unwired: 1 in, 14 out]
        n942 = Index Array(array=w1644, index #1=0 ("index"), index #2=1 ("index")) -> (element #1=w1643:dbl, element #2=w1642:dbl)
        n943 = local write "Xo"(w1643) -> ()
        n944 = local write "Yo"(w1642) -> ()
      }
      frame "MOVE APERTURE STAGES" {
        w1653 = string[] ["1", "2"] ("Axes to move")
        w1652 = 1 ("System no.")
        n945 = local read "MASS APERTURE POSITIONS"() -> (w1661:cluster{"NAME":string, "Xa":dbl, "Ya":dbl}[])
        n946 = local read "APERTURE (MASS)"() -> (w1660:u16)
        n947 = Index Array(array=w1661, index=w1660) -> (element=w1669:cluster{"NAME":string, "Xa":dbl, "Ya":dbl})
        n948 = Unbundle By Name(w1669) -> ("Xa"=w1668:dbl, "Ya"=w1667:dbl)
        n949 = Build Array(w1668, w1667) -> (w1666:dbl[])
        n950 = call "MOV.vi"("System no."=w1652, "Axes to move"=w1653, "Position values"=w1666) -> ("error out"=w1670:errorcluster)  [unwired: 2 in, 14 out]
        n951 = call "MOV?.vi"("System no."=w1652, "Axes to query"=w1653, "All axes?"=TRUE, "error in"=w1670) -> ("Target position"=w1665:dbl[], "error out"=w1654:errorcluster)  [unwired: 1 in, 13 out]
        n952 = while {
          tunnel: w1653 -> [w1672]
          tunnel: w1652 -> [w1675]
          shift-right: [w1671] -> _
          shift-left: w1654 -> [w1676]
          stop <- w1679 stop-if-true
          w1673 = FALSE ("All axes?")
          n953 = call "POS?.vi"("System no."=w1675, "Axes to query"=w1672, "All axes?"=w1673, "error in"=w1676) -> ("error out"=w1674:errorcluster)  [unwired: 1 in, 14 out]
          n954 = call "ONT?.vi"("System no."=w1675, "Axes to query"=w1672, "All axes?"=w1673, "error in"=w1674) -> ("Axis on target?"=w1678:bool[], "error out"=w1671:errorcluster)  [unwired: 1 in, 13 out]
          "ON TRARGET" <- w1678
          n955 = Index Array(array=w1678, index #1=0 ("index"), index #2=1 ("index")) -> (element #1=w1680:bool, element #2=w1681:bool)
          n956 = Wait (ms)(milliseconds to wait=u32 100) -> ()  [unwired: 1 out]
          n957 = And(x=w1680, y=w1681) -> (x .and. y?=w1679:bool)
        }
        n958 = Index Array(array=w1665, index #1=0 ("index"), index #2=1 ("index")) -> (element #1=w1659:dbl, element #2=w1658:dbl)
        n959 = local write "Xa"(w1659) -> ()
        n960 = local write "Ya"(w1658) -> ()
      }
    }
  }
  n961 = while {
    shift-right: [w1685] -> _
    shift-left: w14 -> [w1687]
    stop <- TRUE continue-if-true
    n962 = Dequeue Element(queue=w1687) -> (queue out=w1685:refnum<queue>, element=w1686:enum16{"INIT DAQ", "STOP TASKS"})  [unwired: 2 in, 2 out]
    n963 = case shown="\"STOP TASKS\"" w1686 {
      frame "INIT DAQ", Default {
      }
      frame "STOP TASKS" {
      }
    }
  }
  n964 = while {
    shift-right: [w1689] -> _
    shift-left: w26 -> [w1692]
    stop <- w1690 stop-if-true
    n965 = Dequeue Element(queue=w1692) -> (queue out=w1689:refnum<queue>, element=w1691:T17)  [unwired: 2 in, 2 out]
    n966 = case shown="True" "ENABLE CAMERA" {
      tunnel: w1691 -> [_ w1693]
      frame False {
      }
      frame True {
        n967 = case shown="\"INIT VIDEO\"" w1693 {
          frame "LOOP", Default {
            n968 = local read "FIB SAMPLE CAMERA"() -> (w1695:T4)
            n969 = local read "FIB CAMERA ERROR"() -> (w1696:errorcluster)
            n970 = local read "FIB CAMERA"() -> (w1697:T5)
            n971 = property on="ANGLE" class="DigNum (strict)"("Visible"="ROTATE VIEW") -> ()  [unwired: 2 in, 2 out]
            n972 = call <vilib>:"IMAQdx Get Image2.vi"("Timeout (ms)"=500, "Buffer Number Mode (Next)"=IMAQdx_Buffer_Number_Mode."Last New", "error in"=w1696, "Image In"=w1697, "Session In"=w1695) -> ("error out"=w1707:errorcluster, "Image Out"=w1708:T5)  [unwired: 3 in, 2 out]
            n973 = case shown="True" "ROTATE VIEW" {
              tunnel: w1708 -> [w1722 w1726]
              tunnel: w1707 -> [w1721 w1725]
              tunnel: [w1721 w1724] -> w1702
              tunnel: [w1722 w1723] -> w1703
              frame False {
              }
              frame True {
                n974 = call "IMAQ Rotate"("error in (no error)"=w1725, "Angle (degrees)"="ANGLE", "Image Src"=w1726) -> ("error out"=w1724:errorcluster, "Image Dst Out"=w1723:T5)  [unwired: 7 in]
              }
            }
            n975 = case shown="False" "SYMMETRY" {
              tunnel: w1703 -> [w1729 w1734]
              tunnel: w1702 -> [w1728 w1733]
              tunnel: "IMAGE SYMMETRY" -> [_ w1732]
              tunnel: [w1729 w1731] -> w1709
              tunnel: [w1728 w1730] -> w1710
              frame False {
              }
              frame True {
                n976 = call "IMAQ Symmetry"("error in (no error)"=w1733, "Type of Symmetry"=w1732, "Image Src"=w1734) -> ("error out"=w1730:errorcluster, "Image Dst Out"=w1731:T5)  [unwired: 2 in]
              }
            }
            n977 = property on="BRIGHT,CONT,GAMMA" class="Clust (strict)"("Visible"="REFLECTIVITY") -> ()  [unwired: 2 in, 2 out]
            n978 = case shown="True" "REFLECTIVITY" {
              tunnel: w1709 -> [w1712 w1716]
              tunnel: [w1712 w1718] -> w1694
              tunnel: "BRIGHT,CONT,GAMMA" -> [_ w1717]
              tunnel: w1710 -> [w1711 w1715]
              tunnel: [w1711 w1713] -> _
              frame False {
              }
              frame True {
                w1720 = T29 0 items=["Grayscale (U8)", "Grayscale (I16)", "Grayscale (SGL)", "Complex (CSG)", "RGB (U32)", "HSL (U32)", "RGB (U64)", "Grayscale (U16)"] ("Image Type")
                n979 = call "IMAQ Cast Image"("Image Type"=w1720, "error in (no error)"=w1715, "Image Src"=w1716) -> ("error out"=w1714:errorcluster, "Image Dst Out"=w1719:T5)  [unwired: 7 in]
                n980 = call "IMAQ BCGLookup"("Image Src"=w1719, "BCG Values"=w1717, "error in (no error)"=w1714) -> ("Image Dst Out"=w1718:T5, "error out"=w1713:errorcluster)  [unwired: 4 in]
              }
            }
            n981 = local write "FIB CAMERA"(w1694) -> ()
          }
          frame "INIT VIDEO" {
            w1741 = T29 4 items=["Grayscale (U8)", "Grayscale (I16)", "Grayscale (SGL)", "Complex (CSG)", "RGB (U32)", "HSL (U32)", "RGB (U64)", "Grayscale (U16)"] ("Image Type")
            w1744 = 2.0
            w1772 = 2.0
            w1771 = sgl 0.95 ("x")
            n982 = call <vilib>:"IMAQdx Open Camera.vi"("Camera Control Mode"=IMAQdx_Camera_Control_Mode."Controller", "Session In"=T4 "MAKO") -> ("error out"=w1769:errorcluster, "Session Out"=w1770:T4)  [unwired: 8 in]
            n983 = call <vilib>:"IMAQdx Enumerate Attributes.vi"("error in"=w1769, "Session In"=w1770) -> ("error out"=w1765:errorcluster, "Session Out"=w1766:T4)  [unwired: 7 in, 1 out]
            n984 = property class="IMAQdx"(reference=w1766, error in=w1765) -> (reference out=w1764:T4, error out=w1763:errorcluster, "ActualPeakBandwidth"=→"ActualPeakBandwidth":dbl)
            n985 = property class="IMAQdx"(reference=w1764, error in=w1763) -> (reference out=w1738:T4, error out=w1737:errorcluster, "IPAddress"=→"IP ADDRESS":string, "Width"=w1736:u32, "Height"=w1735:u32)
            "IMAGE XPIXELS" <- w1736
            "IMAGE YPIXELS" <- w1735
            n986 = Multiply(x=w1736, y=w1771) -> (x*y=w1775:sgl)
            n987 = Multiply(x=w1735, y=w1771) -> (x*y=w1774:sgl)
            n988 = To Double Precision Float(number=w1736) -> (double precision float=w1777:dbl)
            n989 = To Double Precision Float(number=w1735) -> (double precision float=w1778:dbl)
            n990 = Bundle(w1775, w1774) -> ()  [unwired: 1 in, 1 out]
            n991 = Divide(x=w1778, y=w1772) -> (x/y=→"IMAGE YCENTRE":dbl)
            n992 = Divide(x=w1777, y=w1772) -> (x/y=→"IMAGE XCENTRE":dbl)
            n993 = call <vilib>:"IMAQdx Configure Grab.vi"("error in"=w1737, "Session In"=w1738) -> ("error out"=w1751:errorcluster, "Session Out"=w1752:T4)  [unwired: 8 in]
            n994 = case shown="False" FALSE {
              tunnel: w1752 -> [w1782 w1786]
              tunnel: [w1782 w1785] -> w1761
              tunnel: w1751 -> [w1781 w1784]
              tunnel: [w1781 w1783] -> w1762
              frame False {
              }
              frame True {
                n995 = call <vilib>:"IMAQdx Read Attributes.vi"("error in"=w1784, "Session In"=w1786) -> ("error out"=w1783:errorcluster, "Session Out"=w1785:T4)  [unwired: 8 in]
              }
            }
            n996 = Divide(x=w1736, y=w1744) -> (x/y=w1753:dbl)
            n997 = Divide(x=w1735, y=w1744) -> (x/y=w1754:dbl)
            n998 = To Long Integer(number=w1753) -> (32bit integer=w1755:i32)
            n999 = To Long Integer(number=w1754) -> (32bit integer=w1756:i32)
            n1000 = Subtract(x=w1755, y=3) -> (x-y=w1758:i32)
            n1001 = call <vilib>:"IMAQdx Start Acquisition.vi"("error in"=w1762, "Session In"=w1761) -> ("error out"=→"FIB CAMERA ERROR":errorcluster, "Session Out"=→"FIB SAMPLE CAMERA":T4)  [unwired: 8 in]
            n1002 = Subtract(x=w1756, y=2) -> (x-y=w1757:i32)
            n1003 = call "IMAQ Create"("Image Name"="TARGET", "Image Type"=w1741, "error in (no error)"=w1762) -> ("New Image"=w1749:T5, "error out"=w1760:errorcluster)  [unwired: 2 in]
            n1004 = Bundle(w1758, w1757) -> (w1759:cluster{i32, i32})  [unwired: 1 in]
            "CENTRE CAMERA FOV" <- w1759
            n1005 = call "IMAQ Overlay Bitmap"("Group"="FEATURES", "error in (no error)"=w1760, "Bitmap"=u32[][] [[16777216, 16777216, 16777216, 16777216, 16777216, 16777216, 16777216, 16777216, 16777216, 16777216, 16777216, 12189440, 16777216, 16777216, 16777216, 16777216, 16777216, 16777216, 16777216, 16777216, 16777216, 16777216, 16777216], [16777216, 16777216, 16777216, 16777216, 16777216, 16777216, 16777216, 16777216, 16777216, 16777216, 16777216, 12189440, 16777216, 16777216, 16777216, 16777216, 16777216, 16777216, 16777216, 16777216, 16777216, 16777216, 16777216], [16777216, 16777216, 16777216, 16777216, 16777216, 16777216, 16777216, 16777216, 16777216, 16777216, 15859456, 12189440, 15859456, 16777216, 16777216, 16777216, 16777216, 16777216, 16777216, 16777216, 16777216, 16777216, 16777216], [16777216, 16777216, 16777216, 16777216, 16777216, 16777216, 16777216, 16777216, 16777216, 16777216, 15859456, 12189440, 15859456, 16777216, 16777216, 16777216, 16777216, 16777216, 16777216, 16777216, 16777216, 16777216, 16777216], [16777216, 16777216, 16777216, 16777216, 16777216, 16777216, 16777216, 16777216, 16777216, 16777216, 15859456, 12189440, 15859456, 16777216, 16777216, 16777216, 16777216, 16777216, 16777216, 16777216, 16777216, 16777216, 16777216], [16777216, 16777216, 16777216, 16777216, 16777216, 16777216, 16777216, 16777216, 16777216, 16777216, 15859456, 12189440, 15859456, 16777216, 16777216, 16777216, 16777216, 16777216, 16777216, 16777216, 16777216, 16777216, 16777216], [16777216, 16777216, 16777216, 16777216, 16777216, 16777216, 16777216, 16777216, 16777216, 16777216, 15859456, 12189440, 15859456, 16777216, 16777216, 16777216, 16777216, 16777216, 16777216, 16777216, 16777216, 16777216, 16777216], [16777216, 16777216, 16777216, 16777216, 16777216, 16777216, 16777216, 16777216, 16777216, 16777216, 16777216, 12189440, 16777216, 16777216, 16777216, 16777216, 16777216, 16777216, 16777216, 16777216, 16777216, 16777216, 16777216], [16777216, 16777216, 16777216, 16777216, 16777216, 16777216, 16777216, 16777216, 12189440, 16777216, 16777216, 12189440, 16777216, 16777216, 12189440, 16777216, 16777216, 16777216, 16777216, 16777216, 16777216, 16777216, 16777216], [16777216, 16777216, 16777216, 16777216, 16777216, 16777216, 16777216, 16777216, 16777216, 12189440, 16777216, 12189440, 16777216, 12189440, 16777216, 16777216, 16777216, 16777216, 16777216, 16777216, 16777216, 16777216, 16777216], [16777216, 16777216, 15859456, 15859456, 15859456, 15859456, 15859456, 16777216, 16777216, 16777216, 16777216, 12189440, 16777216, 16777216, 16777216, 16777216, 15859456, 15859456, 15859456, 15859456, 15859456, 16777216, 16777216], [12189440, 12189440, 12189440, 12189440, 12189440, 12189440, 12189440, 12189440, 12189440, 12189440, 12189440, 12189440, 12189440, 12189440, 12189440, 12189440, 12189440, 12189440, 12189440, 12189440, 12189440, 12189440, 12189440], [16777216, 16777216, 15859456, 15859456, 15859456, 15859456, 15859456, 16777216, 16777216, 16777216, 16777216, 12189440, 16777216, 16777216, 16777216, 16777216, 15859456, 15859456, 15859456, 15859456, 15859456, 16777216, 16777216], [16777216, 16777216, 16777216, 16777216, 16777216, 16777216, 16777216, 16777216, 16777216, 12189440, 16777216, 12189440, 16777216, 12189440, 16777216, 16777216, 16777216, 16777216, 16777216, 16777216, 16777216, 16777216, 16777216], [16777216, 16777216, 16777216, 16777216, 16777216, 16777216, 16777216, 16777216, 12189440, 16777216, 16777216, 12189440, 16777216, 16777216, 12189440, 16777216, 16777216, 16777216, 16777216, 16777216, 16777216, 16777216, 16777216], [16777216, 16777216, 16777216, 16777216, 16777216, 16777216, 16777216, 16777216, 16777216, 16777216, 16777216, 12189440, 16777216, 16777216, 16777216, 16777216, 16777216, 16777216, 16777216, 16777216, 16777216, 16777216, 16777216], [16777216, 16777216, 16777216, 16777216, 16777216, 16777216, 16777216, 16777216, 16777216, 16777216, 15859456, 12189440, 15859456, 16777216, 16777216, 16777216, 16777216, 16777216, 16777216, 16777216, 16777216, 16777216, 16777216], [16777216, 16777216, 16777216, 16777216, 16777216, 16777216, 16777216, 16777216, 16777216, 16777216, 15859456, 12189440, 15859456, 16777216, 16777216, 16777216, 16777216, 16777216, 16777216, 16777216, 16777216, 16777216, 16777216], [16777216, 16777216, 16777216, 16777216, 16777216, 16777216, 16777216, 16777216, 16777216, 16777216, 15859456, 12189440, 15859456, 16777216, 16777216, 16777216, 16777216, 16777216, 16777216, 16777216, 16777216, 16777216, 16777216], [16777216, 16777216, 16777216, 16777216, 16777216, 16777216, 16777216, 16777216, 16777216, 16777216, 15859456, 12189440, 15859456, 16777216, 16777216, 16777216, 16777216, 16777216, 16777216, 16777216, 16777216, 16777216, 16777216], [16777216, 16777216, 16777216, 16777216, 16777216, 16777216, 16777216, 16777216, 16777216, 16777216, 15859456, 12189440, 15859456, 16777216, 16777216, 16777216, 16777216, 16777216, 16777216, 16777216, 16777216, 16777216, 16777216], [16777216, 16777216, 16777216, 16777216, 16777216, 16777216, 16777216, 16777216, 16777216, 16777216, 16777216, 12189440, 16777216, 16777216, 16777216, 16777216, 16777216, 16777216, 16777216, 16777216, 16777216, 16777216, 16777216], [16777216, 16777216, 16777216, 16777216, 16777216, 16777216, 16777216, 16777216, 16777216, 16777216, 16777216, 12189440, 16777216, 16777216, 16777216, 16777216, 16777216, 16777216, 16777216, 16777216, 16777216, 16777216, 16777216]], "Top Left Point"=w1759, "Image"=w1749) -> ("Image Out"=w1750:T5)  [unwired: 5 in, 1 out]
            n1006 = local write "FIB CAMERA"(w1750) -> ()
          }
          frame "CAMERA GAIN" {
            n1007 = local read "FIB SAMPLE CAMERA"() -> (w1789:T4)
            n1008 = local read "FIB CAMERA ERROR"() -> (w1788:errorcluster)
            n1009 = property class="IMAQdx"(reference=w1789, error in=w1788, "ActiveAttribute"="GainAuto") -> (reference out=w1796:T4, error out=w1797:errorcluster)
            n1010 = property class="IMAQdx"(reference=w1796, error in=w1797, "ValueU32"="GAIN METHOD") -> (reference out=w1798:T4, error out=w1799:errorcluster)
            n1011 = property class="IMAQdx"(reference=w1798, error in=w1799, "ActiveAttribute"="GainRaw") -> (reference out=w1793:T4, error out=w1794:errorcluster)
            n1012 = property class="IMAQdx"(reference=w1793, error in=w1794, "ValueDBL"="GAIN") -> (reference out=w1790:T4, error out=w1787:errorcluster)
            n1013 = local write "FIB SAMPLE CAMERA"(w1790) -> ()
            n1014 = local write "FIB CAMERA ERROR"(w1787) -> ()
          }
          frame "CAMERA EXPOSURE" {
            n1015 = local read "FIB SAMPLE CAMERA"() -> (w1804:T4)
            n1016 = local read "FIB CAMERA ERROR"() -> (w1803:errorcluster)
            n1017 = property class="IMAQdx"(reference=w1804, error in=w1803, "ActiveAttribute"="ExposureAuto") -> (reference out=w1808:T4, error out=w1807:errorcluster)
            n1018 = property class="IMAQdx"(reference=w1808, error in=w1807, "ValueU32"=u32 1) -> (reference out=w1817:T4, error out=w1818:errorcluster)
            n1019 = case shown="0, Default" "CONFIGS" {
              tunnel: [w1833 20.0 ("EXPOSURE TIME") 5.0 ("EXPOSURE TIME")] -> w1816
              tunnel: "EXPOSURE" -> [w1833 _ _]
              frame 0, Default {
              }
              frame 1 {
              }
              frame 2 {
              }
            }
            n1020 = local write "EXPOSURE"(w1816) -> ()
            n1021 = Multiply(x=1000.0, y=w1816) -> (x*y=w1819:dbl)
            n1022 = case shown="True" TRUE {
              tunnel: w1817 -> [w1824 w1831]
              tunnel: w1818 -> [w1823 w1830]
              tunnel: w1819 -> [_ w1827]
              tunnel: [w1824 w1826] -> w1806
              tunnel: [w1823 w1825] -> w1805
              frame False {
              }
              frame True {
                n1023 = property class="IMAQdx"(reference=w1831, error in=w1830, "ActiveAttribute"="ExposureTimeAbs") -> (reference out=w1829:T4, error out=w1828:errorcluster)
                n1024 = property class="IMAQdx"(reference=w1829, error in=w1828, "ValueDBL"=w1827) -> (reference out=w1826:T4, error out=w1825:errorcluster)
              }
            }
            n1025 = property class="IMAQdx"(reference=w1806, error in=w1805, "ActiveAttribute"="GainAuto") -> (reference out=w1820:T4, error out=w1821:errorcluster)
            n1026 = property class="IMAQdx"(reference=w1820, error in=w1821, "ValueU32"=u32 2) -> (reference out=w1802:T4, error out=w1801:errorcluster)
            n1027 = local write "FIB SAMPLE CAMERA"(w1802) -> ()
            n1028 = local write "FIB CAMERA ERROR"(w1801) -> ()
          }
        }
      }
    }
    n1029 = local read "STOP"() -> (w1690:bool)
  }
  n1030 = case shown="True" FALSE {
    frame False {
    }
    frame True {
      n1031 = call "MNL.vi"() -> ()  [unwired: 5 in, 15 out]
      n1032 = call "MPL.vi"() -> ()  [unwired: 5 in, 15 out]
      n1033 = call "VEL.vi"() -> ()  [unwired: 6 in, 14 out]
      n1034 = call "VEL?.vi"() -> ()  [unwired: 5 in, 15 out]
      n1035 = call "TMN?.vi"() -> ()  [unwired: 5 in, 15 out]
      n1036 = call "LIM?.vi"() -> ()  [unwired: 5 in, 15 out]
      n1037 = call "GOH.vi"() -> ()  [unwired: 5 in, 15 out]
      n1038 = call "TMX?.vi"() -> ()  [unwired: 5 in, 15 out]
    }
  }
